vi "单通道IT01.vi"() -> ()   [LabVIEW 2020]
uses:
  <vilib>/Utility/miscctls.llb/LVPointTypeDef.ctl
  <vilib>/Utility/config.llb/Write Key (String).vi
  <vilib>/Utility/config.llb/Read Key (String).vi
  <vilib>/Utility/file.llb/Write Delimited Spreadsheet (string).vi
  <vilib>/Modbus/master/Modbus Master.lvclass
  <vilib>/Utility/config.llb/NI_LVConfig.lvlib
  LABVIEW.dll
  <vilib>/Modbus/master/Create Master Instance (Serial).vi
panel:
  in  "按钮":bool
  in  "文本下拉列表":u16(ring)=50 items=["30"=300, "35"=350, "40"=400, "45"=450, "50"=500, "55"=550, "60"=600, "65"=650, "70"=700, "75"=750, "80"=800]
  out "当前温度 2":dbl
  out "error out":errorcluster caption="错误输出"
  out "退出":bool
  out "保存所有":bool
  out "分析":bool
  out "配置":bool
  out "连接":bool
  in  "选项卡控件 3":enum32{"选项卡 2"}(tab)
  in  "开始连接":bool
  in  "搜索设备":bool
  in  "通讯方式选择":enum32{"USB", "ETHERNET", "RS485", "GPIB"}(radio)
  in  "表格":string[][](table)
  out "数组 2":refnum<vi>[](array[refnum])
  in  "通道选择":enum32{"ALL", "A1", "A2", "A3", "A4"}(radio)
  in  "测试项目":enum32{"EIS", "极化曲线", "耐久性曲线", "线性扫描"}(radio)
  in  "1":bool
  in  "测试项目 2":enum32{"极化曲线", "耐久性测试", "EIS"}(tab)
  in  "电源类型":u16(ring)
  in  "Ⅱ区测试点数:":i32
  in  "Ⅰ区测试点数:":dbl
  in  "膜面积(cm^2):":dbl
  in  "工步 2":i32(listbox)
  out "电流密度(A/cm^2):":dbl
  in  "测试时长(H):":dbl
  in  "施加电流(A):":dbl
  in  "有效膜面积(cm^2):":dbl
  in  "按钮 2":bool
  in  "VISA resource name 2":refnum<visa-resource-name>="COM3" caption="VISA resource name"
  in  "保存":bool
  in  "电解槽最大电压":dbl caption="电解槽最高温度设定："
  in  "循环水最差水质":dbl caption="冷却水最高温度："
  in  "水箱最低液位":dbl caption="冷却水最高温度："
  in  "氢气出口最大压力：":dbl caption="电解槽进口压力设定："
  in  "电解槽最高温度：":dbl caption="电解槽最高温度设定："
  in  "氢气最大露点：":dbl caption="氢气露点设定："
  in  "冷却水最高温度：":dbl
  in  "水箱补水液位：":dbl caption="水箱补水液位设定："
  in  "气液分离液位：":dbl caption="气液分离液位设定："
  in  "氢气出口背压设定：":dbl
  in  "水质换水":dbl caption="水质换水设定："
  in  "流量":T1(ring)
  in  "泵头":enum16{"YZ1515", "YZ2515", "KZ25", "YZ35"}(ring)
  in  "单选按钮":enum32{"正转", "反转"}(radio)
  in  "单选按钮 2":enum32{"四线", "二线"}(radio)
  in  "采样率":dbl
  in  "采样数":dbl
  in  "VISA resource name":refnum<visa-resource-name>="COM3"
  in  "温度25":u16(ring)=50 caption="文本下拉列表" items=["30"=300, "35"=350, "40"=400, "45"=450, "50"=500, "55"=550, "60"=600, "65"=650, "70"=700, "75"=750, "80"=800]
  in  "2":bool
  in  "3":bool
  in  "4":bool
  in  "通道选择 2":enum32{"未选择", "A1", "A2", "A3", "A4"}(radio)=enum."A1"
  out "报警信息":string
  out "当前电压":string
  out "当前电流":string
  in  "报警状态":bool
  in  "运行状态":bool
  out "当前温度":string
  out "通讯方式":string
  out "测试类型 2":string
  out "电压范围":string
  out "电流范围":string
  out "电源模式":string
  out "登录时间：":string
  out "用户：":string
  out "字符串 3":string
  out "队列输出 2":refnum<queue>
  in  "开始测量 4":bool caption="开始测量"
  in  "开始测量 3":bool caption="开始测量"
  in  "开始测量 2":bool caption="开始测量"
  in  "开始测量":bool
  in  "导出曲线":bool caption="历史曲线"
  in  "保存工步":bool
  in  "添加工步":bool
  in  "历史曲线":bool
  out "停止测试时间:":string
  out "开始测试时间:":string
  out "刷新":bool
  in  "重排所有视图":bool
  out "显示所有视图":bool
  out "流量 2":bool
  out "工步":bool
  out "压强":bool
  out "温度":bool
  out "电流/电压":bool
  in  "数组 12":string[][](array[string]) caption="数组"
  in  "数组 11":string[][](array[string]) caption="数组"
  in  "数组 10":string[][](array[string]) caption="数组"
  in  "数组":string[][](array[string])
  in  "压力3":string[][](array[string])
  in  "压力4":string[][](array[string])
  in  "压力2":string[][](array[string])
  in  "压力1":string[][](array[string])
  out "数值":i32
  in  "test":bool
  in  "水质4":string[][](array[string])
  in  "温度4":string[][](array[string])
  in  "水质3":string[][](array[string])
  in  "温度3":string[][](array[string])
  in  "水质2":string[][](array[string])
  in  "温度2":string[][](array[string])
  in  "温度显示 4":dbl
  in  "温度显示 3":dbl
  in  "温度显示 2":dbl
  in  "温度显示":dbl
  in  "所有数据4":string[][](array[string])
  in  "所有数据3":string[][](array[string])
  in  "所有数据2":string[][](array[string])
  in  "所有数据":string[][](array[string])
  out "数值 4":i32
  out "数值 3":i32
  out "数值 2":i32
  in  "极化曲线4":dbl[][](array[numeric])
  in  "极化电压4":dbl
  in  "极化电流4":dbl
  in  "电压4":dbl[](array[numeric])
  in  "电流4":dbl[](array[numeric])
  in  "极化曲线3":dbl[][](array[numeric])
  in  "极化电压3":dbl
  in  "极化电流3":dbl
  in  "电压3":dbl[](array[numeric])
  in  "电流3":dbl[](array[numeric])
  in  "极化曲线2":dbl[][](array[numeric])
  in  "极化电压2":dbl
  in  "极化电流2":dbl
  in  "电压2":dbl[](array[numeric])
  in  "电流2":dbl[](array[numeric])
  in  "极化曲线1":dbl[][](array[numeric])
  in  "极化电压1":dbl
  in  "极化电流1":dbl
  in  "电压1":dbl[](array[numeric])
  in  "电流1":dbl[](array[numeric])
  in  "水质1":string[][](array[string])
  in  "温度1":string[][](array[string])
  in  "选项卡控件 2":enum32{"选项卡 1", "选项卡 2", "选项卡 3"}(tab)
  in  "树形控件 2":string(tree)
  in  "撤销当前设置":bool
  in  "保存当前设置":bool
  in  "打开历史设置":bool
  out "数组 8":string[](array[string])
  in  "字符串":string
  out "数值 3":i32
  out "电流":dbl
  out "电压":dbl
  out "数据":string
  in  "数组 4":refnum<vi>[](array[refnum])
  in  "数组 5":refnum<vi>[](array[refnum])
  in  "数组 6":refnum<vi>[](array[refnum])
  in  "数组 7":refnum<vi>[](array[refnum])
  out "布尔":bool
  out "布尔 2":bool
  out "布尔 5":bool
  out "布尔 4":bool
  out "布尔 3":bool
  out "布尔 6":bool
  in  "数组 9":refnum<vi>[](array[refnum])
  in  "数组 3":refnum<vi>[](array[refnum])
  out "输出电磁阀":bool
  out "露点电磁阀":bool
  out "流量电磁阀":bool
  out "补水电磁阀":bool
  out "排水电磁阀":bool
  out "冷水控温阀":bool
  out "排尽电磁阀":bool
  out "冷却水温度过高报警":bool
  out "电堆超压报警":bool
  out "露点报警":bool
  out "电堆温度报警":bool
  out "积水报警":bool
  out "水质报警":bool
  out "水箱缺水报警":bool
  out "循环水温度报警":bool
  out "循环水流量报警":bool
  out "氢气出口超压报警":bool
  out "字符串 2":string
  # "设备列表"
  # "参数设置"
  # "测试设置"
  # "VISA"
  # "水温"
  # "℃"
  # "VISA"
  # "MPa"
  # "MΩ.cm"
  # "cm"
  # "cm"
  # "报警参数设置"
  # "℃"
  # "℃"
  # "V"
  # "℃"
  # "cm"
  # "MPa"
  # "MΩ.cm"
  # "工作设置"
  # "停机设置"
  # "工步设置"
  # "CH1"
  # "CH2"
  # "CH3"
  # "CH4"
  # "电磁阀状态"
  # "报警状态"
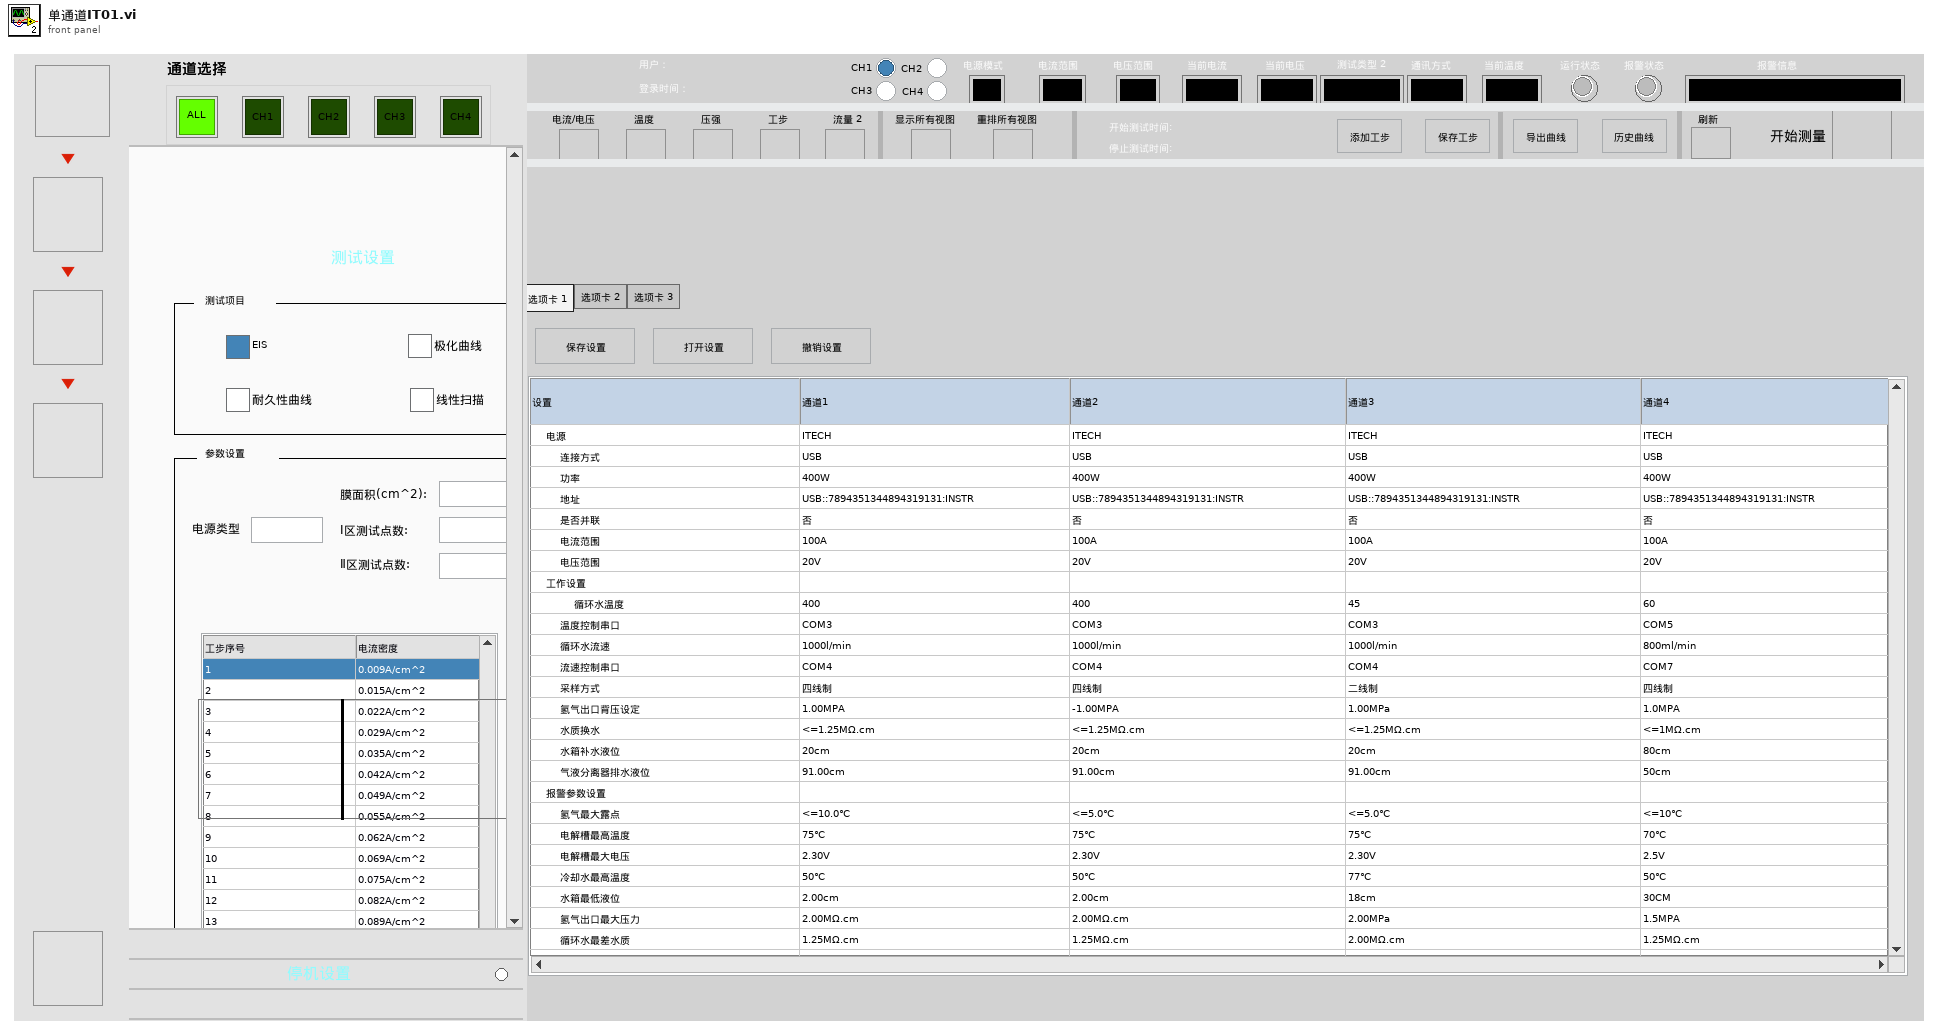
[diagram p1: front panel]
types:
  T1 = enum16{"200ml/min", "400lml/min", "600ml/min", "800ml/min", "1000ml/min", "1200ml/min", "1400ml/min", "1600ml/min"}
  T2 = enum8{"Enabled", "Disabled", "Disabled and Grayed Out"}
  T3 = enum16{"Always On", "Always Off", "Off While Running"}
  T4 = typedef "LVPointTypeDef.ctl" = cluster{"Horizontal":i16, "Vertical":i16}
  T5 = cluster{"温度1":refnum<vi>, "温度2":refnum<vi>, "温度3":refnum<vi>, "温度4":refnum<vi>}
  T6 = cluster{"水质1":refnum<vi>, "水质2":refnum<vi>, "水质3":refnum<vi>, "水质4":refnum<vi>}
  T7 = cluster{"极化曲线1":refnum<vi>, "极化曲线2":refnum<vi>, "极化曲线3":refnum<vi>, "极化曲线4":refnum<vi>}
  T8 = cluster{"电压1":refnum<vi>, "电压2":refnum<vi>, "电压3":refnum<vi>, "电压4":refnum<vi>}
  T9 = cluster{"电流1":refnum<vi>, "电流2":refnum<vi>, "电流3":refnum<vi>, "电流4":refnum<vi>}
  T10 = cluster{"压力1":refnum<vi>, "压力2":refnum<vi>, "压力3":refnum<vi>, "压力4":refnum<vi>}
  T11 = cluster{"所有数据":refnum<vi>, "数值":refnum<vi>, "极化曲线1":refnum<vi>, "极化电压1":refnum<vi>, "极化电流1":refnum<vi>, "电压1":refnum<vi>, "电流1":refnum<vi>, "水质1":refnum<vi>, "温度1":refnum<vi>, "温度显示":refnum<vi>, "压力1":refnum<vi>}
  T12 = cluster{"水质2":refnum<vi>, "温度2":refnum<vi>, "温度显示 2":refnum<vi>, "所有数据2":refnum<vi>, "数值 2":refnum<vi>, "极化曲线2":refnum<vi>, "极化电压2":refnum<vi>, "极化电流2":refnum<vi>, "电压2":refnum<vi>, "电流2":refnum<vi>, "压力2":refnum<vi>}
  T13 = cluster{"水质3":refnum<vi>, "温度3":refnum<vi>, "温度显示 3":refnum<vi>, "所有数据3":refnum<vi>, "数值 3":refnum<vi>, "极化曲线3":refnum<vi>, "极化电压3":refnum<vi>, "极化电流3":refnum<vi>, "电压3":refnum<vi>, "电流3":refnum<vi>, "压力3":refnum<vi>}
  T14 = cluster{"水质4":refnum<vi>, "温度4":refnum<vi>, "温度显示 4":refnum<vi>, "所有数据4":refnum<vi>, "数值 4":refnum<vi>, "极化曲线4":refnum<vi>, "极化电压4":refnum<vi>, "极化电流4":refnum<vi>, "电压4":refnum<vi>, "电流4":refnum<vi>, "压力4":refnum<vi>}
  T15 = enum32{"Invalid", "Standard", "Closed", "Hidden", "Minimized", "Maximized"}
  T16 = enum16{"open", "replace", "create", "open or create", "replace or create", "replace or create with confirmation"}
  T17 = typedef "NI_LVConfig.lvlib/Config Data RefNum.ctl" = refnum<k1>
  T18 = cluster{string, string[], string, i32, bool, i32}
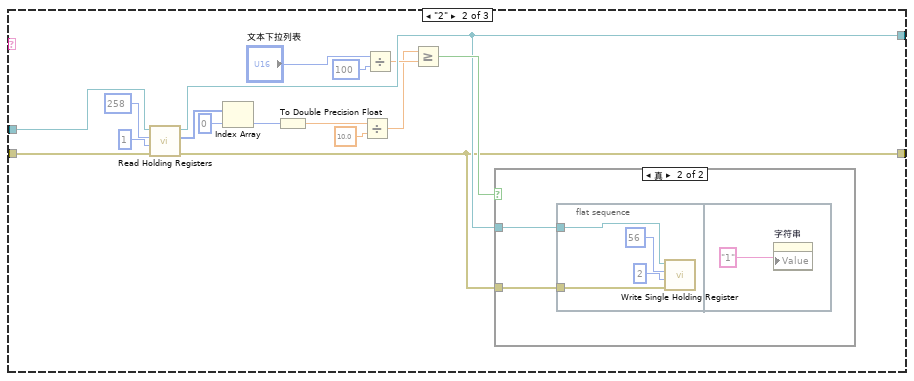
[diagram p2: hidden frame]
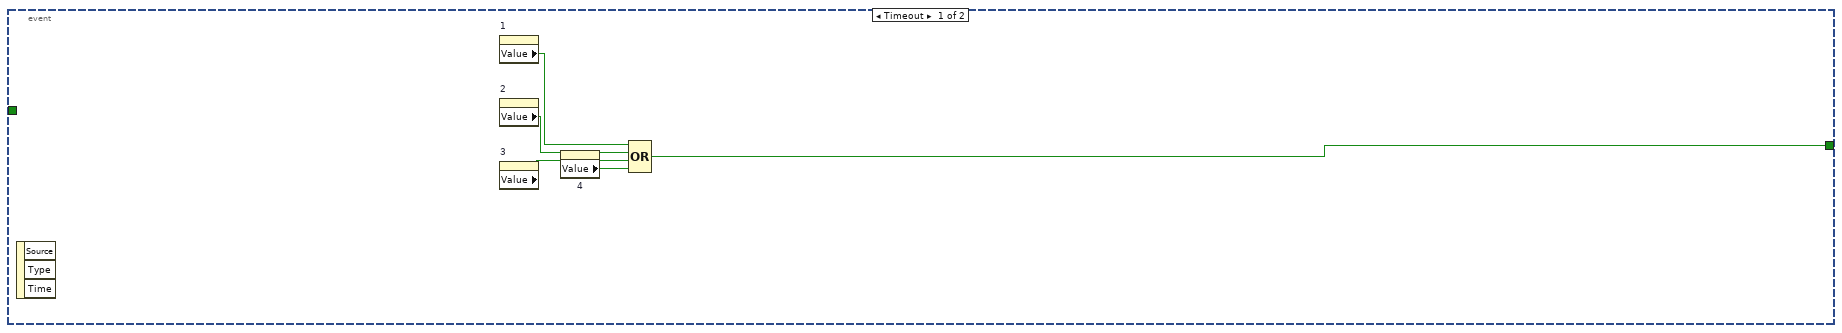
[diagram p6: hidden frame]
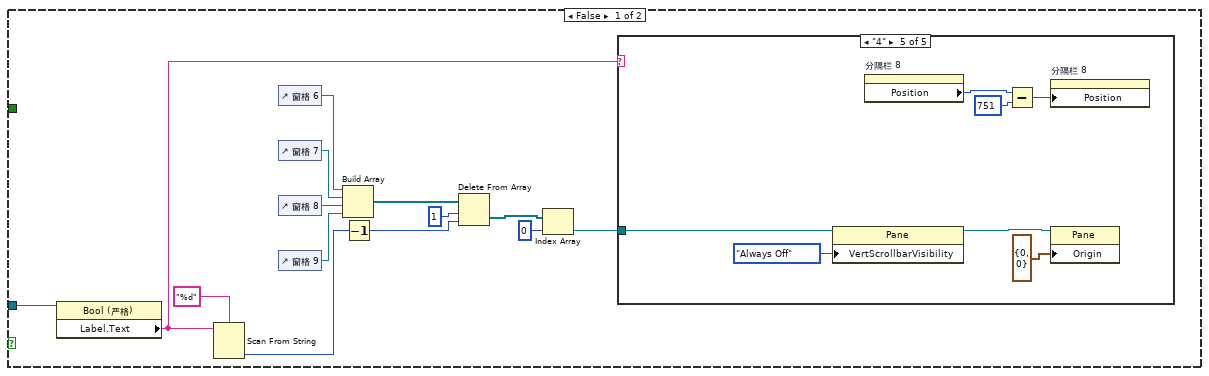
[diagram p7: hidden frame]
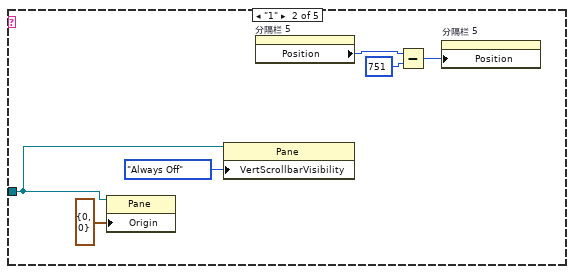
[diagram p9: hidden frame]
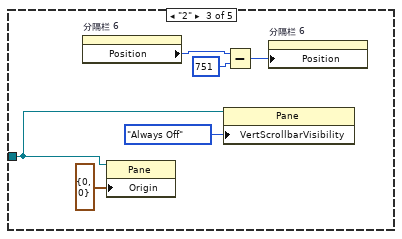
[diagram p10: hidden frame]
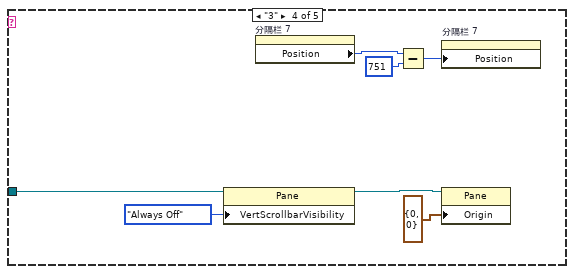
[diagram p11: hidden frame]
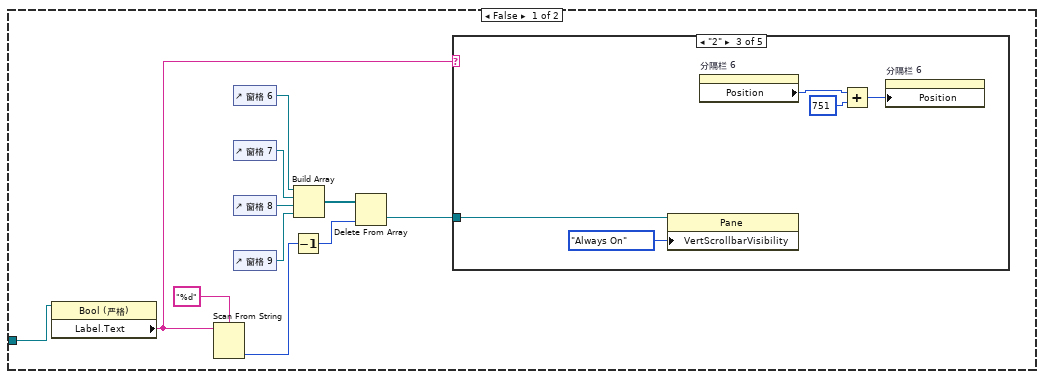
[diagram p12: hidden frame]
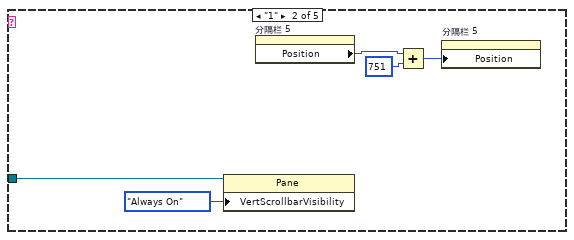
[diagram p14: hidden frame]
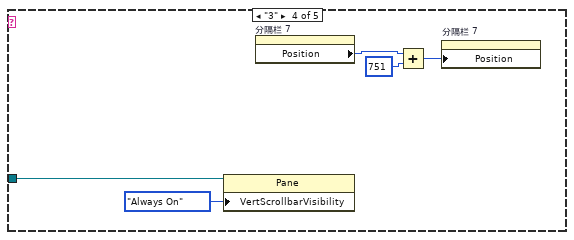
[diagram p15: hidden frame]
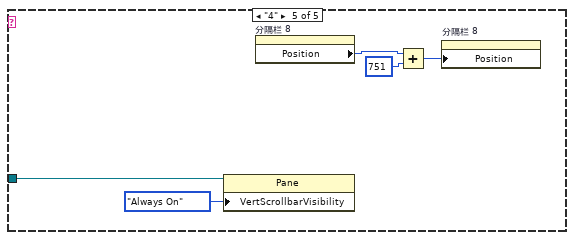
[diagram p16: hidden frame]
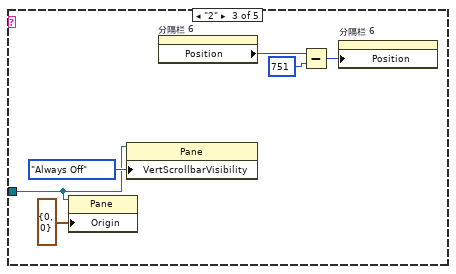
[diagram p19: hidden frame]
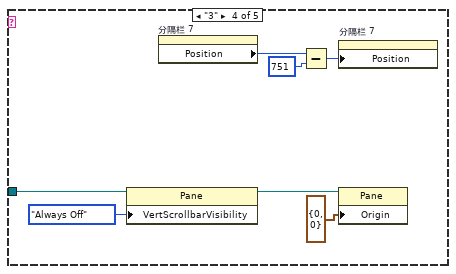
[diagram p20: hidden frame]
diagram:
  w20 = T2."Enabled" ("禁用")
  w10 = refnum<vi>[] [] ("数组 4")
  w64 = string[][] [] ("温度1")
  w65 = dbl[] [] ("电压1")
  (unwired) string[] ["循环水温度", "温度控制串口", "循环水流速", "流速控制串口", "采样方式", "氢气出口背压设定", "水质换水", "水箱补水液位", "气液分离器排水液位", "氢气最大露点", "电解槽最高温度", "电解槽最大电压", "冷却水最高温度", "水箱最低液位", "氢气出口最大压力", "循环水最差水质"]
  (unwired) TRUE ("运行时滚动到原点")
  w4 = string[][] []
  (unwired) TRUE ("布尔 17")
  (unwired) "添加工步"
  # "A2"
  # "USB0::0x2EC7::0x3000::803489033757710010::INSTR"
  # "a1"
  # "USB0::0x2EC7::0x3000::803489033757710011::INSTR"
  n1 = disable-structure shown="禁用" {
    frame Disabled {
      n2 = flat-sequence {
        frame #0 {
          w126 = "已完成" ("活动单元格:字符串")
          w127 = 8 ("活动单元格:活动列数")
          w130 = "A1" ("活动项:标识符")
          n3 = Add() -> (x=w129:dbl, x+y=w128:dbl)  [unwired: 1 in]
        }
        frame #1 {
          n4 = Index Array(array=w136, index (col)=0 ("禁用的索引 (列)")) -> (element=w134)  [unwired: 1 in]
          n5 = Search 1D Array(1D array=w134, element=" " ("元素")) -> (index of element=w132:i32)  [unwired: 1 in]
          n6 = Equal?(y=w132) -> (x = y?=w131:bool)  [unwired: 1 in]
          n7 = case shown="假" w131 {
            tunnel: [w142 _] -> w136
            frame False {
              w137 = u32 6618880
              w138 = "正在运行" ("活动单元格:字符串")
              w139 = 8 ("活动单元格:活动列数")
              w140 = "A1" ("活动项:标识符")
              w146 = 3 ("活动单元格:活动列数")
              w147 = "A1" ("活动项:标识符")
              w152 = 5 ("活动单元格:活动列数")
              w153 = "A1" ("活动项:标识符")
              w157 = 4 ("活动单元格:活动列数")
              w156 = "A1" ("活动项:标识符")
              w160 = 7 ("活动单元格:活动列数")
              w159 = "A1" ("活动项:标识符")
              n8 = Index Array(array=w142) -> (element=w149)  [unwired: 2 in]
              n9 = Increment() -> (x+1=w141:dbl)  [unwired: 1 in]
              n10 = Index Array(array=w149, index=3 ("索引")) -> (element=w150)
              n11 = Index Array(array=w149, index=2 ("索引")) -> (element=w154)
              n12 = Index Array(array=w149, index=5 ("索引")) -> (element=w158)
              n13 = Format Into String(w141) -> (resulting string=w144:string)  [unwired: 3 in, 1 out]
              n14 = Concatenate Strings("工步", w144) -> (w143:string)
            }
            frame True {
              w161 = "已完成" ("活动单元格:字符串")
              w162 = 8 ("活动单元格:活动列数")
              w163 = "A1" ("活动项:标识符")
            }
          }
        }
        frame #2 {
          n15 = case shown="真" {
            selector: _ -> [_ _]
            tunnel: [w165 w186] -> w164
            frame False {
              n16 = Index Array(array=w173) -> (element=w174, index=w175:i32)
              n17 = Unbundle(w174) -> (w168, w170)
              n18 = Build Array(w168) -> (w169:void[], w167)
              n19 = Build Array (concatenate)(w170) -> (w171:void[], w166:void[])
              n20 = Bundle(w169, w171) -> (w172:cluster{void[], void[]})  [unwired: 1 in]
              n21 = Replace Array Subset(new element=w172, index=w175) -> (array=w173:cluster{void[], void[]}[], w165:cluster{void[], void[]}[])
            }
            frame True {
              n22 = Array Size() -> (array=w181:dbl[], size(s)=w182:i32)
              n23 = Index Array(array=w181, index=w182) -> (element=w183)
              n24 = Unbundle(w183) -> (w180, w179)
              n25 = Build Array (concatenate)(w180) -> (w178:void[], w185:void[])
              n26 = Build Array (concatenate)(w179) -> (w177:void[], w184:void[])
              n27 = Bundle(w178, w177) -> (w176:cluster{void[], void[]})  [unwired: 1 in]
              n28 = Insert Into Array(array=w181, new element=w176) -> (w186:cluster{void[], void[]}[])  [unwired: 1 in]
            }
          }
        }
      }
    }
    frame Enabled {
    }
  }
  n29 = disable-structure shown="禁用" {
    frame Disabled {
      n30 = case shown="\"YZ35\"" {
        selector: _ -> [_ _ _ _]
        tunnel: ["YZ1515" "yz2515" "KZ25" "YZ35"] -> _
        frame "YZ1515", Default {
        }
        frame "YZ2515" {
        }
        frame "KZ25" {
        }
        frame "YZ35" {
        }
      }
    }
    frame Enabled {
    }
  }
  n31 = control-ref of="窗格 9"() -> (w100:refnum<vi>)
  n32 = property class="Pane"(reference=w100, "VertScrollbarVisibility"=T3."Always Off" ("垂直滚动条可见")) -> (error out=w98:errorcluster)  [unwired: 1 in, 1 out]
  n33 = property on="电压" class="DigNum (严格)"() -> ("Value"=w85:dbl)  [unwired: 2 in, 2 out]
  n34 = property on="电流" class="DigNum (严格)"() -> ("Value"=w82:dbl)  [unwired: 2 in, 2 out]
  n35 = Bundle By Name(cluster=cluster{"状态":bool, "错误码":i32, string} {"状态"=TRUE, "错误码"=0, ""} ("输入簇"), "状态"=TRUE, "错误码"=0) -> (w121:cluster{"状态":bool, "错误码":i32, string})
  n36 = Number To Fractional String(number=w82, precision (6)=i16 1 ("精度(6)")) -> (F-format string=→"当前电压":string)  [unwired: 2 in]
  n37 = Number To Fractional String(number=w85, precision (6)=i16 1 ("精度(6)")) -> (F-format string=→"当前电流":string)  [unwired: 2 in]
  n38 = flat-sequence {
    frame #0 {
      n39 = for {
        tunnel: i32[] [5, 6, 7] -> [w194] mode=indexing
        n40 = property on="窗格" class="Pane"() -> ("Decos[]"=w193:refnum<vi>[])  [unwired: 2 in, 2 out]
        n41 = Index Array(array=w193, index=w194) -> (element=w192:refnum<vi>)
        n42 = property class="Decor"(reference=w192, "Visible"=TRUE ("可见")) -> ()  [unwired: 1 in, 2 out]
      }
    }
    frame #1 {
      n43 = for {
        tunnel: i32[] [0, 1, 2, 3, 4] -> [w201] mode=indexing
        n44 = property on="窗格" class="Pane"() -> ("Decos[]"=w200:refnum<vi>[])  [unwired: 2 in, 2 out]
        n45 = Index Array(array=w200, index=w201) -> (element=w199:refnum<vi>)
        n46 = property class="Decor"(reference=w199, "Visible"=FALSE ("可见")) -> ()  [unwired: 1 in, 2 out]
      }
      n47 = property on="分隔栏 2" class="Splitter"("Position"=113 ("分隔栏位置")) -> ()  [unwired: 2 in, 2 out]
      n48 = property on="分隔栏 3" class="Splitter"("Position"=116 ("分隔栏位置")) -> ()  [unwired: 2 in, 2 out]
    }
    frame #2 {
      n49 = stacked-sequence {
        frame #0 {
          n50 = property on="分隔栏 4" class="Splitter"() -> ("Position"=w203:i32)  [unwired: 2 in, 2 out]
          n51 = Add(x=w203, y=32 ("分隔栏位置")) -> (x+y=w205:i32)
          n52 = property on="分隔栏 5" class="Splitter"("Position"=w205) -> ()  [unwired: 2 in, 2 out]
        }
        frame #1 {
          n53 = property on="分隔栏 4" class="Splitter"() -> ("Position"=w208:i32)  [unwired: 2 in, 2 out]
          n54 = Add(x=w208, y=62 ("分隔栏位置")) -> (x+y=w207:i32)
          n55 = property on="分隔栏 6" class="Splitter"("Position"=w207) -> ()  [unwired: 2 in, 2 out]
        }
        frame #2 {
          n56 = property on="分隔栏 4" class="Splitter"() -> ("Position"=w211:i32)  [unwired: 2 in, 2 out]
          n57 = Add(x=w211, y=92 ("分隔栏位置")) -> (x+y=w210:i32)
          n58 = property on="分隔栏 7" class="Splitter"("Position"=w210) -> ()  [unwired: 2 in, 2 out]
        }
        frame #3 {
          n59 = property on="分隔栏 4" class="Splitter"() -> ("Position"=w214:i32)  [unwired: 2 in, 2 out]
          n60 = Add(x=w214, y=122 ("分隔栏位置")) -> (x+y=w212:i32)
          n61 = property on="分隔栏 8" class="Splitter"("Position"=w212) -> ()  [unwired: 2 in, 2 out]
        }
      }
    }
  }
  n62 = property on="选项卡控件 2" class="TabCtl (严格)"("Value"=enum32{"选项卡 1", "选项卡 2", "选项卡 3"}."选项卡 1" ("选项卡控件 2")) -> (error out=w7:errorcluster)  [unwired: 2 in, 1 out]
  n63 = Obtain Queue(name (unnamed)="数据处理队列" ("名称（未命名）"), element data type=w121, create if not found? (T)=TRUE ("如未找到则创建？(T)")) -> (queue out=w119:refnum<queue>)  [unwired: 2 in, 2 out]
  "队列输出 2" <- w119
  n64 = property on="4" class="Bool (严格)"(error in=w98, "Value"=FALSE ("3 2")) -> (error out=w101:errorcluster)  [unwired: 1 in, 1 out]
  n65 = property on="重排所有视图" class="Bool (严格)"(error in=w7, "Value"=TRUE ("重排所有视图")) -> (error out=w32:errorcluster)  [unwired: 1 in, 1 out]
  n66 = control-ref of="水质1"() -> ()  [unwired: 1 out]
  n67 = control-ref of="水质2"() -> ()  [unwired: 1 out]
  n68 = control-ref of="水质3"() -> ()  [unwired: 1 out]
  n69 = control-ref of="水质4"() -> ()  [unwired: 1 out]
  n70 = property on="1" class="Bool (严格)"(error in=w101, "Value"=FALSE ("1")) -> (error out=w113:errorcluster)  [unwired: 1 in, 1 out]
  n71 = while {
    tunnel: w119 -> [w216]
    tunnel: [w215] -> w118
    stop <- FALSE stop-if-true
    n72 = event shown="[0] 超时" {
      selector: _ -> [_]
      dyn-events: _ -> [_]
      timeout: 100 -> [_]
      tunnel: w216 -> [w225]
      tunnel: [w222] -> w215
      event Timeout {
        n73 = event-data() -> ()  [unwired: 1 in, 3 out]
        n74 = Dequeue Element(queue=w225, timeout in ms (-1)=-1 ("超时毫秒(-1)")) -> (queue out=w222:refnum<queue>, element=w223:cluster{"状态":bool, "错误码":i32, string})  [unwired: 1 in, 2 out]
        n75 = Unbundle(w223) -> ("状态"=w219:bool, "错误码"=w220:i32, w221:string)
        n76 = case shown="真" w219 {
          tunnel: w221 -> [_ w231]
          tunnel: w220 -> [_ w229]
          frame False {
          }
          frame True {
            n77 = Format Into String(w229) -> (resulting string=w228:string)  [unwired: 3 in, 1 out]
            n78 = Concatenate Strings(w231, "错误：" ("字符串"), w228) -> (w227:string)
            n79 = One Button Dialog(message=w227, button name ("OK")="确定" ("按钮名称（“确定”）")) -> ()  [unwired: 1 out]
          }
        }
      }
    }
  }
  n80 = property on="2" class="Bool (严格)"(error in=w113, "Value"=FALSE ("2")) -> (error out=w112:errorcluster)  [unwired: 1 in, 1 out]
  n81 = property on="通道选择 2" class="RadioBtnsControl (严格)"(error in=w32, "Value"=enum32{"未选择", "A1", "A2", "A3", "A4"}."A1" ("通道选择 2")) -> (error out=w26:errorcluster)  [unwired: 1 in, 1 out]
  n82 = property on="通道选择" class="RadioBtnsControl (严格)"(error in=w26, "Value"=enum32{"ALL", "A1", "A2", "A3", "A4"}."ALL" ("通道选择")) -> (error out=w24:errorcluster)  [unwired: 1 in, 1 out]
  n83 = property on="3" class="Bool (严格)"(error in=w112, "Value"=FALSE ("3")) -> (error out=w109:errorcluster)  [unwired: 1 in, 1 out]
  n84 = property on="测试项目" class="RadioBtnsControl (严格)"(error in=w24, "Value"=enum32{"EIS", "极化曲线", "耐久性曲线", "线性扫描"}."极化曲线" ("测试项目：")) -> (error out=w22:errorcluster)  [unwired: 1 in, 1 out]
  n85 = control-ref of="窗格 6"() -> (w111:refnum<vi>)
  n86 = property on="测试项目 2" class="TabCtl (严格)"(error in=w22, "Value"=enum32{"极化曲线", "耐久性测试", "EIS"}."极化曲线" ("测试项目 2")) -> (error out=w21:errorcluster)  [unwired: 1 in, 1 out]
  n87 = property on="数组 3" class="Arr (严格)"(error in=w21, "Value"=refnum<vi>[] [] ("数组 3")) -> (error out=w96:errorcluster)  [unwired: 1 in, 1 out]
  n88 = property on="数组" class="Arr (严格)"(error in=w96, "Value"=w4) -> (error out=w5:errorcluster)  [unwired: 1 in, 1 out]
  n89 = property on="数组 10" class="Arr (严格)"(error in=w5, "Value"=w4) -> (error out=w2:errorcluster)  [unwired: 1 in, 1 out]
  n90 = property on="数组 11" class="Arr (严格)"(error in=w2, "Value"=w4) -> (error out=w3:errorcluster)  [unwired: 1 in, 1 out]
  n91 = property on="数组 12" class="Arr (严格)"(error in=w3, "Value"=w4) -> (error out=w1:errorcluster)  [unwired: 1 in, 1 out]
  n92 = property class="Pane"(reference=w111, error in=w109, "VertScrollbarVisibility"=T3."Always Off" ("垂直滚动条可见")) -> (error out=w106:errorcluster)  [unwired: 1 out]
  n93 = property on="数组 2" class="Arr (严格)"(error in=w1, "Value"=refnum<vi>[] [] ("数组 2")) -> (error out=w34:errorcluster)  [unwired: 1 in, 1 out]
  n94 = Release Queue(queue=w118) -> ()  [unwired: 2 in, 3 out]
  n95 = control-ref of="窗格 7"() -> (w107:refnum<vi>)
  n96 = property on="数组 4" class="Arr (严格)"(error in=w34, "Value"=refnum<vi>[] [] ("数组 4")) -> (error out=w19:errorcluster)  [unwired: 1 in, 1 out]
  n97 = property on="分析" class="Bool (严格)"(error in=w19, "DisabledEnum"=w20) -> (error out=w18:errorcluster)  [unwired: 1 in, 1 out]
  n98 = property on="保存所有" class="Bool (严格)"(error in=w18, "DisabledEnum"=w20) -> (error out=w17:errorcluster)  [unwired: 1 in, 1 out]
  n99 = property on="连接" class="Bool (严格)"(error in=w17, "DisabledEnum"=w20) -> (error out=w16:errorcluster)  [unwired: 1 in, 1 out]
  n100 = property on="配置" class="Bool (严格)"(error in=w16, "DisabledEnum"=w20) -> (error out=w15:errorcluster)  [unwired: 1 in, 1 out]
  n101 = property class="Pane"(reference=w107, error in=w106, "VertScrollbarVisibility"=T3."Always Off" ("垂直滚动条可见")) -> (error out=w103:errorcluster)  [unwired: 1 out]
  n102 = property on="通道选择" class="RadioBtnsControl (严格)"(error in=w15, "DisabledEnum"=w20) -> (error out=w14:errorcluster)  [unwired: 1 in, 1 out]
  n103 = property on="2" class="Bool (严格)"(error in=w14, "DisabledEnum"=w20) -> (error out=w13:errorcluster)  [unwired: 1 in, 1 out]
  n104 = property on="3" class="Bool (严格)"(error in=w13, "DisabledEnum"=w20) -> (error out=w12:errorcluster)  [unwired: 1 in, 1 out]
  n105 = property on="4" class="Bool (严格)"(error in=w12, "DisabledEnum"=w20) -> (error out=w11:errorcluster)  [unwired: 1 in, 1 out]
  n106 = property on="数值" class="DigNum (严格)"("Value"=0.0 ("数值")) -> (error out=w54:errorcluster)  [unwired: 2 in, 1 out]
  n107 = property on="温度1" class="Arr (严格)"(error in=w54, "Value"=string[][] [] ("温度1")) -> (error out=w73:errorcluster)  [unwired: 1 in, 1 out]
  n108 = property on="水质1" class="Arr (严格)"(error in=w73, "Value"=string[][] [] ("温度1")) -> (error out=w72:errorcluster)  [unwired: 1 in, 1 out]
  n109 = property on="所有数据" class="Arr (严格)"(error in=w72, "Value"=string[][] [] ("温度1")) -> (error out=w70:errorcluster)  [unwired: 1 in, 1 out]
  n110 = property on="极化曲线1" class="Arr (严格)"(error in=w70, "Value"=dbl[][] [] ("极化曲线1")) -> (error out=w69:errorcluster)  [unwired: 1 in, 1 out]
  n111 = property on="数组 5" class="Arr (严格)"(error in=w11, "Value"=refnum<vi>[] [] ("数组 4")) -> (error out=w31:errorcluster)  [unwired: 1 in, 1 out]
  n112 = property on="数组 6" class="Arr (严格)"(error in=w31, "Value"=refnum<vi>[] [] ("数组 4")) -> (error out=w30:errorcluster)  [unwired: 1 in, 1 out]
  n113 = property on="数组 7" class="Arr (严格)"(error in=w30, "Value"=w10) -> (error out=w9:errorcluster)  [unwired: 1 in, 1 out]
  n114 = property on="数组 9" class="Arr (严格)"(error in=w9, "Value"=w10) -> (error out=w8:errorcluster)  [unwired: 1 in, 1 out]
  n115 = property on="开始测量" class="Bool (严格)"(error in=w8, "Visible"=TRUE ("可见")) -> (error out=w47:errorcluster)  [unwired: 1 in, 1 out]
  n116 = property on="开始测量 2" class="Bool (严格)"(error in=w47, "Visible"=FALSE ("可见")) -> (error out=w46:errorcluster)  [unwired: 1 in, 1 out]
  n117 = property on="开始测量 3" class="Bool (严格)"(error in=w46, "Visible"=FALSE ("可见")) -> (error out=w45:errorcluster)  [unwired: 1 in, 1 out]
  n118 = property on="开始测量 4" class="Bool (严格)"(error in=w45, "Visible"=FALSE ("可见")) -> (error out=w44:errorcluster)  [unwired: 1 in, 1 out]
  n119 = property on="数值 2" class="DigNum (严格)"("Value"=0 ("数值 2")) -> ()  [unwired: 2 in, 2 out]
  n120 = property on="电流1" class="Arr (严格)"(error in=w69, "Value"=dbl[] [] ("电压1")) -> (error out=w68:errorcluster)  [unwired: 1 in, 1 out]
  n121 = property on="电压1" class="Arr (严格)"(error in=w68, "Value"=dbl[] [] ("电压1")) -> (error out=w62:errorcluster)  [unwired: 1 in, 1 out]
  n122 = property on="电压2" class="Arr (严格)"(error in=w62, "Value"=w65) -> (error out=w61:errorcluster)  [unwired: 1 in, 1 out]
  n123 = property on="电流2" class="Arr (严格)"(error in=w61, "Value"=w65) -> (error out=w60:errorcluster)  [unwired: 1 in, 1 out]
  n124 = property on="水质2" class="Arr (严格)"(error in=w60, "Value"=w64) -> (error out=w59:errorcluster)  [unwired: 1 in, 1 out]
  n125 = property on="温度2" class="Arr (严格)"(error in=w59, "Value"=w64) -> (error out=w58:errorcluster)  [unwired: 1 in, 1 out]
  n126 = property on="所有数据2" class="Arr (严格)"(error in=w58, "Value"=w64) -> (error out=w57:errorcluster)  [unwired: 1 in, 1 out]
  n127 = property on="极化曲线2" class="Arr (严格)"(error in=w57, "Value"=dbl[][] [] ("极化曲线1")) -> (error out=w56:errorcluster)  [unwired: 1 in, 1 out]
  n128 = control-ref of="窗格 8"() -> (w104:refnum<vi>)
  n129 = property on="开始测量" class="Bool (严格)"(error in=w44, "Value"=FALSE ("开始测量")) -> (error out=w42:errorcluster)  [unwired: 1 in, 1 out]
  n130 = property on="开始测量 2" class="Bool (严格)"(error in=w42, "Value"=FALSE ("开始测量 2")) -> (error out=w40:errorcluster)  [unwired: 1 in, 1 out]
  n131 = property on="开始测量 3" class="Bool (严格)"(error in=w40, "Value"=FALSE ("开始测量 3")) -> (error out=w38:errorcluster)  [unwired: 1 in, 1 out]
  n132 = property on="开始测量 4" class="Bool (严格)"(error in=w38, "Value"=FALSE ("开始测量 4")) -> (error out=w36:errorcluster)  [unwired: 1 in, 1 out]
  n133 = property class="Pane"(reference=w104, error in=w103, "VertScrollbarVisibility"=T3."Always Off" ("垂直滚动条可见")) -> (error out=w79:errorcluster)  [unwired: 1 out]
  n134 = while {
    shift-right: [w233] -> _
    shift-left: FALSE -> [w232]
    tunnel: w79 -> [_]
    stop <- FALSE stop-if-true
    n135 = event shown="[1] \"1\", \"2\", \"3\", \"4\": 值改变" {
      selector: _ -> [_ _]
      dyn-events: _ -> [_ _]
      timeout: 100 -> [_ _]
      tunnel: [w236 w241] -> w233
      tunnel: w232 -> [_ w242]
      event Timeout {
        n136 = event-data() -> ()  [unwired: 1 in, 3 out]
        n137 = property on="1" class="Bool (严格)"() -> ("Value"=w240:bool)  [unwired: 2 in, 2 out]
        n138 = property on="2" class="Bool (严格)"() -> ("Value"=w239:bool)  [unwired: 2 in, 2 out]
        n139 = property on="3" class="Bool (严格)"() -> ("Value"=w238:bool)  [unwired: 2 in, 2 out]
        n140 = property on="4" class="Bool (严格)"() -> ("Value"=w237:bool)  [unwired: 2 in, 2 out]
        n141 = Compound Arithmetic op=OR ("复合运算")(w240, w239, w238, w237) -> (w236:bool)
      }
      event "1", "2", "3", "4": Value Change {
        n142 = event-data() -> ("CtlRef"=w244:refnum<vi>, "NewVal"=w243:bool)  [unwired: 1 in, 4 out]
        n143 = case shown="真" w243 {
          tunnel: w244 -> [w246 w286]
          tunnel: w242 -> [_ w285]
          tunnel: [_ w285] -> w241
          frame False {
            n144 = property class="Bool (严格)"(reference=w246) -> ("Label.Text"=w245:string)  [unwired: 1 in, 2 out]
            n145 = Scan From String(format string="%d" ("格式字符串"), input string=w245) -> (output 1=w247:i32)  [unwired: 3 in, 3 out]
            n146 = control-ref of="窗格 6"() -> (w251:refnum<vi>)
            n147 = control-ref of="窗格 7"() -> (w250:refnum<vi>)
            n148 = control-ref of="窗格 8"() -> (w249:refnum<vi>)
            n149 = control-ref of="窗格 9"() -> (w258:refnum<vi>)
            n150 = Build Array(w251, w250, w249, w258) -> (w248:refnum<vi>[])
            n151 = Decrement(x=w247) -> (x-1=w252:i32)
            n152 = Delete From Array(array=w248, length=1 ("长度"), index=w252) -> (deleted portion=w255:refnum<vi>[])  [unwired: 1 out]
            n153 = Index Array(array=w255, index=0 ("索引")) -> (element=w257:refnum<vi>)
            n154 = case shown="\"4\"" w245 {
              tunnel: w257 -> [_ w260 w265 w272 w281]
              frame "假", Default {
              }
              frame "1" {
                n155 = property class="Pane"(reference=w260, "Origin"=T4 {"Horizontal"=0, "Vertical"=0} ("原点")) -> ()  [unwired: 1 in, 2 out]
                n156 = property class="Pane"(reference=w260, "VertScrollbarVisibility"=T3."Always Off" ("垂直滚动条可见")) -> ()  [unwired: 1 in, 2 out]
                n157 = property on="分隔栏 5" class="Splitter"() -> ("Position"=w263:i32)  [unwired: 2 in, 2 out]
                n158 = Subtract(x=w263, y=751) -> (x-y=w264:i32)
                n159 = property on="分隔栏 5" class="Splitter"("Position"=w264) -> ()  [unwired: 2 in, 2 out]
              }
              frame "2" {
                n160 = property on="分隔栏 6" class="Splitter"() -> ("Position"=w269:i32)  [unwired: 2 in, 2 out]
                n161 = property class="Pane"(reference=w265, "Origin"=T4 {"Horizontal"=0, "Vertical"=0} ("原点")) -> ()  [unwired: 1 in, 2 out]
                n162 = property class="Pane"(reference=w265, "VertScrollbarVisibility"=T3."Always Off" ("垂直滚动条可见")) -> ()  [unwired: 1 in, 2 out]
                n163 = Subtract(x=w269, y=751) -> (x-y=w270:i32)
                n164 = property on="分隔栏 6" class="Splitter"("Position"=w270) -> ()  [unwired: 2 in, 2 out]
              }
              frame "3" {
                n165 = property class="Pane"(reference=w272, "VertScrollbarVisibility"=T3."Always Off" ("垂直滚动条可见")) -> (reference out=w271:refnum<vi>)  [unwired: 1 in, 1 out]
                n166 = property on="分隔栏 7" class="Splitter"() -> ("Position"=w276:i32)  [unwired: 2 in, 2 out]
                n167 = Subtract(x=w276, y=751) -> (x-y=w275:i32)
                n168 = property on="分隔栏 7" class="Splitter"("Position"=w275) -> ()  [unwired: 2 in, 2 out]
                n169 = property class="Pane"(reference=w271, "Origin"=T4 {"Horizontal"=0, "Vertical"=0} ("原点")) -> ()  [unwired: 1 in, 2 out]
              }
              frame "4" {
                n170 = property class="Pane"(reference=w281, "VertScrollbarVisibility"=T3."Always Off" ("垂直滚动条可见")) -> (reference out=w280:refnum<vi>)  [unwired: 1 in, 1 out]
                n171 = property on="分隔栏 8" class="Splitter"() -> ("Position"=w279:i32)  [unwired: 2 in, 2 out]
                n172 = Subtract(x=w279, y=751) -> (x-y=w278:i32)
                n173 = property on="分隔栏 8" class="Splitter"("Position"=w278) -> ()  [unwired: 2 in, 2 out]
                n174 = property class="Pane"(reference=w280, "Origin"=T4 {"Horizontal"=0, "Vertical"=0} ("原点")) -> ()  [unwired: 1 in, 2 out]
              }
            }
          }
          frame True {
            n175 = case shown="真" w285 {
              tunnel: w286 -> [w297 w318]
              frame False {
                n176 = property class="Bool (严格)"(reference=w297) -> ("Label.Text"=w292:string)  [unwired: 1 in, 2 out]
                n177 = Scan From String(format string="%d" ("格式字符串"), input string=w292) -> (output 1=w290:i32)  [unwired: 3 in, 3 out]
                n178 = control-ref of="窗格 6"() -> (w295:refnum<vi>)
                n179 = control-ref of="窗格 7"() -> (w294:refnum<vi>)
                n180 = control-ref of="窗格 8"() -> (w293:refnum<vi>)
                n181 = control-ref of="窗格 9"() -> (w296:refnum<vi>)
                n182 = Decrement(x=w290) -> (x-1=w289:i32)
                n183 = Build Array(w295, w294, w293, w296) -> (w288:refnum<vi>[])
                n184 = Delete From Array(array=w288, index=w289) -> (deleted portion=w287:refnum<vi>)  [unwired: 1 in, 1 out]
                n185 = case shown="\"2\"" w292 {
                  tunnel: w287 -> [_ w299 w303 w308 w315]
                  frame "假", Default {
                  }
                  frame "1" {
                    n186 = property class="Pane"(reference=w299, "VertScrollbarVisibility"=T3."Always On" ("垂直滚动条可见")) -> ()  [unwired: 1 in, 2 out]
                    n187 = property on="分隔栏 5" class="Splitter"() -> ("Position"=w301:i32)  [unwired: 2 in, 2 out]
                    n188 = Add(x=w301, y=751) -> (x+y=w302:i32)
                    n189 = property on="分隔栏 5" class="Splitter"("Position"=w302) -> ()  [unwired: 2 in, 2 out]
                  }
                  frame "2" {
                    n190 = property class="Pane"(reference=w303, "VertScrollbarVisibility"=T3."Always On" ("垂直滚动条可见")) -> ()  [unwired: 1 in, 2 out]
                    n191 = property on="分隔栏 6" class="Splitter"() -> ("Position"=w306:i32)  [unwired: 2 in, 2 out]
                    n192 = Add(x=w306, y=751) -> (x+y=w307:i32)
                    n193 = property on="分隔栏 6" class="Splitter"("Position"=w307) -> ()  [unwired: 2 in, 2 out]
                  }
                  frame "3" {
                    n194 = property class="Pane"(reference=w308, "VertScrollbarVisibility"=T3."Always On" ("垂直滚动条可见")) -> ()  [unwired: 1 in, 2 out]
                    n195 = property on="分隔栏 7" class="Splitter"() -> ("Position"=w311:i32)  [unwired: 2 in, 2 out]
                    n196 = Add(x=w311, y=751) -> (x+y=w310:i32)
                    n197 = property on="分隔栏 7" class="Splitter"("Position"=w310) -> ()  [unwired: 2 in, 2 out]
                  }
                  frame "4" {
                    n198 = property class="Pane"(reference=w315, "VertScrollbarVisibility"=T3."Always On" ("垂直滚动条可见")) -> ()  [unwired: 1 in, 2 out]
                    n199 = property on="分隔栏 8" class="Splitter"() -> ("Position"=w314:i32)  [unwired: 2 in, 2 out]
                    n200 = Add(x=w314, y=751) -> (x+y=w313:i32)
                    n201 = property on="分隔栏 8" class="Splitter"("Position"=w313) -> ()  [unwired: 2 in, 2 out]
                  }
                }
              }
              frame True {
                n202 = stacked-sequence {
                  tunnel: w318 -> [w326 _]
                  tunnel: w318 -> [_ w376]
                  frame #0 {
                    n203 = control-ref of="1"() -> (w327:refnum<vi>)
                    n204 = control-ref of="2"() -> (w328:refnum<vi>)
                    n205 = control-ref of="3"() -> (w329:refnum<vi>)
                    n206 = control-ref of="4"() -> (w330:refnum<vi>)
                    n207 = property class="Bool (严格)"(reference=w326) -> ("Label.Text"=w325:string)  [unwired: 1 in, 2 out]
                    n208 = Scan From String(format string="%d" ("格式字符串"), input string=w325) -> (output 1=w323:i32)  [unwired: 3 in, 3 out]
                    n209 = Build Array(w327, w328, w329, w330) -> (w320:refnum<vi>[])
                    n210 = Decrement(x=w323) -> (x-1=w322:i32)
                    n211 = Delete From Array(array=w320, length=1 ("长度"), index=w322) -> (array with subset deleted=w319:refnum<vi>[])  [unwired: 1 out]
                    n212 = for {
                      tunnel: w319 -> [w332] mode=indexing
                      n213 = property class="Bool (严格)"(reference=w332) -> ("Value"=w331:bool)  [unwired: 1 in, 2 out]
                      n214 = Equal?(x=w331, y=TRUE) -> (x = y?=w333:bool)
                      n215 = case shown="真" w333 {
                        tunnel: w332 -> [_ w336]
                        frame False {
                        }
                        frame True {
                          n216 = property class="Bool (严格)"(reference=w336) -> ("Label.Text"=w340:string)  [unwired: 1 in, 2 out]
                          n217 = property class="Bool (严格)"(reference=w336, "Value"=FALSE ("值")) -> ()  [unwired: 1 in, 2 out]
                          n218 = Scan From String(format string="%d" ("格式字符串"), input string=w340) -> (output 1=w335:i32)  [unwired: 3 in, 3 out]
                          n219 = control-ref of="窗格 6"() -> (w344:refnum<vi>)
                          n220 = control-ref of="窗格 7"() -> (w343:refnum<vi>)
                          n221 = control-ref of="窗格 8"() -> (w342:refnum<vi>)
                          n222 = control-ref of="窗格 9"() -> (w348:refnum<vi>)
                          n223 = Decrement(x=w335) -> (x-1=w345:i32)
                          n224 = Build Array(w344, w343, w342, w348) -> (w341:refnum<vi>[])
                          n225 = Delete From Array(array=w341, length=1 ("长度"), index=w345) -> (deleted portion=w346:refnum<vi>[])  [unwired: 1 out]
                          n226 = Index Array(array=w346, index=0 ("索引")) -> (element=w347:refnum<vi>)
                          n227 = case shown="\"1\"" w340 {
                            tunnel: w347 -> [_ w351 w356 w363 w372]
                            frame "假", Default {
                            }
                            frame "1" {
                              n228 = property class="Pane"(reference=w351, "Origin"=T4 {"Horizontal"=0, "Vertical"=0} ("原点")) -> ()  [unwired: 1 in, 2 out]
                              n229 = property class="Pane"(reference=w351, "VertScrollbarVisibility"=T3."Always Off" ("垂直滚动条可见")) -> ()  [unwired: 1 in, 2 out]
                              n230 = property on="分隔栏 5" class="Splitter"() -> ("Position"=w354:i32)  [unwired: 2 in, 2 out]
                              n231 = Subtract(x=w354, y=751) -> (x-y=w355:i32)
                              n232 = property on="分隔栏 5" class="Splitter"("Position"=w355) -> ()  [unwired: 2 in, 2 out]
                            }
                            frame "2" {
                              n233 = property class="Pane"(reference=w356, "Origin"=T4 {"Horizontal"=0, "Vertical"=0} ("原点")) -> ()  [unwired: 1 in, 2 out]
                              n234 = property class="Pane"(reference=w356, "VertScrollbarVisibility"=T3."Always Off" ("垂直滚动条可见")) -> ()  [unwired: 1 in, 2 out]
                              n235 = property on="分隔栏 6" class="Splitter"() -> ("Position"=w360:i32)  [unwired: 2 in, 2 out]
                              n236 = Subtract(x=w360, y=751) -> (x-y=w361:i32)
                              n237 = property on="分隔栏 6" class="Splitter"("Position"=w361) -> ()  [unwired: 2 in, 2 out]
                            }
                            frame "3" {
                              n238 = property class="Pane"(reference=w363, "VertScrollbarVisibility"=T3."Always Off" ("垂直滚动条可见")) -> (reference out=w362:refnum<vi>)  [unwired: 1 in, 1 out]
                              n239 = property on="分隔栏 7" class="Splitter"() -> ("Position"=w367:i32)  [unwired: 2 in, 2 out]
                              n240 = Subtract(x=w367, y=751) -> (x-y=w366:i32)
                              n241 = property on="分隔栏 7" class="Splitter"("Position"=w366) -> ()  [unwired: 2 in, 2 out]
                              n242 = property class="Pane"(reference=w362, "Origin"=T4 {"Horizontal"=0, "Vertical"=0} ("原点")) -> ()  [unwired: 1 in, 2 out]
                            }
                            frame "4" {
                              n243 = property class="Pane"(reference=w372, "VertScrollbarVisibility"=T3."Always Off" ("垂直滚动条可见")) -> (reference out=w371:refnum<vi>)  [unwired: 1 in, 1 out]
                              n244 = property on="分隔栏 8" class="Splitter"() -> ("Position"=w370:i32)  [unwired: 2 in, 2 out]
                              n245 = Subtract(x=w370, y=751) -> (x-y=w369:i32)
                              n246 = property on="分隔栏 8" class="Splitter"("Position"=w369) -> ()  [unwired: 2 in, 2 out]
                              n247 = property class="Pane"(reference=w371, "Origin"=T4 {"Horizontal"=0, "Vertical"=0} ("原点")) -> ()  [unwired: 1 in, 2 out]
                            }
                          }
                        }
                      }
                    }
                  }
                  frame #1 {
                    n248 = property class="Bool (严格)"(reference=w376) -> ("Label.Text"=w382:string)  [unwired: 1 in, 2 out]
                    n249 = Scan From String(format string="%d" ("格式字符串"), input string=w382) -> (output 1=w381:i32)  [unwired: 3 in, 3 out]
                    n250 = control-ref of="窗格 6"() -> (w385:refnum<vi>)
                    n251 = control-ref of="窗格 7"() -> (w384:refnum<vi>)
                    n252 = control-ref of="窗格 8"() -> (w383:refnum<vi>)
                    n253 = control-ref of="窗格 9"() -> (w386:refnum<vi>)
                    n254 = Decrement(x=w381) -> (x-1=w380:i32)
                    n255 = Build Array(w385, w384, w383, w386) -> (w379:refnum<vi>[])
                    n256 = Delete From Array(array=w379, index=w380) -> (deleted portion=w378:refnum<vi>)  [unwired: 1 in, 1 out]
                    n257 = case shown="\"4\"" w382 {
                      tunnel: w378 -> [_ w388 w392 w397 w404]
                      frame "假", Default {
                      }
                      frame "1" {
                        n258 = property on="分隔栏 5" class="Splitter"() -> ("Position"=w390:i32)  [unwired: 2 in, 2 out]
                        n259 = property class="Pane"(reference=w388, "VertScrollbarVisibility"=T3."Always On" ("垂直滚动条可见")) -> ()  [unwired: 1 in, 2 out]
                        n260 = Add(x=w390, y=751) -> (x+y=w391:i32)
                        n261 = property on="分隔栏 5" class="Splitter"("Position"=w391) -> ()  [unwired: 2 in, 2 out]
                      }
                      frame "2" {
                        n262 = property on="分隔栏 6" class="Splitter"() -> ("Position"=w395:i32)  [unwired: 2 in, 2 out]
                        n263 = property class="Pane"(reference=w392, "VertScrollbarVisibility"=T3."Always On" ("垂直滚动条可见")) -> ()  [unwired: 1 in, 2 out]
                        n264 = Add(x=w395, y=751) -> (x+y=w396:i32)
                        n265 = property on="分隔栏 6" class="Splitter"("Position"=w396) -> ()  [unwired: 2 in, 2 out]
                      }
                      frame "3" {
                        n266 = property on="分隔栏 7" class="Splitter"() -> ("Position"=w400:i32)  [unwired: 2 in, 2 out]
                        n267 = property class="Pane"(reference=w397, "VertScrollbarVisibility"=T3."Always On" ("垂直滚动条可见")) -> ()  [unwired: 1 in, 2 out]
                        n268 = Add(x=w400, y=751) -> (x+y=w399:i32)
                        n269 = property on="分隔栏 7" class="Splitter"("Position"=w399) -> ()  [unwired: 2 in, 2 out]
                      }
                      frame "4" {
                        n270 = property on="分隔栏 8" class="Splitter"() -> ("Position"=w403:i32)  [unwired: 2 in, 2 out]
                        n271 = property class="Pane"(reference=w404, "VertScrollbarVisibility"=T3."Always On" ("垂直滚动条可见")) -> ()  [unwired: 1 in, 2 out]
                        n272 = Add(x=w403, y=751) -> (x+y=w402:i32)
                        n273 = property on="分隔栏 8" class="Splitter"("Position"=w402) -> ()  [unwired: 2 in, 2 out]
                      }
                    }
                  }
                }
              }
            }
          }
        }
      }
    }
  }
  n274 = property on="当前温度 2" class="DigNum (严格)" props=["Value"]() -> ()  [unwired: 2 in, 3 out]
  n275 = property on="队列输出 2" class="TypRef (严格)" props=["Value"]() -> ()  [unwired: 2 in, 3 out]
  n276 = disable-structure shown="禁用" {
    disable-tunnel: [w407 _] -> w77
    frame Disabled {
      w416 = u16 0 items=["无", "奇", "偶"] ("parity (Even)")
      n277 = To Variant(anything="VISA resource name") -> (Variant=w413:variant)
      n278 = Variant To Data(type="", Variant=w413) -> (data=→"数据":string)  [unwired: 1 in, 1 out]
      n279 = call-poly <vilib>:"Create Master Instance.vi"("serial type"=enum16{"RTU", "ASCII"}."RTU", "parity (Even)"=w416, "unit ID"=u8 1, "baud rate (9600)"=u32 9600, "VISA resource name"="VISA resource name") -> ("error out"=w409:errorcluster, "serial master instance"=w407:refnum<class "Modbus Master.lvclass">)  [unwired: 5 in]
      n280 = property on="字符串" class="Str"("Value"="1" ("字符串")) -> ()  [unwired: 2 in, 2 out]
      n281 = while {
        tunnel: w407 -> [w421]
        tunnel: w409 -> [w419]
        stop <- FALSE stop-if-true
        n282 = Wait (ms)(milliseconds to wait=u32 100 ("等待时间（毫秒）")) -> ()  [unwired: 1 out]
        n283 = case shown="\"1\", 默认" "字符串" {
          tunnel: w421 -> [w434 w450 _]
          tunnel: w419 -> [w433 w449 _]
          tunnel: [w430 w440 _] -> _
          tunnel: [w429 w439 _] -> _
          frame "1", Default {
            n284 = call-dynamic "Read Holding Registers.vi"("error in (no error)"=w433, "number of holding registers"=u16 1, "starting address"=u16 258, "Modbus master in"=w434) -> ("error out"=w429:errorcluster, "register values"=w428:u16[], "Modbus master out"=w430:refnum<class "Modbus Master.lvclass">)  [unwired: 5 in]
            "error out" <- w429
            n285 = Index Array(array=w428, index=0 ("索引")) -> (element=w426:u16)
            n286 = To Double Precision Float(number=w426) -> (double precision float=w425:dbl)
            n287 = Divide(x=w425, y=10.0) -> (x/y=→"当前温度 2":dbl)
          }
          frame "2" {
            n288 = call-dynamic "Read Holding Registers.vi"("error in (no error)"=w449, "number of holding registers"=u16 1, "starting address"=u16 258, "Modbus master in"=w450) -> ("error out"=w439:errorcluster, "register values"=w446:u16[], "Modbus master out"=w440:refnum<class "Modbus Master.lvclass">)  [unwired: 5 in]
            n289 = Index Array(array=w446, index=0 ("索引")) -> (element=w444:u16)
            n290 = To Double Precision Float(number=w444) -> (double precision float=w443:dbl)
            n291 = Divide(x=w443, y=10.0) -> (x/y=w435:dbl)
            n292 = Divide(x="文本下拉列表", y=u16 100) -> (x/y=w437:dbl)
            n293 = Greater Or Equal?(x=w435, y=w437) -> (x >= y?=w441:bool)
            n294 = case shown="真" w441 {
              tunnel: w440 -> [_ w452]
              tunnel: w439 -> [_ w451]
              frame False {
              }
              frame True {
                n295 = flat-sequence {
                  tunnel: w452 -> [w454]
                  tunnel: w451 -> [w453]
                  frame #0 {
                    n296 = call-dynamic "Write Single Holding Register.vi"("error in (no error)"=w453, "holding register value"=u16 2, "address"=u16 56, "Modbus master in"=w454) -> ()  [unwired: 6 in, 2 out]
                  }
                  frame #1 {
                    n297 = property on="字符串" class="Str"("Value"="1" ("字符串")) -> ()  [unwired: 2 in, 2 out]
                  }
                }
              }
            }
          }
          frame "0" {
          }
        }
      }
    }
    frame Enabled {
    }
  }
  n298 = while {
    tunnel: w77 -> [w458]
    tunnel: w56 -> [_]
    tunnel: w36 -> [_]
    stop <- FALSE stop-if-true
    n299 = event shown="[6] \"开始测量\", \"开始测量 2\", \"开始测量 3\", \"开始测量 4\": 值改变" {
      selector: _ -> [_ _ _ _ _ _ _ _ _ _ _ _ _ _ _ _]
      dyn-events: _ -> [_ _ _ _ _ _ _ _ _ _ _ _ _ _ _ _]
      timeout: 100 -> [_ _ _ _ _ _ _ _ _ _ _ _ _ _ _ _]
      tunnel: w458 -> [_ _ _ _ _ _ _ _ _ _ _ _ _ _ w1574 _]
      event Timeout {
        n300 = event-data() -> ()  [unwired: 1 in, 3 out]
      }
      event "保存所有", "配置", "连接", "分析", "退出": Mouse Down {
        n301 = event-data() -> ("CtlRef"=w462:refnum<vi>)  [unwired: 1 in, 7 out]
        n302 = flat-sequence {
          tunnel: w462 -> [w473]
          tunnel: [w463] -> w461
          tunnel: w461 -> [w485]
          frame #0 {
            n303 = property class="Bool (严格)"(reference=w473) -> ("Label.Text"=w463:string)  [unwired: 1 in, 2 out]
            n304 = Search 1D Array(1D array=string[] ["保存", "分析", "配置", "连接", "退出"], element=w463, start index (0)=0 ("开始索引(0)")) -> (index of element=w469:i32)
            n305 = Delete From Array(array=i32[] [0, 1, 2, 3, 4], length=1 ("长度"), index=w469) -> (deleted portion=w466:i32[], array with subset deleted=w467:i32[])
            n306 = Index Array(array=w466, index=0 ("索引")) -> (element=w464:i32)
            n307 = flat-sequence {
              tunnel: w467 -> [w476]
              tunnel: [w475] -> w474
              tunnel: w464 -> [w475]
              tunnel: w474 -> [w482]
              frame #0 {
                n308 = for {
                  tunnel: w476 -> [w480] mode=indexing
                  n309 = property on="窗格" class="Pane"() -> ("Decos[]"=w477:refnum<vi>[])  [unwired: 2 in, 2 out]
                  n310 = Index Array(array=w477, index=w480) -> (element=w479:refnum<vi>)
                  n311 = property class="Decor"(reference=w479, "Visible"=FALSE ("可见")) -> ()  [unwired: 1 in, 2 out]
                }
              }
              frame #1 {
                n312 = property on="窗格" class="Pane"() -> ("Decos[]"=w481:refnum<vi>[])  [unwired: 2 in, 2 out]
                n313 = Index Array(array=w481, index=w482) -> (element=w483:refnum<vi>)
                n314 = property class="Decor"(reference=w483, "Visible"=TRUE ("可见")) -> ()  [unwired: 1 in, 2 out]
              }
            }
          }
          frame #1 {
            n315 = case shown="\"分析\"" w485 {
              frame "假", Default {
              }
              frame "连接" {
                n316 = flat-sequence {
                  frame #0 {
                    n317 = property on="分隔栏 3" class="Splitter"() -> ("Position"=w488:i32)  [unwired: 2 in, 2 out]
                    n318 = Equal?(x=w488, y=116) -> (x = y?=w486:bool)
                    n319 = case shown="假" w486 {
                      frame False {
                        n320 = property on="分隔栏 3" class="Splitter"() -> ("Position"=w490:i32)  [unwired: 2 in, 2 out]
                        n321 = Greater?(x=w490, y=508) -> (0:w489:bool)
                        n322 = case shown="真" w489 {
                          frame False {
                          }
                          frame True {
                            n323 = while {
                              i -> [w499]
                              stop <- w492 stop-if-true
                              n324 = Multiply(x=50, y=w499) -> (x*y=w496:i32)
                              n325 = Subtract(x=509, y=w496) -> (x-y=w493:i32)
                              n326 = Less?(x=w493, y=166) -> (x < y?=w494:bool)
                              n327 = case shown="假" w494 {
                                tunnel: w493 -> [w500 _]
                                tunnel: [FALSE TRUE] -> w492
                                frame False {
                                n328 = property on="分隔栏 3" class="Splitter"("Position"=w500) -> ()  [unwired: 2 in, 2 out]
                                }
                                frame True {
                                n329 = property on="分隔栏 3" class="Splitter"("Position"=116 ("分隔栏位置")) -> ()  [unwired: 2 in, 2 out]
                                }
                              }
                            }
                          }
                        }
                      }
                      frame True {
                      }
                    }
                  }
                  frame #1 {
                    n330 = property on="分隔栏 2" class="Splitter"() -> ("Position"=w506:i32)  [unwired: 2 in, 2 out]
                    n331 = Equal?(x=w506, y=113) -> (x = y?=w505:bool)
                    n332 = case shown="真" w505 {
                      frame True {
                        n333 = while {
                          i -> [w514]
                          stop <- w507 stop-if-true
                          n334 = Multiply(x=50, y=w514) -> (x*y=w511:i32)
                          n335 = Add(x=113, y=w511) -> (x+y=w508:i32)
                          n336 = Greater?(x=w508, y=398) -> (0:w509:bool)
                          n337 = case shown="真" w509 {
                            tunnel: w508 -> [w515 _]
                            tunnel: [FALSE TRUE] -> w507
                            frame False {
                              n338 = property on="分隔栏 2" class="Splitter"("Position"=w515) -> ()  [unwired: 2 in, 2 out]
                            }
                            frame True {
                              n339 = property on="分隔栏 2" class="Splitter"("Position"=505 ("分隔栏位置")) -> ()  [unwired: 2 in, 2 out]
                            }
                          }
                        }
                      }
                      frame False {
                        n340 = while {
                          i -> [w526]
                          stop <- w519 stop-if-true
                          n341 = Multiply(x=50, y=w526) -> (x*y=w523:i32)
                          n342 = Subtract(x=448, y=w523) -> (x-y=w520:i32)
                          n343 = Less?(x=w520, y=163) -> (x < y?=w521:bool)
                          n344 = case shown="真" w521 {
                            tunnel: w520 -> [w527 _]
                            tunnel: [FALSE TRUE] -> w519
                            frame False {
                              n345 = property on="分隔栏 2" class="Splitter"("Position"=w527) -> ()  [unwired: 2 in, 2 out]
                            }
                            frame True {
                              n346 = property on="分隔栏 2" class="Splitter"("Position"=113 ("分隔栏位置")) -> ()  [unwired: 2 in, 2 out]
                            }
                          }
                        }
                      }
                    }
                  }
                }
              }
              frame "配置" {
                n347 = flat-sequence {
                  frame #0 {
                    n348 = property on="分隔栏 2" class="Splitter"() -> ("Position"=w532:i32)  [unwired: 2 in, 2 out]
                    n349 = Equal?(x=w532, y=113) -> (x = y?=w533:bool)
                    n350 = case shown="假" w533 {
                      frame False {
                        n351 = while {
                          i -> [w542]
                          stop <- w535 stop-if-true
                          n352 = Multiply(x=50, y=w542) -> (x*y=w539:i32)
                          n353 = Subtract(x=448, y=w539) -> (x-y=w536:i32)
                          n354 = Less?(x=w536, y=163) -> (x < y?=w537:bool)
                          n355 = case shown="真" w537 {
                            tunnel: w536 -> [w543 _]
                            tunnel: [FALSE TRUE] -> w535
                            frame False {
                              n356 = property on="分隔栏 2" class="Splitter"("Position"=w543) -> ()  [unwired: 2 in, 2 out]
                            }
                            frame True {
                              n357 = property on="分隔栏 2" class="Splitter"("Position"=113 ("分隔栏位置")) -> ()  [unwired: 2 in, 2 out]
                            }
                          }
                        }
                      }
                      frame True {
                      }
                    }
                  }
                  frame #1 {
                    n358 = property on="分隔栏 3" class="Splitter"() -> ("Position"=w547:i32)  [unwired: 2 in, 2 out]
                    n359 = Equal?(x=w547, y=116) -> (x = y?=w549:bool)
                    n360 = case shown="假" w549 {
                      frame True {
                        n361 = while {
                          i -> [w557]
                          stop <- w550 stop-if-true
                          n362 = Multiply(x=50, y=w557) -> (x*y=w554:i32)
                          n363 = Add(x=116, y=w554) -> (x+y=w551:i32)
                          n364 = Greater?(x=w551, y=459) -> (0:w552:bool)
                          n365 = case shown="真" w552 {
                            tunnel: w551 -> [w558 _]
                            tunnel: [FALSE TRUE] -> w550
                            frame False {
                              n366 = property on="分隔栏 3" class="Splitter"("Position"=w558) -> ()  [unwired: 2 in, 2 out]
                            }
                            frame True {
                              n367 = property on="分隔栏 3" class="Splitter"("Position"=509 ("分隔栏位置")) -> ()  [unwired: 2 in, 2 out]
                            }
                          }
                        }
                      }
                      frame False {
                        n368 = while {
                          i -> [w569]
                          stop <- w562 stop-if-true
                          n369 = Multiply(x=50, y=w569) -> (x*y=w566:i32)
                          n370 = Subtract(x=509, y=w566) -> (x-y=w563:i32)
                          n371 = Less?(x=w563, y=166) -> (x < y?=w564:bool)
                          n372 = case shown="真" w564 {
                            tunnel: w563 -> [w570 _]
                            tunnel: [FALSE TRUE] -> w562
                            frame False {
                              n373 = property on="分隔栏 3" class="Splitter"("Position"=w570) -> ()  [unwired: 2 in, 2 out]
                            }
                            frame True {
                              n374 = property on="分隔栏 3" class="Splitter"("Position"=116 ("分隔栏位置")) -> ()  [unwired: 2 in, 2 out]
                            }
                          }
                        }
                      }
                    }
                  }
                }
                n375 = property on="选项卡控件 2" class="TabCtl (严格)"("Value"=enum32{"选项卡 1", "选项卡 2", "选项卡 3"}."选项卡 1" ("选项卡控件 2")) -> ()  [unwired: 2 in, 2 out]
              }
              frame "分析" {
                n376 = property on="测试项目" class="RadioBtnsControl (严格)"() -> ("Value"=w575:enum32{"EIS", "极化曲线", "耐久性曲线", "线性扫描"})  [unwired: 2 in, 2 out]
                n377 = property on="选项卡控件 2" class="TabCtl (严格)"("Value"=enum32{"选项卡 1", "选项卡 2", "选项卡 3"}."选项卡 3" ("选项卡控件 2")) -> ()  [unwired: 2 in, 2 out]
                n378 = case shown="\"极化曲线\"" w575 {
                  frame "EIS", Default {
                  }
                  frame "极化曲线" {
                    n379 = flat-sequence {
                      frame #0 {
                        n380 = flat-sequence {
                          frame #0 {
                            "数组 8" <- string[] ["温度", "水质", "极化曲线", "压力", "工步列表"]
                          }
                          frame #1 {
                            n381 = stacked-sequence {
                              frame #0 {
                                n382 = flat-sequence {
                                frame #0 {
                                n383 = stacked-sequence {
                                frame #0 {
                                n384 = property on="分隔栏 4" class="Splitter"() -> ("Position"=w578:i32)  [unwired: 2 in, 2 out]
                                n385 = Add(x=w578, y=32 ("分隔栏位置")) -> (x+y=w580:i32)
                                n386 = property on="分隔栏 5" class="Splitter"("Position"=w580) -> ()  [unwired: 2 in, 2 out]
                                }
                                frame #1 {
                                n387 = property on="分隔栏 4" class="Splitter"() -> ("Position"=w583:i32)  [unwired: 2 in, 2 out]
                                n388 = Add(x=w583, y=62 ("分隔栏位置")) -> (x+y=w582:i32)
                                n389 = property on="分隔栏 6" class="Splitter"("Position"=w582) -> ()  [unwired: 2 in, 2 out]
                                }
                                frame #2 {
                                n390 = property on="分隔栏 4" class="Splitter"() -> ("Position"=w586:i32)  [unwired: 2 in, 2 out]
                                n391 = Add(x=w586, y=92 ("分隔栏位置")) -> (x+y=w585:i32)
                                n392 = property on="分隔栏 7" class="Splitter"("Position"=w585) -> ()  [unwired: 2 in, 2 out]
                                }
                                frame #3 {
                                n393 = property on="分隔栏 4" class="Splitter"() -> ("Position"=w589:i32)  [unwired: 2 in, 2 out]
                                n394 = Add(x=w589, y=122 ("分隔栏位置")) -> (x+y=w587:i32)
                                n395 = property on="分隔栏 8" class="Splitter"("Position"=w587) -> ()  [unwired: 2 in, 2 out]
                                }
                                }
                                }
                                frame #1 {
                                n396 = property on="1" class="Bool (严格)"("Value"=FALSE ("1")) -> ()  [unwired: 2 in, 2 out]
                                n397 = property on="2" class="Bool (严格)"("Value"=FALSE ("2")) -> ()  [unwired: 2 in, 2 out]
                                n398 = property on="3" class="Bool (严格)"("Value"=FALSE ("3")) -> ()  [unwired: 2 in, 2 out]
                                n399 = property on="4" class="Bool (严格)"("Value"=FALSE ("4")) -> ()  [unwired: 2 in, 2 out]
                                }
                                frame #2 {
                                n400 = control-ref of="窗格 8"() -> (w598:refnum<vi>)
                                n401 = control-ref of="窗格 7"() -> (w599:refnum<vi>)
                                n402 = control-ref of="窗格 6"() -> (w600:refnum<vi>)
                                n403 = control-ref of="窗格 9"() -> (w601:refnum<vi>)
                                n404 = property class="Pane"(reference=w598, "VertScrollbarVisibility"=T3."Always Off" ("垂直滚动条可见")) -> ()  [unwired: 1 in, 2 out]
                                n405 = property class="Pane"(reference=w599, "VertScrollbarVisibility"=T3."Always Off" ("垂直滚动条可见")) -> ()  [unwired: 1 in, 2 out]
                                n406 = property class="Pane"(reference=w600, "VertScrollbarVisibility"=T3."Always Off" ("垂直滚动条可见")) -> ()  [unwired: 1 in, 2 out]
                                n407 = property class="Pane"(reference=w601, "VertScrollbarVisibility"=T3."Always Off" ("垂直滚动条可见")) -> ()  [unwired: 1 in, 2 out]
                                }
                                }
                              }
                              frame #1 {
                                n408 = property on="分隔栏 2" class="Splitter"() -> ("Position"=w605:i32)  [unwired: 2 in, 2 out]
                                n409 = property on="分隔栏 3" class="Splitter"() -> ("Position"=w606:i32)  [unwired: 2 in, 2 out]
                                n410 = Equal?(x=w605, y=113) -> (x = y?=w604:bool)
                                n411 = Equal?(x=w606, y=116) -> (x = y?=w607:bool)
                                n412 = case shown="假" w607 {
                                frame False {
                                n413 = property on="分隔栏 3" class="Splitter"() -> ("Position"=w609:i32)  [unwired: 2 in, 2 out]
                                n414 = Greater?(x=w609, y=508) -> (0:w608:bool)
                                n415 = case shown="真" w608 {
                                frame False {
                                }
                                frame True {
                                n416 = while {
                                i -> [w618]
                                stop <- w611 stop-if-true
                                n417 = Multiply(x=10, y=w618) -> (x*y=w615:i32)
                                n418 = Subtract(x=509, y=w615) -> (x-y=w612:i32)
                                n419 = Less?(x=w612, y=166) -> (x < y?=w613:bool)
                                n420 = case shown="真" w613 {
                                tunnel: w612 -> [w619 _]
                                tunnel: [FALSE TRUE] -> w611
                                frame False {
                                n421 = property on="分隔栏 3" class="Splitter"("Position"=w619) -> ()  [unwired: 2 in, 2 out]
                                }
                                frame True {
                                n422 = property on="分隔栏 3" class="Splitter"("Position"=116 ("分隔栏位置")) -> ()  [unwired: 2 in, 2 out]
                                }
                                }
                                }
                                }
                                }
                                }
                                frame True {
                                }
                                }
                                n423 = case shown="假" w604 {
                                frame False {
                                n424 = while {
                                i -> [w630]
                                stop <- w623 stop-if-true
                                n425 = Multiply(x=10, y=w630) -> (x*y=w627:i32)
                                n426 = Subtract(x=448, y=w627) -> (x-y=w624:i32)
                                n427 = Less?(x=w624, y=163) -> (x < y?=w625:bool)
                                n428 = case shown="假" w625 {
                                tunnel: w624 -> [w631 _]
                                tunnel: [FALSE TRUE] -> w623
                                frame False {
                                n429 = property on="分隔栏 2" class="Splitter"("Position"=w631) -> ()  [unwired: 2 in, 2 out]
                                }
                                frame True {
                                n430 = property on="分隔栏 2" class="Splitter"("Position"=113 ("分隔栏位置")) -> ()  [unwired: 2 in, 2 out]
                                }
                                }
                                }
                                }
                                frame True {
                                }
                                }
                              }
                            }
                            n431 = property on="数组 3" class="Arr (严格)"() -> ("Value"=w577:refnum<vi>[])  [unwired: 2 in, 2 out]
                            n432 = for {
                              tunnel: w577 -> [w641] mode=indexing
                              n433 = property class="VI"(reference=w641) -> ("Name"=w640:string)  [unwired: 1 in, 2 out]
                              n434 = Search/Split String(string=w640, search string/char (-)=".") -> (substring before match=w638:string)  [unwired: 1 in, 2 out]
                              n435 = property on="数组 8" class="Arr (严格)"() -> ("Value"=w637:string[])  [unwired: 2 in, 2 out]
                              n436 = Search 1D Array(1D array=w637, element=w638) -> (index of element=w636:i32)  [unwired: 1 in]
                              n437 = Delete From Array(array=w637, index=w636) -> (array with subset deleted=w635:string[])  [unwired: 1 in, 1 out]
                              n438 = property on="数组 8" class="Arr (严格)"("Value"=w635) -> ()  [unwired: 2 in, 2 out]
                            }
                          }
                          frame #2 {
                            n439 = control-ref of="通道选择 2"() -> (w643:refnum<vi>)
                            n440 = register-events(w643) -> (reference out=w642:refnum<event-registration>)  [unwired: 2 in, 1 out]
                            n441 = property on="数组 8" class="Arr (严格)"() -> ("Value"=w644:string[])  [unwired: 2 in, 2 out]
                            n442 = for {
                              tunnel: w644 -> [w646] mode=indexing
                              tunnel: w642 -> [w645]
                              n443 = case shown="\"极化曲线\"" w646 {
                                tunnel: w645 -> [w650 w666 w682 w716 _]
                                frame "温度", Default {
                                n444 = control-ref of="温度1"() -> (w657:refnum<vi>)
                                n445 = control-ref of="温度2"() -> (w658:refnum<vi>)
                                n446 = control-ref of="温度3"() -> (w659:refnum<vi>)
                                n447 = control-ref of="温度4"() -> (w660:refnum<vi>)
                                n448 = Bundle By Name(cluster=T5 {"温度1"=refnum, "温度2"=refnum, "温度3"=refnum, "温度4"=refnum}, "温度1"=w657, "温度2"=w658, "温度3"=w659, "温度4"=w660) -> (w656:T5)
                                n449 = Open VI Reference(type specifier VI Refnum (for type only)=refnum<vi> refnum ("类型说明符VI引用句柄（仅用于类型）"), vi path=path "C:/Users/526computer/Desktop/新建文件夹/温度.vi", options=128 ("选项")) -> (vi reference=w662:refnum<vi>, error out=w661:errorcluster)  [unwired: 3 in]
                                n450 = control-ref of="布尔"() -> (w655:refnum<vi>)
                                n451 = call-by-ref "开始异步调用"(reference=w662, error in=w661, "Bool引用句柄"=w655, "簇"=w656, "事件注册引用句柄 2"=w650) -> (reference out=w647:refnum<vi>)  [unwired: 9 in, 1 out]
                                n452 = property on="数组 3" class="Arr (严格)"() -> ("Value"=w648:refnum<vi>[])  [unwired: 2 in, 2 out]
                                n453 = Insert Into Array(array=w648, new element=w647) -> (w649:refnum<vi>[])  [unwired: 1 in]
                                n454 = property on="数组 3" class="Arr (严格)"("Value"=w649) -> ()  [unwired: 2 in, 2 out]
                                }
                                frame "水质" {
                                n455 = control-ref of="水质1"() -> (w674:refnum<vi>)
                                n456 = control-ref of="水质2"() -> (w675:refnum<vi>)
                                n457 = control-ref of="水质3"() -> (w676:refnum<vi>)
                                n458 = control-ref of="水质4"() -> (w677:refnum<vi>)
                                n459 = Bundle By Name(cluster=T6 {"水质1"=refnum, "水质2"=refnum, "水质3"=refnum, "水质4"=refnum}, "水质1"=w674, "水质2"=w675, "水质3"=w676, "水质4"=w677) -> (w673:T6)
                                n460 = control-ref of="布尔 2"() -> (w671:refnum<vi>)
                                n461 = Open VI Reference(type specifier VI Refnum (for type only)=refnum<vi> refnum ("类型说明符VI引用句柄（仅用于类型）"), vi path=path "C:/Users/526computer/Desktop/新建文件夹/水质.vi", options=128 ("选项")) -> (vi reference=w672:refnum<vi>, error out=w678:errorcluster)  [unwired: 3 in]
                                n462 = call-by-ref "开始异步调用"(reference=w672, error in=w678, "Bool引用句柄"=w671, "簇"=w673, "事件注册引用句柄"=w666) -> (reference out=w663:refnum<vi>)  [unwired: 9 in, 1 out]
                                n463 = property on="数组 3" class="Arr (严格)"() -> ("Value"=w664:refnum<vi>[])  [unwired: 2 in, 2 out]
                                n464 = Insert Into Array(array=w664, new element=w663) -> (w665:refnum<vi>[])  [unwired: 1 in]
                                n465 = property on="数组 3" class="Arr (严格)"("Value"=w665) -> ()  [unwired: 2 in, 2 out]
                                }
                                frame "极化曲线" {
                                n466 = control-ref of="电流4"() -> (w693:refnum<vi>)
                                n467 = control-ref of="电流3"() -> (w694:refnum<vi>)
                                n468 = control-ref of="电流2"() -> (w695:refnum<vi>)
                                n469 = control-ref of="电流1"() -> (w696:refnum<vi>)
                                n470 = Bundle By Name(cluster=T9 {"电流1"=refnum, "电流2"=refnum, "电流3"=refnum, "电流4"=refnum}, "电流1"=w696, "电流2"=w695, "电流3"=w694, "电流4"=w693) -> (w692:T9)
                                n471 = control-ref of="电压3"() -> (w699:refnum<vi>)
                                n472 = control-ref of="电压4"() -> (w698:refnum<vi>)
                                n473 = control-ref of="电压1"() -> (w697:refnum<vi>)
                                n474 = control-ref of="电压2"() -> (w700:refnum<vi>)
                                n475 = Bundle By Name(cluster=T8 {"电压1"=refnum, "电压2"=refnum, "电压3"=refnum, "电压4"=refnum}, "电压1"=w697, "电压2"=w700, "电压3"=w699, "电压4"=w698) -> (w691:T8)
                                n476 = control-ref of="布尔 3"() -> (w689:refnum<vi>)
                                n477 = Open VI Reference(type specifier VI Refnum (for type only)=refnum<vi> refnum ("类型说明符VI引用句柄（仅用于类型）"), vi path=path "C:/Users/526computer/Desktop/新建文件夹/极化曲线.vi", options=128 ("选项")) -> (vi reference=w706:refnum<vi>, error out=w705:errorcluster)  [unwired: 3 in]
                                n478 = control-ref of="极化曲线3"() -> (w703:refnum<vi>)
                                n479 = control-ref of="极化曲线4"() -> (w704:refnum<vi>)
                                n480 = control-ref of="极化曲线1"() -> (w701:refnum<vi>)
                                n481 = control-ref of="极化曲线2"() -> (w702:refnum<vi>)
                                n482 = property on="数组 3" class="Arr (严格)"() -> ("Value"=w680:refnum<vi>[])  [unwired: 2 in, 2 out]
                                n483 = Bundle By Name(cluster=T7 {"极化曲线1"=refnum, "极化曲线2"=refnum, "极化曲线3"=refnum, "极化曲线4"=refnum}, "极化曲线1"=w701, "极化曲线2"=w702, "极化曲线3"=w703, "极化曲线4"=w704) -> (w690:T7)
                                n484 = call-by-ref "开始异步调用"(reference=w706, error in=w705, "Bool引用句柄"=w689, "输出簇 3"=w690, "输出簇 2"=w691, "输出簇"=w692, "事件注册引用句柄 2"=w682) -> (reference out=w679:refnum<vi>)  [unwired: 7 in, 1 out]
                                n485 = Insert Into Array(array=w680, new element=w679) -> (w681:refnum<vi>[])  [unwired: 1 in]
                                n486 = property on="数组 3" class="Arr (严格)"("Value"=w681) -> ()  [unwired: 2 in, 2 out]
                                }
                                frame "压力" {
                                n487 = control-ref of="压力1"() -> (w711:refnum<vi>)
                                n488 = control-ref of="压力2"() -> (w710:refnum<vi>)
                                n489 = control-ref of="压力3"() -> (w709:refnum<vi>)
                                n490 = control-ref of="压力4"() -> (w708:refnum<vi>)
                                n491 = Bundle By Name(cluster=T10 {"压力1"=refnum, "压力2"=refnum, "压力3"=refnum, "压力4"=refnum}, "压力1"=w711, "压力2"=w710, "压力3"=w709, "压力4"=w708) -> (w707:T10)
                                n492 = control-ref of="布尔 4"() -> (w720:refnum<vi>)
                                n493 = Open VI Reference(type specifier VI Refnum (for type only)=refnum<vi> refnum ("类型说明符VI引用句柄（仅用于类型）"), vi path=path "C:/Users/526computer/Desktop/新建文件夹/压力.vi", options=128 ("选项")) -> (vi reference=w721:refnum<vi>, error out=w722:errorcluster)  [unwired: 3 in]
                                n494 = call-by-ref "开始异步调用"(reference=w721, error in=w722, "Bool引用句柄"=w720, "簇"=w707, "事件注册引用句柄 2"=w716) -> (reference out=w713:refnum<vi>)  [unwired: 9 in, 1 out]
                                n495 = property on="数组 3" class="Arr (严格)"() -> ("Value"=w714:refnum<vi>[])  [unwired: 2 in, 2 out]
                                n496 = Insert Into Array(array=w714, new element=w713) -> (w715:refnum<vi>[])  [unwired: 1 in]
                                n497 = property on="数组 3" class="Arr (严格)"("Value"=w715) -> ()  [unwired: 2 in, 2 out]
                                }
                                frame "工步列表" {
                                w729 = string[][] [["1", "CC", "15", "0.95", "1700", "20"], ["2", "CC", "15", "2.15", "1700", "20"], ["3", "CC", "15", "3.35", "1700", "20"], ["4", "CC", "15", "4.55", "1700", "20"], ["5", "CC", "15", "5.75", "1700", "20"], ["6", "CC", "15", "6.95", "1700", "20"], ["7", "CC", "15", "8.15", "1700", "20"], ["8", "CC", "15", "9.35", "1700", "20"], ["9", "CC", "15", "10.55", "1700", "20"], ["10", "CC", "15", "11.75", "1700", "20"], ["11", "CC", "15", "12.95", "1700", "20"], ["12", "CC", "15", "14.15", "1700", "20"], ["13", "CC", "15", "15.35", "1700", "20"], ["14", "CC", "15", "16.55", "1700", "20"], ["15", "CC", "15", "17.75", "1700", "20"], ["16", "CC", "15", "18.95", "1700", "180"], ["17", "CC", "15", "20.15", "1700", "180"], ["18", "CC", "15", "21.35", "1700", "180"], ["19", "CC", "15", "22.55", "1700", "180"], ["20", "CC", "15", "23.75", "1700", "180"], ["21", "CC", "15", "24.95", "1700", "180"], ["22", "CC", "15", "26.15", "1700", "180"], ["23", "CC", "15", "27.35", "1700", "180"], ["24", "CC", "15", "28.55", "1700", "180"], ["25", "CC", "15", "29.75", "1700", "180"], ["26", "CC", "15", "30.95", "1700", "180"], ["27", "CC", "15", "32.15", "1700", "180"], ["28", "CC", "15", "33.35", "1700", "180"], ["29", "CC", "15", "34.55", "1700", "180"], ["30", "CC", "15", "35.75", "1700", "180"], ["31", "CC", "15", "36.95", "1700", "180"], ["32", "CC", "15", "38.15", "1700", "180"], ["33", "CC", "15", "39.35", "1700", "180"], ["34", "CC", "15", "40.55", "1700", "180"], ["35", "CC", "15", "41.75", "1700", "180"], ["36", "CC", "15", "42.95", "1700", "180"], ["37", "CC", "15", "44.15", "1700", "180"], ["38", "CC", "15", "45.35", "1700", "180"], ["39", "CC", "15", "46.55", "1700", "180"], ["40", "CC", "15", "47.75", "1700", "180"], ["41", "CC", "15", "48.95", "1700", "180"], ["42", "CC", "15", "50.15", "1700", "180"], ["43", "CC", "15", "51.35", "1700", "180"], ["44", "CC", "15", "52.55", "1700", "180"], ["45", "CC", "15", "53.75", "1700", "180"], ["46", "CC", "15", "54.95", "1700", "180"], ["47", "CC", "15", "56.15", "1700", "180"], ["48", "CC", "15", "57.35", "1700", "180"], ["49", "CC", "15", "58.55", "1700", "180"], ["50", "CC", "15", "59.75", "1700", "180"], ["51", "CC", "15", "60.95", "1700", "180"], ["52", "CC", "15", "62.15", "1700", "180"], ["53", "CC", "15", "63.35", "1700", "180"], ["54", "CC", "15", "64.55", "1700", "180"], ["55", "CC", "15", "65.75", "1700", "180"], ["56", "CC", "15", "66.95", "1700", "180"], ["57", "CC", "15", "68.15", "1700", "180"], ["58", "CC", "15", "69.35", "1700", "180"], ["59", "CC", "15", "70.55", "1700", "180"], ["60", "CC", "15", "71.75", "1700", "180"], ["61", "CC", "15", "72.95", "1700", "180"], ["62", "CC", "15", "74.15", "1700", "180"], ["63", "CC", "15", "75.35", "1700", "180"], ["64", "CC", "15", "76.55", "1700", "180"], ["65", "CC", "15", "77.75", "1700", "180"], ["66", "CC", "15", "78.95", "1700", "180"], ["67", "CC", "15", "80.15", "1700", "180"], ["68", "CC", "15", "81.35", "1700", "180"], ["69", "CC", "15", "82.55", "1700", "180"], ["70", "CC", "15", "83.75", "1700", "180"], ["71", "CC", "15", "84.95", "1700", "180"], ["72", "CC", "15", "86.15", "1700", "180"], ["73", "CC", "15", "87.35", "1700", "180"], ["74", "CC", "15", "88.55", "1700", "180"], ["75", "CC", "15", "89.75", "1700", "180"], ["76", "CC", "15", "90.95", "1700", "180"], ["77", "CC", "15", "92.15", "1700", "180"], ["78", "CC", "15", "93.35", "1700", "180"], ["79", "CC", "15", "94.55", "1700", "180"], ["80", "CC", "15", "95.75", "1700", "180"], ["81", "CC", "15", "96.95", "1700", "180"], ["82", "CC", "15", "98.15", "1700", "180"], ["83", "CC", "15", "99.35", "1700", "180"], ["84", "CC", "15", "100.55", "1700", "180"], [" ", " ", " ", " ", " ", " "]] ("已删除元素的数组子集")
                                # "数值 3"
                                n498 = control-ref of="数值"() -> (w738:refnum<vi>)
                                n499 = control-ref of="数值 2"() -> (w737:refnum<vi>)
                                n500 = control-ref of="数值 4"() -> (w735:refnum<vi>)
                                n501 = control-ref of="数值 3"() -> (w736:refnum<vi>)
                                n502 = Build Array(w738, w737, w736, w735) -> (w734:refnum<vi>[])
                                n503 = register-events(w734) -> (reference out=w732:refnum<event-registration>)  [unwired: 2 in, 1 out]
                                n504 = Build Array(string[][] [["1", "CC", "15", "0.95", "1700", "20"], ["2", "CC", "15", "2.15", "1700", "20"], ["3", "CC", "15", "3.35", "1700", "20"], ["4", "CC", "15", "4.55", "1700", "20"], ["5", "CC", "15", "5.75", "1700", "20"], ["6", "CC", "15", "6.95", "1700", "20"], ["7", "CC", "15", "8.15", "1700", "20"], ["8", "CC", "15", "9.35", "1700", "20"], ["9", "CC", "15", "10.55", "1700", "20"], ["10", "CC", "15", "11.75", "1700", "20"], ["11", "CC", "15", "12.95", "1700", "20"], ["12", "CC", "15", "14.15", "1700", "20"], ["13", "CC", "15", "15.35", "1700", "20"], ["14", "CC", "15", "16.55", "1700", "20"], ["15", "CC", "15", "17.75", "1700", "20"], ["16", "CC", "15", "18.95", "1700", "180"], ["17", "CC", "15", "20.15", "1700", "180"], ["18", "CC", "15", "21.35", "1700", "180"], ["19", "CC", "15", "22.55", "1700", "180"], ["20", "CC", "15", "23.75", "1700", "180"], ["21", "CC", "15", "24.95", "1700", "180"], ["22", "CC", "15", "26.15", "1700", "180"], ["23", "CC", "15", "27.35", "1700", "180"], ["24", "CC", "15", "28.55", "1700", "180"], ["25", "CC", "15", "29.75", "1700", "180"], ["26", "CC", "15", "30.95", "1700", "180"], ["27", "CC", "15", "32.15", "1700", "180"], ["28", "CC", "15", "33.35", "1700", "180"], ["29", "CC", "15", "34.55", "1700", "180"], ["30", "CC", "15", "35.75", "1700", "180"], ["31", "CC", "15", "36.95", "1700", "180"], ["32", "CC", "15", "38.15", "1700", "180"], ["33", "CC", "15", "39.35", "1700", "180"], ["34", "CC", "15", "40.55", "1700", "180"], ["35", "CC", "15", "41.75", "1700", "180"], ["36", "CC", "15", "42.95", "1700", "180"], ["37", "CC", "15", "44.15", "1700", "180"], ["38", "CC", "15", "45.35", "1700", "180"], ["39", "CC", "15", "46.55", "1700", "180"], ["40", "CC", "15", "47.75", "1700", "180"], ["41", "CC", "15", "48.95", "1700", "180"], ["42", "CC", "15", "50.15", "1700", "180"], ["43", "CC", "15", "51.35", "1700", "180"], ["44", "CC", "15", "52.55", "1700", "180"], ["45", "CC", "15", "53.75", "1700", "180"], ["46", "CC", "15", "54.95", "1700", "180"], ["47", "CC", "15", "56.15", "1700", "180"], ["48", "CC", "15", "57.35", "1700", "180"], ["49", "CC", "15", "58.55", "1700", "180"], ["50", "CC", "15", "59.75", "1700", "180"], ["51", "CC", "15", "60.95", "1700", "180"], ["52", "CC", "15", "62.15", "1700", "180"], ["53", "CC", "15", "63.35", "1700", "180"], ["54", "CC", "15", "64.55", "1700", "180"], ["55", "CC", "15", "65.75", "1700", "180"], ["56", "CC", "15", "66.95", "1700", "180"], ["57", "CC", "15", "68.15", "1700", "180"], ["58", "CC", "15", "69.35", "1700", "180"], ["59", "CC", "15", "70.55", "1700", "180"], ["60", "CC", "15", "71.75", "1700", "180"], ["61", "CC", "15", "72.95", "1700", "180"], ["62", "CC", "15", "74.15", "1700", "180"], ["63", "CC", "15", "75.35", "1700", "180"], ["64", "CC", "15", "76.55", "1700", "180"], ["65", "CC", "15", "77.75", "1700", "180"], ["66", "CC", "15", "78.95", "1700", "180"], ["67", "CC", "15", "80.15", "1700", "180"], ["68", "CC", "15", "81.35", "1700", "180"], ["69", "CC", "15", "82.55", "1700", "180"], ["70", "CC", "15", "83.75", "1700", "180"], ["71", "CC", "15", "84.95", "1700", "180"], ["72", "CC", "15", "86.15", "1700", "180"], ["73", "CC", "15", "87.35", "1700", "180"], ["74", "CC", "15", "88.55", "1700", "180"], ["75", "CC", "15", "89.75", "1700", "180"], ["76", "CC", "15", "90.95", "1700", "180"], ["77", "CC", "15", "92.15", "1700", "180"], ["78", "CC", "15", "93.35", "1700", "180"], ["79", "CC", "15", "94.55", "1700", "180"], ["80", "CC", "15", "95.75", "1700", "180"], ["81", "CC", "15", "96.95", "1700", "180"], ["82", "CC", "15", "98.15", "1700", "180"], ["83", "CC", "15", "99.35", "1700", "180"], ["84", "CC", "15", "100.55", "1700", "180"], [" ", " ", " ", " ", " ", " "]] ("已删除元素的数组子集"), w729, w729, w729) -> (w733:string[][][])
                                n505 = control-ref of="布尔 5"() -> (w731:refnum<vi>)
                                n506 = Open VI Reference(type specifier VI Refnum (for type only)=refnum<vi> refnum ("类型说明符VI引用句柄（仅用于类型）"), vi path=path "C:/Users/526computer/Desktop/新建文件夹/工步列表.vi" ("VI路径"), options=128 ("选项")) -> (vi reference=w740:refnum<vi>, error out=w739:errorcluster)  [unwired: 3 in]
                                n507 = call-by-ref "开始异步调用"(reference=w740, error in=w739, "Bool引用句柄"=w731, "事件注册引用句柄 3"=w732, "添加的数组 2"=w734, "添加的数组"=w733) -> (reference out=w723:refnum<vi>)  [unwired: 8 in, 1 out]
                                n508 = property on="数组 3" class="Arr (严格)"() -> ("Value"=w724:refnum<vi>[])  [unwired: 2 in, 2 out]
                                n509 = Insert Into Array(array=w724, new element=w723) -> (w725:refnum<vi>[])  [unwired: 1 in]
                                n510 = property on="数组 3" class="Arr (严格)"("Value"=w725) -> ()  [unwired: 2 in, 2 out]
                                }
                              }
                            }
                          }
                        }
                      }
                      frame #1 {
                        n511 = property on="数组 3" class="Arr (严格)"() -> ("Value"=w741:refnum<vi>[])  [unwired: 2 in, 2 out]
                        n512 = for {
                          tunnel: w741 -> [w742] mode=indexing
                          n513 = property class="VI"(reference=w742) -> ("Front Panel.Title"=w753:string)  [unwired: 1 in, 2 out]
                          n514 = Wait (ms)(milliseconds to wait=u32 100 ("等待时间（毫秒）")) -> ()  [unwired: 1 out]
                          n515 = Compound Arithmetic op=OR ("复合运算")(1, 2 ("y"), 64 ("值")) -> (w754:i32)
                          n516 = dll-call lib="C:/Users/526computer/Desktop/LABVIEW.dll" fn="findlabview"("lpcallsname"=0, "winname"=w753, "layer"=-1, "x"=0, "y"=0, "cx"=0, "cy"=0, "flag"=w754) -> ()  [unwired: 12 in, 2 out]
                        }
                      }
                    }
                  }
                  frame "耐久性曲线" {
                    n517 = flat-sequence {
                      frame #0 {
                        n518 = flat-sequence {
                          frame #0 {
                            n519 = stacked-sequence {
                              frame #0 {
                                n520 = property on="分隔栏 4" class="Splitter"() -> ("Position"=w755:i32)  [unwired: 2 in, 2 out]
                                n521 = Add(x=w755, y=32 ("分隔栏位置")) -> (x+y=w757:i32)
                                n522 = property on="分隔栏 5" class="Splitter"("Position"=w757) -> ()  [unwired: 2 in, 2 out]
                              }
                              frame #1 {
                                n523 = property on="分隔栏 4" class="Splitter"() -> ("Position"=w760:i32)  [unwired: 2 in, 2 out]
                                n524 = Add(x=w760, y=62 ("分隔栏位置")) -> (x+y=w759:i32)
                                n525 = property on="分隔栏 6" class="Splitter"("Position"=w759) -> ()  [unwired: 2 in, 2 out]
                              }
                              frame #2 {
                                n526 = property on="分隔栏 4" class="Splitter"() -> ("Position"=w763:i32)  [unwired: 2 in, 2 out]
                                n527 = Add(x=w763, y=92 ("分隔栏位置")) -> (x+y=w762:i32)
                                n528 = property on="分隔栏 7" class="Splitter"("Position"=w762) -> ()  [unwired: 2 in, 2 out]
                              }
                              frame #3 {
                                n529 = property on="分隔栏 4" class="Splitter"() -> ("Position"=w766:i32)  [unwired: 2 in, 2 out]
                                n530 = Add(x=w766, y=122 ("分隔栏位置")) -> (x+y=w764:i32)
                                n531 = property on="分隔栏 8" class="Splitter"("Position"=w764) -> ()  [unwired: 2 in, 2 out]
                              }
                            }
                          }
                          frame #1 {
                            n532 = property on="1" class="Bool (严格)"("Value"=FALSE ("1")) -> ()  [unwired: 2 in, 2 out]
                            n533 = property on="2" class="Bool (严格)"("Value"=FALSE ("2")) -> ()  [unwired: 2 in, 2 out]
                            n534 = property on="3" class="Bool (严格)"("Value"=FALSE ("3")) -> ()  [unwired: 2 in, 2 out]
                            n535 = property on="4" class="Bool (严格)"("Value"=FALSE ("4")) -> ()  [unwired: 2 in, 2 out]
                          }
                          frame #2 {
                            n536 = control-ref of="窗格 8"() -> (w775:refnum<vi>)
                            n537 = control-ref of="窗格 7"() -> (w776:refnum<vi>)
                            n538 = control-ref of="窗格 6"() -> (w777:refnum<vi>)
                            n539 = control-ref of="窗格 9"() -> (w778:refnum<vi>)
                            n540 = property class="Pane"(reference=w775, "VertScrollbarVisibility"=T3."Always Off" ("垂直滚动条可见")) -> ()  [unwired: 1 in, 2 out]
                            n541 = property class="Pane"(reference=w776, "VertScrollbarVisibility"=T3."Always Off" ("垂直滚动条可见")) -> ()  [unwired: 1 in, 2 out]
                            n542 = property class="Pane"(reference=w777, "VertScrollbarVisibility"=T3."Always Off" ("垂直滚动条可见")) -> ()  [unwired: 1 in, 2 out]
                            n543 = property class="Pane"(reference=w778, "VertScrollbarVisibility"=T3."Always Off" ("垂直滚动条可见")) -> ()  [unwired: 1 in, 2 out]
                          }
                        }
                      }
                      frame #1 {
                        n544 = property on="分隔栏 2" class="Splitter"() -> ("Position"=w782:i32)  [unwired: 2 in, 2 out]
                        n545 = property on="分隔栏 3" class="Splitter"() -> ("Position"=w783:i32)  [unwired: 2 in, 2 out]
                        n546 = Equal?(x=w782, y=113) -> (x = y?=w781:bool)
                        n547 = Equal?(x=w783, y=116) -> (x = y?=w784:bool)
                        n548 = case shown="假" w784 {
                          frame False {
                            n549 = property on="分隔栏 3" class="Splitter"() -> ("Position"=w786:i32)  [unwired: 2 in, 2 out]
                            n550 = Greater?(x=w786, y=508) -> (0:w785:bool)
                            n551 = case shown="真" w785 {
                              frame False {
                              }
                              frame True {
                                n552 = while {
                                i -> [w795]
                                stop <- w788 stop-if-true
                                n553 = Multiply(x=10, y=w795) -> (x*y=w792:i32)
                                n554 = Subtract(x=509, y=w792) -> (x-y=w789:i32)
                                n555 = Less?(x=w789, y=166) -> (x < y?=w790:bool)
                                n556 = case shown="真" w790 {
                                tunnel: w789 -> [w796 _]
                                tunnel: [FALSE TRUE] -> w788
                                frame False {
                                n557 = property on="分隔栏 3" class="Splitter"("Position"=w796) -> ()  [unwired: 2 in, 2 out]
                                }
                                frame True {
                                n558 = property on="分隔栏 3" class="Splitter"("Position"=116 ("分隔栏位置")) -> ()  [unwired: 2 in, 2 out]
                                }
                                }
                                }
                              }
                            }
                          }
                          frame True {
                          }
                        }
                        n559 = case shown="假" w781 {
                          frame False {
                            n560 = while {
                              i -> [w807]
                              stop <- w800 stop-if-true
                              n561 = Multiply(x=10, y=w807) -> (x*y=w804:i32)
                              n562 = Subtract(x=448, y=w804) -> (x-y=w801:i32)
                              n563 = Less?(x=w801, y=163) -> (x < y?=w802:bool)
                              n564 = case shown="假" w802 {
                                tunnel: w801 -> [w808 _]
                                tunnel: [FALSE TRUE] -> w800
                                frame False {
                                n565 = property on="分隔栏 2" class="Splitter"("Position"=w808) -> ()  [unwired: 2 in, 2 out]
                                }
                                frame True {
                                n566 = property on="分隔栏 2" class="Splitter"("Position"=113 ("分隔栏位置")) -> ()  [unwired: 2 in, 2 out]
                                }
                              }
                            }
                          }
                          frame True {
                          }
                        }
                      }
                      frame #2 {
                        n567 = control-ref of="电流1"() -> (w826:refnum<vi>)
                        n568 = control-ref of="电流2"() -> (w825:refnum<vi>)
                        n569 = control-ref of="电流3"() -> (w824:refnum<vi>)
                        n570 = control-ref of="电流4"() -> (w823:refnum<vi>)
                        n571 = control-ref of="电压1"() -> (w827:refnum<vi>)
                        n572 = control-ref of="电压2"() -> (w830:refnum<vi>)
                        n573 = control-ref of="电压3"() -> (w829:refnum<vi>)
                        n574 = control-ref of="电压4"() -> (w828:refnum<vi>)
                        n575 = Bundle By Name(cluster=T9 {"电流1"=refnum, "电流2"=refnum, "电流3"=refnum, "电流4"=refnum}, "电流1"=w826, "电流2"=w825, "电流3"=w824, "电流4"=w823) -> (w822:T9)
                        n576 = Bundle By Name(cluster=T8 {"电压1"=refnum, "电压2"=refnum, "电压3"=refnum, "电压4"=refnum}, "电压1"=w827, "电压2"=w830, "电压3"=w829, "电压4"=w828) -> (w821:T8)
                        n577 = control-ref of="布尔 6"() -> (w820:refnum<vi>)
                        n578 = Open VI Reference(type specifier VI Refnum (for type only)=refnum<vi> refnum ("类型说明符VI引用句柄（仅用于类型）"), vi path=path "C:/Users/526computer/Desktop/新建文件夹/耐久性测试.vi" ("VI路径"), options=128 ("选项")) -> (vi reference=w831:refnum<vi>)  [unwired: 3 in, 1 out]
                        n579 = call-by-ref "开始异步调用"(reference=w831, "Bool引用句柄"=w820, "输出簇 2"=w821, "输出簇"=w822, "事件注册引用句柄 2"=refnum<event-registration> refnum ("事件注册引用句柄")) -> (reference out=w813:refnum<vi>)  [unwired: 9 in, 1 out]
                        n580 = Build Array(w813) -> (w812:refnum<vi>[])
                        n581 = property on="数组 9" class="Arr (严格)"("Value"=w812) -> ()  [unwired: 2 in, 2 out]
                      }
                      frame #3 {
                        n582 = Wait (ms)(milliseconds to wait=u32 100 ("等待时间（毫秒）")) -> ()  [unwired: 1 out]
                        n583 = Compound Arithmetic op=OR ("复合运算")(1, 2 ("y"), 64 ("值")) -> (w843:i32)
                        n584 = dll-call lib="C:/Users/526computer/Desktop/LABVIEW.dll" fn="findlabview"("lpcallsname"=0, "winname"="耐久性测试", "layer"=-1, "x"=0, "y"=0, "cx"=0, "cy"=0, "flag"=w843) -> ()  [unwired: 12 in, 2 out]
                      }
                    }
                  }
                  frame "线性扫描" {
                  }
                }
              }
            }
          }
          frame #2 {
          }
        }
      }
      event "连接": Mouse Enter {
        n585 = event-data() -> ()  [unwired: 1 in, 4 out]
        n586 = flat-sequence {
          frame #0 {
            n587 = flat-sequence {
              frame #0 {
                n588 = stacked-sequence {
                  frame #0 {
                    n589 = property on="分隔栏 4" class="Splitter"() -> ("Position"=w844:i32)  [unwired: 2 in, 2 out]
                    n590 = Add(x=w844, y=32 ("分隔栏位置")) -> (x+y=w846:i32)
                    n591 = property on="分隔栏 5" class="Splitter"("Position"=w846) -> ()  [unwired: 2 in, 2 out]
                  }
                  frame #1 {
                    n592 = property on="分隔栏 4" class="Splitter"() -> ("Position"=w849:i32)  [unwired: 2 in, 2 out]
                    n593 = Add(x=w849, y=62 ("分隔栏位置")) -> (x+y=w848:i32)
                    n594 = property on="分隔栏 6" class="Splitter"("Position"=w848) -> ()  [unwired: 2 in, 2 out]
                  }
                  frame #2 {
                    n595 = property on="分隔栏 4" class="Splitter"() -> ("Position"=w852:i32)  [unwired: 2 in, 2 out]
                    n596 = Add(x=w852, y=92 ("分隔栏位置")) -> (x+y=w851:i32)
                    n597 = property on="分隔栏 7" class="Splitter"("Position"=w851) -> ()  [unwired: 2 in, 2 out]
                  }
                  frame #3 {
                    n598 = property on="分隔栏 4" class="Splitter"() -> ("Position"=w855:i32)  [unwired: 2 in, 2 out]
                    n599 = Add(x=w855, y=122 ("分隔栏位置")) -> (x+y=w853:i32)
                    n600 = property on="分隔栏 8" class="Splitter"("Position"=w853) -> ()  [unwired: 2 in, 2 out]
                  }
                }
              }
              frame #1 {
                n601 = property on="1" class="Bool (严格)"("Value"=FALSE ("1")) -> ()  [unwired: 2 in, 2 out]
                n602 = property on="2" class="Bool (严格)"("Value"=FALSE ("2")) -> ()  [unwired: 2 in, 2 out]
                n603 = property on="3" class="Bool (严格)"("Value"=FALSE ("3")) -> ()  [unwired: 2 in, 2 out]
                n604 = property on="4" class="Bool (严格)"("Value"=FALSE ("4")) -> ()  [unwired: 2 in, 2 out]
              }
              frame #2 {
                n605 = control-ref of="窗格 8"() -> (w864:refnum<vi>)
                n606 = control-ref of="窗格 7"() -> (w865:refnum<vi>)
                n607 = control-ref of="窗格 6"() -> (w866:refnum<vi>)
                n608 = control-ref of="窗格 9"() -> (w867:refnum<vi>)
                n609 = property class="Pane"(reference=w864, "VertScrollbarVisibility"=T3."Always Off" ("垂直滚动条可见")) -> ()  [unwired: 1 in, 2 out]
                n610 = property class="Pane"(reference=w865, "VertScrollbarVisibility"=T3."Always Off" ("垂直滚动条可见")) -> ()  [unwired: 1 in, 2 out]
                n611 = property class="Pane"(reference=w866, "VertScrollbarVisibility"=T3."Always Off" ("垂直滚动条可见")) -> ()  [unwired: 1 in, 2 out]
                n612 = property class="Pane"(reference=w867, "VertScrollbarVisibility"=T3."Always Off" ("垂直滚动条可见")) -> ()  [unwired: 1 in, 2 out]
              }
            }
          }
          frame #1 {
            n613 = property on="分隔栏 3" class="Splitter"() -> ("Position"=w870:i32)  [unwired: 2 in, 2 out]
            n614 = Equal?(x=w870, y=116) -> (x = y?=w869:bool)
            n615 = case shown="假" w869 {
              frame False {
                n616 = property on="分隔栏 3" class="Splitter"() -> ("Position"=w872:i32)  [unwired: 2 in, 2 out]
                n617 = Greater?(x=w872, y=508) -> (0:w871:bool)
                n618 = case shown="真" w871 {
                  frame False {
                  }
                  frame True {
                    n619 = while {
                      i -> [w881]
                      stop <- w874 stop-if-true
                      n620 = Multiply(x=10, y=w881) -> (x*y=w878:i32)
                      n621 = Subtract(x=509, y=w878) -> (x-y=w875:i32)
                      n622 = Less?(x=w875, y=166) -> (x < y?=w876:bool)
                      n623 = case shown="真" w876 {
                        tunnel: w875 -> [w882 _]
                        tunnel: [FALSE TRUE] -> w874
                        frame False {
                          n624 = property on="分隔栏 3" class="Splitter"("Position"=w882) -> ()  [unwired: 2 in, 2 out]
                        }
                        frame True {
                          n625 = property on="分隔栏 3" class="Splitter"("Position"=116 ("分隔栏位置")) -> ()  [unwired: 2 in, 2 out]
                        }
                      }
                    }
                  }
                }
              }
              frame True {
              }
            }
          }
          frame #2 {
            n626 = while {
              tunnel: u32 10 ("Delay(ms)") -> [w890]
              stop <- w891 stop-if-true
              n627 = property on="分隔栏 2" class="Splitter"() -> ("Position"=w887:i32)  [unwired: 2 in, 2 out]
              n628 = Wait (ms)(milliseconds to wait=w890) -> ()  [unwired: 1 out]
              n629 = Subtract(x=510 ("y"), y=w887) -> (x-y=w894:i32)
              n630 = expression code="x/10"(w894) -> (w893:i32)
              n631 = Round Toward -Infinity(1:w893) -> (0:w892:i32)
              n632 = Add(x=w887, y=w892) -> (x+y=w888:i32)
              n633 = Equal To 0?(x=w892) -> (x = 0?=w891:bool)
              n634 = property on="分隔栏 2" class="Splitter"("Position"=w888) -> ()  [unwired: 2 in, 2 out]
            }
          }
        }
      }
      event "配置": Mouse Enter {
        n635 = event-data() -> ()  [unwired: 1 in, 4 out]
        n636 = property on="选项卡控件 2" class="TabCtl (严格)"("Value"=enum32{"选项卡 1", "选项卡 2", "选项卡 3"}."选项卡 1" ("选项卡控件 2")) -> ()  [unwired: 2 in, 2 out]
        n637 = flat-sequence {
          frame #0 {
            n638 = flat-sequence {
              frame #0 {
                n639 = stacked-sequence {
                  frame #0 {
                    n640 = property on="分隔栏 4" class="Splitter"() -> ("Position"=w896:i32)  [unwired: 2 in, 2 out]
                    n641 = Add(x=w896, y=32 ("分隔栏位置")) -> (x+y=w898:i32)
                    n642 = property on="分隔栏 5" class="Splitter"("Position"=w898) -> ()  [unwired: 2 in, 2 out]
                  }
                  frame #1 {
                    n643 = property on="分隔栏 4" class="Splitter"() -> ("Position"=w901:i32)  [unwired: 2 in, 2 out]
                    n644 = Add(x=w901, y=62 ("分隔栏位置")) -> (x+y=w900:i32)
                    n645 = property on="分隔栏 6" class="Splitter"("Position"=w900) -> ()  [unwired: 2 in, 2 out]
                  }
                  frame #2 {
                    n646 = property on="分隔栏 4" class="Splitter"() -> ("Position"=w904:i32)  [unwired: 2 in, 2 out]
                    n647 = Add(x=w904, y=92 ("分隔栏位置")) -> (x+y=w903:i32)
                    n648 = property on="分隔栏 7" class="Splitter"("Position"=w903) -> ()  [unwired: 2 in, 2 out]
                  }
                  frame #3 {
                    n649 = property on="分隔栏 4" class="Splitter"() -> ("Position"=w907:i32)  [unwired: 2 in, 2 out]
                    n650 = Add(x=w907, y=122 ("分隔栏位置")) -> (x+y=w905:i32)
                    n651 = property on="分隔栏 8" class="Splitter"("Position"=w905) -> ()  [unwired: 2 in, 2 out]
                  }
                }
              }
              frame #1 {
                n652 = property on="1" class="Bool (严格)"("Value"=FALSE ("1")) -> ()  [unwired: 2 in, 2 out]
                n653 = property on="2" class="Bool (严格)"("Value"=FALSE ("2")) -> ()  [unwired: 2 in, 2 out]
                n654 = property on="3" class="Bool (严格)"("Value"=FALSE ("3")) -> ()  [unwired: 2 in, 2 out]
                n655 = property on="4" class="Bool (严格)"("Value"=FALSE ("4")) -> ()  [unwired: 2 in, 2 out]
              }
              frame #2 {
                n656 = control-ref of="窗格 8"() -> (w916:refnum<vi>)
                n657 = control-ref of="窗格 7"() -> (w917:refnum<vi>)
                n658 = control-ref of="窗格 6"() -> (w918:refnum<vi>)
                n659 = control-ref of="窗格 9"() -> (w919:refnum<vi>)
                n660 = property class="Pane"(reference=w916, "VertScrollbarVisibility"=T3."Always Off" ("垂直滚动条可见")) -> ()  [unwired: 1 in, 2 out]
                n661 = property class="Pane"(reference=w917, "VertScrollbarVisibility"=T3."Always Off" ("垂直滚动条可见")) -> ()  [unwired: 1 in, 2 out]
                n662 = property class="Pane"(reference=w918, "VertScrollbarVisibility"=T3."Always Off" ("垂直滚动条可见")) -> ()  [unwired: 1 in, 2 out]
                n663 = property class="Pane"(reference=w919, "VertScrollbarVisibility"=T3."Always Off" ("垂直滚动条可见")) -> ()  [unwired: 1 in, 2 out]
              }
            }
          }
          frame #1 {
            n664 = property on="分隔栏 2" class="Splitter"() -> ("Position"=w921:i32)  [unwired: 2 in, 2 out]
            n665 = Equal?(x=w921, y=113) -> (x = y?=w922:bool)
            n666 = case shown="假" w922 {
              frame False {
                n667 = while {
                  i -> [w930]
                  stop <- w923 stop-if-true
                  n668 = Multiply(x=10, y=w930) -> (x*y=w927:i32)
                  n669 = Subtract(x=448, y=w927) -> (x-y=w924:i32)
                  n670 = Less?(x=w924, y=163) -> (x < y?=w925:bool)
                  n671 = case shown="假" w925 {
                    tunnel: w924 -> [w931 _]
                    tunnel: [FALSE TRUE] -> w923
                    frame False {
                      n672 = property on="分隔栏 2" class="Splitter"("Position"=w931) -> ()  [unwired: 2 in, 2 out]
                    }
                    frame True {
                      n673 = property on="分隔栏 2" class="Splitter"("Position"=113 ("分隔栏位置")) -> ()  [unwired: 2 in, 2 out]
                    }
                  }
                }
              }
              frame True {
              }
            }
          }
          frame #2 {
            n674 = while {
              tunnel: 10 -> [w939]
              stop <- w940 stop-if-true
              n675 = property on="分隔栏 3" class="Splitter"() -> ("Position"=w937:i32)  [unwired: 2 in, 2 out]
              n676 = Wait (ms)(milliseconds to wait=w939) -> ()  [unwired: 1 out]
              n677 = Subtract(x=514, y=w937) -> (x-y=w943:i32)
              n678 = expression code="x/10"(w943) -> (w942:i32)
              n679 = Round Toward -Infinity(1:w942) -> (0:w941:i32)
              n680 = Add(x=w937, y=w941) -> (x+y=w938:i32)
              n681 = Equal To 0?(x=w941) -> (x = 0?=w940:bool)
              n682 = property on="分隔栏 3" class="Splitter"("Position"=w938) -> ()  [unwired: 2 in, 2 out]
            }
          }
        }
      }
      event "分析": Mouse Enter {
        n683 = event-data() -> ()  [unwired: 1 in, 4 out]
      }
      event "布尔 2", "布尔 3", "布尔 4", "布尔 5", "布尔", "布尔 6": Value Change {
        n684 = event-data() -> ("CtlRef"=w945:refnum<vi>)  [unwired: 1 in, 5 out]
        n685 = property class="Bool (严格)"(reference=w945) -> ("Label.Text"=w944:string)  [unwired: 1 in, 2 out]
        n686 = case shown="\"布尔 6\"" w944 {
          frame "布尔", Default {
            n687 = property on="数组 3" class="Arr (严格)"() -> ("Value"=w946:refnum<vi>[])  [unwired: 2 in, 2 out]
            n688 = for {
              tunnel: w946 -> [w948] mode=indexing
              i -> [w947]
              n689 = property class="VI"(reference=w948) -> ("Name"=w951:string)  [unwired: 1 in, 2 out]
              n690 = Equal?(x=w951, y="温度.vi") -> (x = y?=w949:bool)
              n691 = case shown="真" w949 {
                tunnel: w948 -> [_ w957]
                tunnel: w947 -> [_ w953]
                frame False {
                }
                frame True {
                  n692 = invoke class="VI" method="Abort VI"(reference=w957) -> (reference out=w956:refnum<vi>)  [unwired: 2 in, 2 out]
                  n693 = invoke class="VI" method="FP.Close"(reference=w956) -> (reference out=w955:refnum<vi>)  [unwired: 2 in, 2 out]
                  n694 = Close Reference(reference=w955) -> ()  [unwired: 1 in, 1 out]
                  n695 = property on="数组 3" class="Arr (严格)"() -> ("Value"=w954:refnum<vi>[])  [unwired: 2 in, 2 out]
                  n696 = Delete From Array(array=w954, index=w953) -> (array with subset deleted=w952:refnum<vi>[])  [unwired: 1 in, 1 out]
                  n697 = property on="数组 3" class="Arr (严格)"("Value"=w952) -> ()  [unwired: 2 in, 2 out]
                }
              }
            }
          }
          frame "布尔 2" {
            n698 = property on="数组 3" class="Arr (严格)"() -> ("Value"=w958:refnum<vi>[])  [unwired: 2 in, 2 out]
            n699 = for {
              tunnel: w958 -> [w961] mode=indexing
              i -> [w960]
              n700 = property class="VI"(reference=w961) -> ("Name"=w963:string)  [unwired: 1 in, 2 out]
              n701 = Equal?(x=w963, y="水质.vi") -> (x = y?=w962:bool)
              n702 = case shown="真" w962 {
                tunnel: w961 -> [_ w969]
                tunnel: w960 -> [_ w966]
                frame False {
                }
                frame True {
                  n703 = invoke class="VI" method="Abort VI"(reference=w969) -> (reference out=w968:refnum<vi>)  [unwired: 2 in, 2 out]
                  n704 = invoke class="VI" method="FP.Close"(reference=w968) -> (reference out=w967:refnum<vi>)  [unwired: 2 in, 2 out]
                  n705 = Close Reference(reference=w967) -> ()  [unwired: 1 in, 1 out]
                  n706 = property on="数组 3" class="Arr (严格)"() -> ("Value"=w965:refnum<vi>[])  [unwired: 2 in, 2 out]
                  n707 = Delete From Array(array=w965, index=w966) -> (array with subset deleted=w964:refnum<vi>[])  [unwired: 1 in, 1 out]
                  n708 = property on="数组 3" class="Arr (严格)"("Value"=w964) -> ()  [unwired: 2 in, 2 out]
                }
              }
            }
          }
          frame "布尔 3" {
            n709 = property on="数组 3" class="Arr (严格)"() -> ("Value"=w970:refnum<vi>[])  [unwired: 2 in, 2 out]
            n710 = for {
              tunnel: w970 -> [w973] mode=indexing
              i -> [w972]
              n711 = property class="VI"(reference=w973) -> ("Name"=w975:string)  [unwired: 1 in, 2 out]
              n712 = Equal?(x=w975, y="极化曲线.vi") -> (x = y?=w974:bool)
              n713 = case shown="真" w974 {
                tunnel: w973 -> [_ w981]
                tunnel: w972 -> [_ w978]
                frame False {
                }
                frame True {
                  n714 = invoke class="VI" method="Abort VI"(reference=w981) -> (reference out=w980:refnum<vi>)  [unwired: 2 in, 2 out]
                  n715 = invoke class="VI" method="FP.Close"(reference=w980) -> (reference out=w979:refnum<vi>)  [unwired: 2 in, 2 out]
                  n716 = Close Reference(reference=w979) -> ()  [unwired: 1 in, 1 out]
                  n717 = property on="数组 3" class="Arr (严格)"() -> ("Value"=w976:refnum<vi>[])  [unwired: 2 in, 2 out]
                  n718 = Delete From Array(array=w976, index=w978) -> (array with subset deleted=w977:refnum<vi>[])  [unwired: 1 in, 1 out]
                  n719 = property on="数组 3" class="Arr (严格)"("Value"=w977) -> ()  [unwired: 2 in, 2 out]
                }
              }
            }
          }
          frame "布尔 4" {
            n720 = property on="数组 3" class="Arr (严格)"() -> ("Value"=w982:refnum<vi>[])  [unwired: 2 in, 2 out]
            n721 = for {
              tunnel: w982 -> [w985] mode=indexing
              i -> [w984]
              n722 = property class="VI"(reference=w985) -> ("Name"=w987:string)  [unwired: 1 in, 2 out]
              n723 = Equal?(x=w987, y="压力.vi") -> (x = y?=w986:bool)
              n724 = case shown="真" w986 {
                tunnel: w985 -> [_ w993]
                tunnel: w984 -> [_ w990]
                frame False {
                }
                frame True {
                  n725 = invoke class="VI" method="Abort VI"(reference=w993) -> (reference out=w992:refnum<vi>)  [unwired: 2 in, 2 out]
                  n726 = invoke class="VI" method="FP.Close"(reference=w992) -> (reference out=w991:refnum<vi>)  [unwired: 2 in, 2 out]
                  n727 = Close Reference(reference=w991) -> ()  [unwired: 1 in, 1 out]
                  n728 = property on="数组 3" class="Arr (严格)"() -> ("Value"=w989:refnum<vi>[])  [unwired: 2 in, 2 out]
                  n729 = Delete From Array(array=w989, index=w990) -> (array with subset deleted=w988:refnum<vi>[])  [unwired: 1 in, 1 out]
                  n730 = property on="数组 3" class="Arr (严格)"("Value"=w988) -> ()  [unwired: 2 in, 2 out]
                }
              }
            }
          }
          frame "布尔 5" {
            n731 = property on="数组 3" class="Arr (严格)"() -> ("Value"=w994:refnum<vi>[])  [unwired: 2 in, 2 out]
            n732 = for {
              tunnel: w994 -> [w997] mode=indexing
              i -> [w996]
              n733 = property class="VI"(reference=w997) -> ("Name"=w999:string)  [unwired: 1 in, 2 out]
              n734 = Equal?(x=w999, y="工步列表.vi") -> (x = y?=w998:bool)
              n735 = case shown="真" w998 {
                tunnel: w997 -> [_ w1005]
                tunnel: w996 -> [_ w1002]
                frame False {
                }
                frame True {
                  n736 = invoke class="VI" method="Abort VI"(reference=w1005) -> (reference out=w1004:refnum<vi>)  [unwired: 2 in, 2 out]
                  n737 = invoke class="VI" method="FP.Close"(reference=w1004) -> (reference out=w1003:refnum<vi>)  [unwired: 2 in, 2 out]
                  n738 = Close Reference(reference=w1003) -> ()  [unwired: 1 in, 1 out]
                  n739 = property on="数组 3" class="Arr (严格)"() -> ("Value"=w1001:refnum<vi>[])  [unwired: 2 in, 2 out]
                  n740 = Delete From Array(array=w1001, index=w1002) -> (array with subset deleted=w1000:refnum<vi>[])  [unwired: 1 in, 1 out]
                  n741 = property on="数组 3" class="Arr (严格)"("Value"=w1000) -> ()  [unwired: 2 in, 2 out]
                }
              }
            }
          }
          frame "布尔 6" {
            n742 = flat-sequence {
              frame #0 {
                n743 = property on="数组 9" class="Arr (严格)"() -> ("Value"=w1006:refnum<vi>[])  [unwired: 2 in, 2 out]
                n744 = for {
                  tunnel: w1006 -> [w1007] mode=indexing
                  n745 = invoke class="VI" method="Abort VI"(reference=w1007) -> (reference out=w1009:refnum<vi>)  [unwired: 2 in, 2 out]
                  n746 = invoke class="VI" method="FP.Close"(reference=w1009) -> (reference out=w1008:refnum<vi>)  [unwired: 2 in, 2 out]
                  n747 = Close Reference(reference=w1008) -> ()  [unwired: 1 in, 1 out]
                }
              }
              frame #1 {
                n748 = property on="数组 9" class="Arr (严格)"("Value"=refnum<vi>[] [] ("数组 9")) -> ()  [unwired: 2 in, 2 out]
              }
            }
          }
        }
      }
      event "开始测量", "开始测量 2", "开始测量 3", "开始测量 4": Value Change {
        n749 = event-data() -> ("CtlRef"=w1014:refnum<vi>, "NewVal"=w1012:bool)  [unwired: 1 in, 4 out]
        n750 = property class="Bool (严格)"(reference=w1014) -> ("Label.Text"=w1013:string)  [unwired: 1 in, 2 out]
        n751 = property on="测试项目" class="RadioBtnsControl (严格)"() -> ("Value"=w1011:enum32{"EIS", "极化曲线", "耐久性曲线", "线性扫描"})  [unwired: 2 in, 2 out]
        n752 = case shown="\"极化曲线\"" w1011 {
          tunnel: w1013 -> [_ w1016 w1143 _]
          tunnel: w1012 -> [_ w1015 w1144 _]
          frame "EIS", Default {
          }
          frame "极化曲线" {
            n753 = case shown="真" w1015 {
              tunnel: w1016 -> [w1017 w1038]
              frame False {
                n754 = case shown="\"开始测量\", 默认" w1017 {
                  frame "开始测量", Default {
                    n755 = flat-sequence {
                      frame #0 {
                        n756 = property on="数组 4" class="Arr (严格)"() -> ("Value"=w1018:refnum<vi>[])  [unwired: 2 in, 2 out]
                        n757 = for {
                          tunnel: w1018 -> [w1021] mode=indexing
                          n758 = invoke class="VI" method="Abort VI"(reference=w1021) -> (reference out=w1020:refnum<vi>)  [unwired: 2 in, 2 out]
                          n759 = invoke class="VI" method="FP.Close"(reference=w1020) -> (reference out=w1019:refnum<vi>)  [unwired: 2 in, 2 out]
                          n760 = Close Reference(reference=w1019) -> ()  [unwired: 1 in, 1 out]
                        }
                      }
                      frame #1 {
                        n761 = property on="数组 4" class="Arr (严格)"("Value"=refnum<vi>[] [] ("数组 4")) -> ()  [unwired: 2 in, 2 out]
                      }
                    }
                  }
                  frame "开始测量 2" {
                    n762 = flat-sequence {
                      frame #0 {
                        n763 = property on="数组 5" class="Arr (严格)"() -> ("Value"=w1023:refnum<vi>[])  [unwired: 2 in, 2 out]
                        n764 = for {
                          tunnel: w1023 -> [w1026] mode=indexing
                          n765 = invoke class="VI" method="Abort VI"(reference=w1026) -> (reference out=w1025:refnum<vi>)  [unwired: 2 in, 2 out]
                          n766 = invoke class="VI" method="FP.Close"(reference=w1025) -> (reference out=w1024:refnum<vi>)  [unwired: 2 in, 2 out]
                          n767 = Close Reference(reference=w1024) -> ()  [unwired: 1 in, 1 out]
                        }
                      }
                      frame #1 {
                        n768 = property on="数组 5" class="Arr (严格)"("Value"=refnum<vi>[] [] ("数组 5")) -> ()  [unwired: 2 in, 2 out]
                      }
                    }
                  }
                  frame "开始测量 3" {
                    n769 = flat-sequence {
                      frame #0 {
                        n770 = property on="数组 6" class="Arr (严格)"() -> ("Value"=w1028:refnum<vi>[])  [unwired: 2 in, 2 out]
                        n771 = for {
                          tunnel: w1028 -> [w1031] mode=indexing
                          n772 = invoke class="VI" method="Abort VI"(reference=w1031) -> (reference out=w1030:refnum<vi>)  [unwired: 2 in, 2 out]
                          n773 = invoke class="VI" method="FP.Close"(reference=w1030) -> (reference out=w1029:refnum<vi>)  [unwired: 2 in, 2 out]
                          n774 = Close Reference(reference=w1029) -> ()  [unwired: 1 in, 1 out]
                        }
                      }
                      frame #1 {
                        n775 = property on="数组 6" class="Arr (严格)"("Value"=refnum<vi>[] [] ("数组 6")) -> ()  [unwired: 2 in, 2 out]
                      }
                    }
                  }
                  frame "开始测量 4" {
                    n776 = flat-sequence {
                      frame #0 {
                        n777 = property on="数组 7" class="Arr (严格)"() -> ("Value"=w1033:refnum<vi>[])  [unwired: 2 in, 2 out]
                        n778 = for {
                          tunnel: w1033 -> [w1036] mode=indexing
                          n779 = invoke class="VI" method="Abort VI"(reference=w1036) -> (reference out=w1035:refnum<vi>)  [unwired: 2 in, 2 out]
                          n780 = invoke class="VI" method="FP.Close"(reference=w1035) -> (reference out=w1034:refnum<vi>)  [unwired: 2 in, 2 out]
                          n781 = Close Reference(reference=w1034) -> ()  [unwired: 1 in, 1 out]
                        }
                      }
                      frame #1 {
                        n782 = property on="数组 7" class="Arr (严格)"("Value"=refnum<vi>[] [] ("数组 7")) -> ()  [unwired: 2 in, 2 out]
                      }
                    }
                  }
                }
              }
              frame True {
                n783 = case shown="\"开始测量\", 默认" w1038 {
                  frame "开始测量", Default {
                    w1044 = "USB0::0x2EC7::0x3000::803489033757710017::INSTR"  # 用户名
                    n784 = control-ref of="温度显示"() -> (w1054:refnum<vi>)
                    n785 = control-ref of="水质1"() -> (w1055:refnum<vi>)
                    n786 = control-ref of="温度1"() -> (w1056:refnum<vi>)
                    n787 = control-ref of="所有数据"() -> (w1057:refnum<vi>)
                    n788 = control-ref of="数值"() -> (w1058:refnum<vi>)
                    n789 = control-ref of="极化曲线1"() -> (w1059:refnum<vi>)
                    n790 = control-ref of="极化电压1"() -> (w1060:refnum<vi>)
                    n791 = control-ref of="极化电流1"() -> (w1061:refnum<vi>)
                    n792 = control-ref of="电压1"() -> (w1062:refnum<vi>)
                    n793 = control-ref of="电流1"() -> (w1063:refnum<vi>)
                    n794 = property on="用户：" class="Str"() -> ("Value"=w1052:string)  [unwired: 2 in, 2 out]
                    n795 = property on="测试类型 2" class="Str"() -> ("Value"=w1051:string)  [unwired: 2 in, 2 out]
                    n796 = Bundle By Name(cluster=cluster{"用户名":string, "项目名称":string} {"用户名"="", "项目名称"=""}, "用户名"=w1052, "项目名称"=w1051) -> (w1050:cluster{"用户名":string, "项目名称":string})
                    n797 = control-ref of="压力1"() -> (w1040:refnum<vi>)
                    n798 = Bundle By Name(cluster=T11 {"所有数据"=refnum, "数值"=refnum, "极化曲线1"=refnum, "极化电压1"=refnum, "极化电流1"=refnum, "电压1"=refnum, "电流1"=refnum, "水质1"=refnum, "温度1"=refnum, "温度显示"=refnum, "压力1"=refnum}, "所有数据"=w1057, "数值"=w1058, "极化曲线1"=w1059, "极化电压1"=w1060, "极化电流1"=w1061, "电压1"=w1062, "电流1"=w1063, "水质1"=w1055, "温度1"=w1056, "温度显示"=w1054, "压力1"=w1040) -> (w1039:T11)
                    n799 = Open VI Reference(type specifier VI Refnum (for type only)=refnum<vi> refnum ("类型说明符VI引用句柄（仅用于类型）"), vi path=path "C:/Users/526computer/Desktop/2022 - 副本/pem/电源函数/输出调用01.vi" ("VI路径"), options=128 ("选项")) -> (vi reference=w1053:refnum<vi>)  [unwired: 3 in, 1 out]
                    n800 = call-by-ref "开始异步调用"(reference=w1053, "输出簇"=w1050, "数组"=string[][] [["1", "CC", "15", "0.95", "1700", "20"], ["2", "CC", "15", "2.15", "1700", "20"], ["3", "CC", "15", "3.35", "1700", "20"], ["4", "CC", "15", "4.55", "1700", "20"], ["5", "CC", "15", "5.75", "1700", "20"], ["6", "CC", "15", "6.95", "1700", "20"], ["7", "CC", "15", "8.15", "1700", "20"], ["8", "CC", "15", "9.35", "1700", "20"], ["9", "CC", "15", "10.55", "1700", "20"], ["10", "CC", "15", "11.75", "1700", "20"], ["11", "CC", "15", "12.95", "1700", "20"], ["12", "CC", "15", "14.15", "1700", "20"], ["13", "CC", "15", "15.35", "1700", "20"], ["14", "CC", "15", "16.55", "1700", "20"], ["15", "CC", "15", "17.75", "1700", "20"], ["16", "CC", "15", "18.95", "1700", "180"], ["17", "CC", "15", "20.15", "1700", "180"], ["18", "CC", "15", "21.35", "1700", "180"], ["19", "CC", "15", "22.55", "1700", "180"], ["20", "CC", "15", "23.75", "1700", "180"], ["21", "CC", "15", "24.95", "1700", "180"], ["22", "CC", "15", "26.15", "1700", "180"], ["23", "CC", "15", "27.35", "1700", "180"], ["24", "CC", "15", "28.55", "1700", "180"], ["25", "CC", "15", "29.75", "1700", "180"], ["26", "CC", "15", "30.95", "1700", "180"], ["27", "CC", "15", "32.15", "1700", "180"], ["28", "CC", "15", "33.35", "1700", "180"], ["29", "CC", "15", "34.55", "1700", "180"], ["30", "CC", "15", "35.75", "1700", "180"], ["31", "CC", "15", "36.95", "1700", "180"], ["32", "CC", "15", "38.15", "1700", "180"], ["33", "CC", "15", "39.35", "1700", "180"], ["34", "CC", "15", "40.55", "1700", "180"], ["35", "CC", "15", "41.75", "1700", "180"], ["36", "CC", "15", "42.95", "1700", "180"], ["37", "CC", "15", "44.15", "1700", "180"], ["38", "CC", "15", "45.35", "1700", "180"], ["39", "CC", "15", "46.55", "1700", "180"], ["40", "CC", "15", "47.75", "1700", "180"], ["41", "CC", "15", "48.95", "1700", "180"], ["42", "CC", "15", "50.15", "1700", "180"], ["43", "CC", "15", "51.35", "1700", "180"], ["44", "CC", "15", "52.55", "1700", "180"], ["45", "CC", "15", "53.75", "1700", "180"], ["46", "CC", "15", "54.95", "1700", "180"], ["47", "CC", "15", "56.15", "1700", "180"], ["48", "CC", "15", "57.35", "1700", "180"], ["49", "CC", "15", "58.55", "1700", "180"], ["50", "CC", "15", "59.75", "1700", "180"], ["51", "CC", "15", "60.95", "1700", "180"], ["52", "CC", "15", "62.15", "1700", "180"], ["53", "CC", "15", "63.35", "1700", "180"], ["54", "CC", "15", "64.55", "1700", "180"], ["55", "CC", "15", "65.75", "1700", "180"], ["56", "CC", "15", "66.95", "1700", "180"], ["57", "CC", "15", "68.15", "1700", "180"], ["58", "CC", "15", "69.35", "1700", "180"], ["59", "CC", "15", "70.55", "1700", "180"], ["60", "CC", "15", "71.75", "1700", "180"], ["61", "CC", "15", "72.95", "1700", "180"], ["62", "CC", "15", "74.15", "1700", "180"], ["63", "CC", "15", "75.35", "1700", "180"], ["64", "CC", "15", "76.55", "1700", "180"], ["65", "CC", "15", "77.75", "1700", "180"], ["66", "CC", "15", "78.95", "1700", "180"], ["67", "CC", "15", "80.15", "1700", "180"], ["68", "CC", "15", "81.35", "1700", "180"], ["69", "CC", "15", "82.55", "1700", "180"], ["70", "CC", "15", "83.75", "1700", "180"], ["71", "CC", "15", "84.95", "1700", "180"], ["72", "CC", "15", "86.15", "1700", "180"], ["73", "CC", "15", "87.35", "1700", "180"], ["74", "CC", "15", "88.55", "1700", "180"], ["75", "CC", "15", "89.75", "1700", "180"], ["76", "CC", "15", "90.95", "1700", "180"], ["77", "CC", "15", "92.15", "1700", "180"], ["78", "CC", "15", "93.35", "1700", "180"], ["79", "CC", "15", "94.55", "1700", "180"], ["80", "CC", "15", "95.75", "1700", "180"], ["81", "CC", "15", "96.95", "1700", "180"], ["82", "CC", "15", "98.15", "1700", "180"], ["83", "CC", "15", "99.35", "1700", "180"], ["84", "CC", "15", "100.55", "1700", "180"], [" ", " ", " ", " ", " ", " "]] ("已删除元素的数组子集"), "字符串"=w1044, "输出簇 2"=w1039) -> (reference out=w1047:refnum<vi>)  [unwired: 13 in, 1 out]
                    n801 = property on="数组 4" class="Arr (严格)"() -> ("Value"=w1049:refnum<vi>[])  [unwired: 2 in, 2 out]
                    n802 = Insert Into Array(array=w1049, new element=w1047) -> (w1048:refnum<vi>[])  [unwired: 1 in]
                    n803 = property on="数组 4" class="Arr (严格)"("Value"=w1048) -> ()  [unwired: 2 in, 2 out]
                  }
                  frame "开始测量 2" {
                    w1083 = "USB0::0x2EC7::0x3000::803490033757710003::INSTR"  # 用户名
                    n804 = property on="用户：" class="Str"() -> ("Value"=w1087:string)  [unwired: 2 in, 2 out]
                    n805 = property on="测试类型 2" class="Str"() -> ("Value"=w1086:string)  [unwired: 2 in, 2 out]
                    n806 = Bundle By Name(cluster=cluster{"用户名":string, "项目名称":string} {"用户名"="", "项目名称"=""}, "用户名"=w1087, "项目名称"=w1086) -> (w1082:cluster{"用户名":string, "项目名称":string})
                    n807 = control-ref of="电流2"() -> (w1069:refnum<vi>)
                    n808 = control-ref of="电压2"() -> (w1070:refnum<vi>)
                    n809 = control-ref of="极化电流2"() -> (w1071:refnum<vi>)
                    n810 = control-ref of="极化曲线2"() -> (w1073:refnum<vi>)
                    n811 = control-ref of="极化电压2"() -> (w1072:refnum<vi>)
                    n812 = control-ref of="数值 2"() -> (w1074:refnum<vi>)
                    n813 = control-ref of="所有数据2"() -> (w1075:refnum<vi>)
                    n814 = control-ref of="水质2"() -> (w1078:refnum<vi>)
                    n815 = control-ref of="温度2"() -> (w1077:refnum<vi>)
                    n816 = control-ref of="温度显示 2"() -> (w1076:refnum<vi>)
                    n817 = control-ref of="压力2"() -> (w1065:refnum<vi>)
                    n818 = Bundle By Name(cluster=T12 {"水质2"=refnum, "温度2"=refnum, "温度显示 2"=refnum, "所有数据2"=refnum, "数值 2"=refnum, "极化曲线2"=refnum, "极化电压2"=refnum, "极化电流2"=refnum, "电压2"=refnum, "电流2"=refnum, "压力2"=refnum}, "水质2"=w1078, "温度2"=w1077, "温度显示 2"=w1076, "所有数据2"=w1075, "数值 2"=w1074, "极化曲线2"=w1073, "极化电压2"=w1072, "极化电流2"=w1071, "电压2"=w1070, "电流2"=w1069, "压力2"=w1065) -> (w1068:T12)
                    n819 = Open VI Reference(type specifier VI Refnum (for type only)=refnum<vi> refnum ("类型说明符VI引用句柄（仅用于类型）"), vi path=path "C:/Users/526computer/Desktop/2022 - 副本/pem/电源函数/输出调用02.vi" ("VI路径"), options=128 ("选项")) -> (vi reference=w1090:refnum<vi>)  [unwired: 3 in, 1 out]
                    n820 = call-by-ref "开始异步调用"(reference=w1090, "输出簇"=w1082, "数组"=string[][] [["1", "CC", "15", "0.95", "1700", "20"], ["2", "CC", "15", "2.15", "1700", "20"], ["3", "CC", "15", "3.35", "1700", "20"], ["4", "CC", "15", "4.55", "1700", "20"], ["5", "CC", "15", "5.75", "1700", "20"], ["6", "CC", "15", "6.95", "1700", "20"], ["7", "CC", "15", "8.15", "1700", "20"], ["8", "CC", "15", "9.35", "1700", "20"], ["9", "CC", "15", "10.55", "1700", "20"], ["10", "CC", "15", "11.75", "1700", "20"], ["11", "CC", "15", "12.95", "1700", "20"], ["12", "CC", "15", "14.15", "1700", "20"], ["13", "CC", "15", "15.35", "1700", "20"], ["14", "CC", "15", "16.55", "1700", "20"], ["15", "CC", "15", "17.75", "1700", "20"], ["16", "CC", "15", "18.95", "1700", "180"], ["17", "CC", "15", "20.15", "1700", "180"], ["18", "CC", "15", "21.35", "1700", "180"], ["19", "CC", "15", "22.55", "1700", "180"], ["20", "CC", "15", "23.75", "1700", "180"], ["21", "CC", "15", "24.95", "1700", "180"], ["22", "CC", "15", "26.15", "1700", "180"], ["23", "CC", "15", "27.35", "1700", "180"], ["24", "CC", "15", "28.55", "1700", "180"], ["25", "CC", "15", "29.75", "1700", "180"], ["26", "CC", "15", "30.95", "1700", "180"], ["27", "CC", "15", "32.15", "1700", "180"], ["28", "CC", "15", "33.35", "1700", "180"], ["29", "CC", "15", "34.55", "1700", "180"], ["30", "CC", "15", "35.75", "1700", "180"], ["31", "CC", "15", "36.95", "1700", "180"], ["32", "CC", "15", "38.15", "1700", "180"], ["33", "CC", "15", "39.35", "1700", "180"], ["34", "CC", "15", "40.55", "1700", "180"], ["35", "CC", "15", "41.75", "1700", "180"], ["36", "CC", "15", "42.95", "1700", "180"], ["37", "CC", "15", "44.15", "1700", "180"], ["38", "CC", "15", "45.35", "1700", "180"], ["39", "CC", "15", "46.55", "1700", "180"], ["40", "CC", "15", "47.75", "1700", "180"], ["41", "CC", "15", "48.95", "1700", "180"], ["42", "CC", "15", "50.15", "1700", "180"], ["43", "CC", "15", "51.35", "1700", "180"], ["44", "CC", "15", "52.55", "1700", "180"], ["45", "CC", "15", "53.75", "1700", "180"], ["46", "CC", "15", "54.95", "1700", "180"], ["47", "CC", "15", "56.15", "1700", "180"], ["48", "CC", "15", "57.35", "1700", "180"], ["49", "CC", "15", "58.55", "1700", "180"], ["50", "CC", "15", "59.75", "1700", "180"], ["51", "CC", "15", "60.95", "1700", "180"], ["52", "CC", "15", "62.15", "1700", "180"], ["53", "CC", "15", "63.35", "1700", "180"], ["54", "CC", "15", "64.55", "1700", "180"], ["55", "CC", "15", "65.75", "1700", "180"], ["56", "CC", "15", "66.95", "1700", "180"], ["57", "CC", "15", "68.15", "1700", "180"], ["58", "CC", "15", "69.35", "1700", "180"], ["59", "CC", "15", "70.55", "1700", "180"], ["60", "CC", "15", "71.75", "1700", "180"], ["61", "CC", "15", "72.95", "1700", "180"], ["62", "CC", "15", "74.15", "1700", "180"], ["63", "CC", "15", "75.35", "1700", "180"], ["64", "CC", "15", "76.55", "1700", "180"], ["65", "CC", "15", "77.75", "1700", "180"], ["66", "CC", "15", "78.95", "1700", "180"], ["67", "CC", "15", "80.15", "1700", "180"], ["68", "CC", "15", "81.35", "1700", "180"], ["69", "CC", "15", "82.55", "1700", "180"], ["70", "CC", "15", "83.75", "1700", "180"], ["71", "CC", "15", "84.95", "1700", "180"], ["72", "CC", "15", "86.15", "1700", "180"], ["73", "CC", "15", "87.35", "1700", "180"], ["74", "CC", "15", "88.55", "1700", "180"], ["75", "CC", "15", "89.75", "1700", "180"], ["76", "CC", "15", "90.95", "1700", "180"], ["77", "CC", "15", "92.15", "1700", "180"], ["78", "CC", "15", "93.35", "1700", "180"], ["79", "CC", "15", "94.55", "1700", "180"], ["80", "CC", "15", "95.75", "1700", "180"], ["81", "CC", "15", "96.95", "1700", "180"], ["82", "CC", "15", "98.15", "1700", "180"], ["83", "CC", "15", "99.35", "1700", "180"], ["84", "CC", "15", "100.55", "1700", "180"], [" ", " ", " ", " ", " ", " "]] ("已删除元素的数组子集"), "字符串"=w1083, "输出簇 2"=w1068) -> (reference out=w1081:refnum<vi>)  [unwired: 13 in, 1 out]
                    n821 = property on="数组 5" class="Arr (严格)"() -> ("Value"=w1067:refnum<vi>[])  [unwired: 2 in, 2 out]
                    n822 = Insert Into Array(array=w1067, new element=w1081) -> (w1066:refnum<vi>[])  [unwired: 1 in]
                    n823 = property on="数组 5" class="Arr (严格)"("Value"=w1066) -> ()  [unwired: 2 in, 2 out]
                  }
                  frame "开始测量 3" {
                    w1110 = "USB0::0x2EC7::0x3000::803489033757710017::INSTR"  # 用户名
                    n824 = property on="用户：" class="Str"() -> ("Value"=w1106:string)  [unwired: 2 in, 2 out]
                    n825 = property on="测试类型 2" class="Str"() -> ("Value"=w1105:string)  [unwired: 2 in, 2 out]
                    n826 = control-ref of="水质3"() -> (w1104:refnum<vi>)
                    n827 = control-ref of="温度3"() -> (w1103:refnum<vi>)
                    n828 = control-ref of="温度显示 3"() -> (w1102:refnum<vi>)
                    n829 = control-ref of="所有数据3"() -> (w1101:refnum<vi>)
                    n830 = control-ref of="数值 3"() -> (w1100:refnum<vi>)
                    n831 = control-ref of="极化曲线3"() -> (w1099:refnum<vi>)
                    n832 = control-ref of="极化电压3"() -> (w1098:refnum<vi>)
                    n833 = control-ref of="极化电流3"() -> (w1097:refnum<vi>)
                    n834 = control-ref of="电压3"() -> (w1096:refnum<vi>)
                    n835 = control-ref of="电流3"() -> (w1095:refnum<vi>)
                    n836 = Bundle By Name(cluster=cluster{"用户名":string, "项目名称":string} {"用户名"="", "项目名称"=""}, "用户名"=w1106, "项目名称"=w1105) -> (w1114:cluster{"用户名":string, "项目名称":string})
                    n837 = control-ref of="压力3"() -> (w1091:refnum<vi>)
                    n838 = Bundle By Name(cluster=T13 {"水质3"=refnum, "温度3"=refnum, "温度显示 3"=refnum, "所有数据3"=refnum, "数值 3"=refnum, "极化曲线3"=refnum, "极化电压3"=refnum, "极化电流3"=refnum, "电压3"=refnum, "电流3"=refnum, "压力3"=refnum}, "水质3"=w1104, "温度3"=w1103, "温度显示 3"=w1102, "所有数据3"=w1101, "数值 3"=w1100, "极化曲线3"=w1099, "极化电压3"=w1098, "极化电流3"=w1097, "电压3"=w1096, "电流3"=w1095, "压力3"=w1091) -> (w1094:T13)
                    n839 = Open VI Reference(type specifier VI Refnum (for type only)=refnum<vi> refnum ("类型说明符VI引用句柄（仅用于类型）"), vi path=path "C:/Users/526computer/Desktop/2022 - 副本/pem/电源函数/输出调用03.vi" ("VI路径"), options=128 ("选项")) -> (vi reference=w1115:refnum<vi>)  [unwired: 3 in, 1 out]
                    n840 = property on="数组 6" class="Arr (严格)"() -> ("Value"=w1093:refnum<vi>[])  [unwired: 2 in, 2 out]
                    n841 = call-by-ref "开始异步调用"(reference=w1115, "输出簇"=w1114, "数组"=string[][] [["1", "CC", "15", "0.95", "1700", "20"], ["2", "CC", "15", "2.15", "1700", "20"], ["3", "CC", "15", "3.35", "1700", "20"], ["4", "CC", "15", "4.55", "1700", "20"], ["5", "CC", "15", "5.75", "1700", "20"], ["6", "CC", "15", "6.95", "1700", "20"], ["7", "CC", "15", "8.15", "1700", "20"], ["8", "CC", "15", "9.35", "1700", "20"], ["9", "CC", "15", "10.55", "1700", "20"], ["10", "CC", "15", "11.75", "1700", "20"], ["11", "CC", "15", "12.95", "1700", "20"], ["12", "CC", "15", "14.15", "1700", "20"], ["13", "CC", "15", "15.35", "1700", "20"], ["14", "CC", "15", "16.55", "1700", "20"], ["15", "CC", "15", "17.75", "1700", "20"], ["16", "CC", "15", "18.95", "1700", "180"], ["17", "CC", "15", "20.15", "1700", "180"], ["18", "CC", "15", "21.35", "1700", "180"], ["19", "CC", "15", "22.55", "1700", "180"], ["20", "CC", "15", "23.75", "1700", "180"], ["21", "CC", "15", "24.95", "1700", "180"], ["22", "CC", "15", "26.15", "1700", "180"], ["23", "CC", "15", "27.35", "1700", "180"], ["24", "CC", "15", "28.55", "1700", "180"], ["25", "CC", "15", "29.75", "1700", "180"], ["26", "CC", "15", "30.95", "1700", "180"], ["27", "CC", "15", "32.15", "1700", "180"], ["28", "CC", "15", "33.35", "1700", "180"], ["29", "CC", "15", "34.55", "1700", "180"], ["30", "CC", "15", "35.75", "1700", "180"], ["31", "CC", "15", "36.95", "1700", "180"], ["32", "CC", "15", "38.15", "1700", "180"], ["33", "CC", "15", "39.35", "1700", "180"], ["34", "CC", "15", "40.55", "1700", "180"], ["35", "CC", "15", "41.75", "1700", "180"], ["36", "CC", "15", "42.95", "1700", "180"], ["37", "CC", "15", "44.15", "1700", "180"], ["38", "CC", "15", "45.35", "1700", "180"], ["39", "CC", "15", "46.55", "1700", "180"], ["40", "CC", "15", "47.75", "1700", "180"], ["41", "CC", "15", "48.95", "1700", "180"], ["42", "CC", "15", "50.15", "1700", "180"], ["43", "CC", "15", "51.35", "1700", "180"], ["44", "CC", "15", "52.55", "1700", "180"], ["45", "CC", "15", "53.75", "1700", "180"], ["46", "CC", "15", "54.95", "1700", "180"], ["47", "CC", "15", "56.15", "1700", "180"], ["48", "CC", "15", "57.35", "1700", "180"], ["49", "CC", "15", "58.55", "1700", "180"], ["50", "CC", "15", "59.75", "1700", "180"], ["51", "CC", "15", "60.95", "1700", "180"], ["52", "CC", "15", "62.15", "1700", "180"], ["53", "CC", "15", "63.35", "1700", "180"], ["54", "CC", "15", "64.55", "1700", "180"], ["55", "CC", "15", "65.75", "1700", "180"], ["56", "CC", "15", "66.95", "1700", "180"], ["57", "CC", "15", "68.15", "1700", "180"], ["58", "CC", "15", "69.35", "1700", "180"], ["59", "CC", "15", "70.55", "1700", "180"], ["60", "CC", "15", "71.75", "1700", "180"], ["61", "CC", "15", "72.95", "1700", "180"], ["62", "CC", "15", "74.15", "1700", "180"], ["63", "CC", "15", "75.35", "1700", "180"], ["64", "CC", "15", "76.55", "1700", "180"], ["65", "CC", "15", "77.75", "1700", "180"], ["66", "CC", "15", "78.95", "1700", "180"], ["67", "CC", "15", "80.15", "1700", "180"], ["68", "CC", "15", "81.35", "1700", "180"], ["69", "CC", "15", "82.55", "1700", "180"], ["70", "CC", "15", "83.75", "1700", "180"], ["71", "CC", "15", "84.95", "1700", "180"], ["72", "CC", "15", "86.15", "1700", "180"], ["73", "CC", "15", "87.35", "1700", "180"], ["74", "CC", "15", "88.55", "1700", "180"], ["75", "CC", "15", "89.75", "1700", "180"], ["76", "CC", "15", "90.95", "1700", "180"], ["77", "CC", "15", "92.15", "1700", "180"], ["78", "CC", "15", "93.35", "1700", "180"], ["79", "CC", "15", "94.55", "1700", "180"], ["80", "CC", "15", "95.75", "1700", "180"], ["81", "CC", "15", "96.95", "1700", "180"], ["82", "CC", "15", "98.15", "1700", "180"], ["83", "CC", "15", "99.35", "1700", "180"], ["84", "CC", "15", "100.55", "1700", "180"], [" ", " ", " ", " ", " ", " "]] ("已删除元素的数组子集"), "字符串"=w1110, "输出簇 2"=w1094) -> (reference out=w1113:refnum<vi>)  [unwired: 13 in, 1 out]
                    n842 = Insert Into Array(array=w1093, new element=w1113) -> (w1092:refnum<vi>[])  [unwired: 1 in]
                    n843 = property on="数组 6" class="Arr (严格)"("Value"=w1092) -> ()  [unwired: 2 in, 2 out]
                  }
                  frame "开始测量 4" {
                    w1136 = "USB0::0x2EC7::0x3000::803489033757710017::INSTR"  # 用户名
                    n844 = control-ref of="水质4"() -> (w1130:refnum<vi>)
                    n845 = control-ref of="温度4"() -> (w1129:refnum<vi>)
                    n846 = control-ref of="温度显示 4"() -> (w1128:refnum<vi>)
                    n847 = control-ref of="所有数据4"() -> (w1127:refnum<vi>)
                    n848 = control-ref of="数值 4"() -> (w1126:refnum<vi>)
                    n849 = control-ref of="极化曲线4"() -> (w1125:refnum<vi>)
                    n850 = control-ref of="极化电压4"() -> (w1124:refnum<vi>)
                    n851 = control-ref of="极化电流4"() -> (w1123:refnum<vi>)
                    n852 = control-ref of="电压4"() -> (w1122:refnum<vi>)
                    n853 = control-ref of="电流4"() -> (w1121:refnum<vi>)
                    n854 = property on="用户：" class="Str"() -> ("Value"=w1132:string)  [unwired: 2 in, 2 out]
                    n855 = property on="测试类型 2" class="Str"() -> ("Value"=w1131:string)  [unwired: 2 in, 2 out]
                    n856 = Bundle By Name(cluster=cluster{"用户名":string, "项目名称":string} {"用户名"="", "项目名称"=""}, "用户名"=w1132, "项目名称"=w1131) -> (w1140:cluster{"用户名":string, "项目名称":string})
                    n857 = control-ref of="压力4"() -> (w1117:refnum<vi>)
                    n858 = Bundle By Name(cluster=T14 {"水质4"=refnum, "温度4"=refnum, "温度显示 4"=refnum, "所有数据4"=refnum, "数值 4"=refnum, "极化曲线4"=refnum, "极化电压4"=refnum, "极化电流4"=refnum, "电压4"=refnum, "电流4"=refnum, "压力4"=refnum}, "水质4"=w1130, "温度4"=w1129, "温度显示 4"=w1128, "所有数据4"=w1127, "数值 4"=w1126, "极化曲线4"=w1125, "极化电压4"=w1124, "极化电流4"=w1123, "电压4"=w1122, "电流4"=w1121, "压力4"=w1117) -> (w1120:T14)
                    n859 = Open VI Reference(type specifier VI Refnum (for type only)=refnum<vi> refnum ("类型说明符VI引用句柄（仅用于类型）"), vi path=path "C:/Users/526computer/Desktop/2022 - 副本/pem/电源函数/输出调用04.vi" ("VI路径"), options=128 ("选项")) -> (vi reference=w1141:refnum<vi>)  [unwired: 3 in, 1 out]
                    n860 = property on="数组 7" class="Arr (严格)"() -> ("Value"=w1119:refnum<vi>[])  [unwired: 2 in, 2 out]
                    n861 = call-by-ref "开始异步调用"(reference=w1141, "输出簇"=w1140, "数组"=string[][] [["1", "CC", "15", "0.95", "1700", "20"], ["2", "CC", "15", "2.15", "1700", "20"], ["3", "CC", "15", "3.35", "1700", "20"], ["4", "CC", "15", "4.55", "1700", "20"], ["5", "CC", "15", "5.75", "1700", "20"], ["6", "CC", "15", "6.95", "1700", "20"], ["7", "CC", "15", "8.15", "1700", "20"], ["8", "CC", "15", "9.35", "1700", "20"], ["9", "CC", "15", "10.55", "1700", "20"], ["10", "CC", "15", "11.75", "1700", "20"], ["11", "CC", "15", "12.95", "1700", "20"], ["12", "CC", "15", "14.15", "1700", "20"], ["13", "CC", "15", "15.35", "1700", "20"], ["14", "CC", "15", "16.55", "1700", "20"], ["15", "CC", "15", "17.75", "1700", "20"], ["16", "CC", "15", "18.95", "1700", "180"], ["17", "CC", "15", "20.15", "1700", "180"], ["18", "CC", "15", "21.35", "1700", "180"], ["19", "CC", "15", "22.55", "1700", "180"], ["20", "CC", "15", "23.75", "1700", "180"], ["21", "CC", "15", "24.95", "1700", "180"], ["22", "CC", "15", "26.15", "1700", "180"], ["23", "CC", "15", "27.35", "1700", "180"], ["24", "CC", "15", "28.55", "1700", "180"], ["25", "CC", "15", "29.75", "1700", "180"], ["26", "CC", "15", "30.95", "1700", "180"], ["27", "CC", "15", "32.15", "1700", "180"], ["28", "CC", "15", "33.35", "1700", "180"], ["29", "CC", "15", "34.55", "1700", "180"], ["30", "CC", "15", "35.75", "1700", "180"], ["31", "CC", "15", "36.95", "1700", "180"], ["32", "CC", "15", "38.15", "1700", "180"], ["33", "CC", "15", "39.35", "1700", "180"], ["34", "CC", "15", "40.55", "1700", "180"], ["35", "CC", "15", "41.75", "1700", "180"], ["36", "CC", "15", "42.95", "1700", "180"], ["37", "CC", "15", "44.15", "1700", "180"], ["38", "CC", "15", "45.35", "1700", "180"], ["39", "CC", "15", "46.55", "1700", "180"], ["40", "CC", "15", "47.75", "1700", "180"], ["41", "CC", "15", "48.95", "1700", "180"], ["42", "CC", "15", "50.15", "1700", "180"], ["43", "CC", "15", "51.35", "1700", "180"], ["44", "CC", "15", "52.55", "1700", "180"], ["45", "CC", "15", "53.75", "1700", "180"], ["46", "CC", "15", "54.95", "1700", "180"], ["47", "CC", "15", "56.15", "1700", "180"], ["48", "CC", "15", "57.35", "1700", "180"], ["49", "CC", "15", "58.55", "1700", "180"], ["50", "CC", "15", "59.75", "1700", "180"], ["51", "CC", "15", "60.95", "1700", "180"], ["52", "CC", "15", "62.15", "1700", "180"], ["53", "CC", "15", "63.35", "1700", "180"], ["54", "CC", "15", "64.55", "1700", "180"], ["55", "CC", "15", "65.75", "1700", "180"], ["56", "CC", "15", "66.95", "1700", "180"], ["57", "CC", "15", "68.15", "1700", "180"], ["58", "CC", "15", "69.35", "1700", "180"], ["59", "CC", "15", "70.55", "1700", "180"], ["60", "CC", "15", "71.75", "1700", "180"], ["61", "CC", "15", "72.95", "1700", "180"], ["62", "CC", "15", "74.15", "1700", "180"], ["63", "CC", "15", "75.35", "1700", "180"], ["64", "CC", "15", "76.55", "1700", "180"], ["65", "CC", "15", "77.75", "1700", "180"], ["66", "CC", "15", "78.95", "1700", "180"], ["67", "CC", "15", "80.15", "1700", "180"], ["68", "CC", "15", "81.35", "1700", "180"], ["69", "CC", "15", "82.55", "1700", "180"], ["70", "CC", "15", "83.75", "1700", "180"], ["71", "CC", "15", "84.95", "1700", "180"], ["72", "CC", "15", "86.15", "1700", "180"], ["73", "CC", "15", "87.35", "1700", "180"], ["74", "CC", "15", "88.55", "1700", "180"], ["75", "CC", "15", "89.75", "1700", "180"], ["76", "CC", "15", "90.95", "1700", "180"], ["77", "CC", "15", "92.15", "1700", "180"], ["78", "CC", "15", "93.35", "1700", "180"], ["79", "CC", "15", "94.55", "1700", "180"], ["80", "CC", "15", "95.75", "1700", "180"], ["81", "CC", "15", "96.95", "1700", "180"], ["82", "CC", "15", "98.15", "1700", "180"], ["83", "CC", "15", "99.35", "1700", "180"], ["84", "CC", "15", "100.55", "1700", "180"], [" ", " ", " ", " ", " ", " "]] ("已删除元素的数组子集"), "字符串"=w1136, "输出簇 2"=w1120) -> (reference out=w1139:refnum<vi>)  [unwired: 13 in, 1 out]
                    n862 = Insert Into Array(array=w1119, new element=w1139) -> (w1118:refnum<vi>[])  [unwired: 1 in]
                    n863 = property on="数组 7" class="Arr (严格)"("Value"=w1118) -> ()  [unwired: 2 in, 2 out]
                  }
                }
              }
            }
          }
          frame "耐久性曲线" {
            n864 = case shown="真" w1144 {
              tunnel: w1143 -> [w1145 w1151]
              frame False {
                n865 = case shown="\"开始测量\", 默认" w1145 {
                  frame "开始测量", Default {
                    n866 = flat-sequence {
                      frame #0 {
                        n867 = property on="数组 4" class="Arr (严格)"() -> ("Value"=w1146:refnum<vi>[])  [unwired: 2 in, 2 out]
                        n868 = for {
                          tunnel: w1146 -> [w1149] mode=indexing
                          n869 = invoke class="VI" method="Abort VI"(reference=w1149) -> (reference out=w1148:refnum<vi>)  [unwired: 2 in, 2 out]
                          n870 = invoke class="VI" method="FP.Close"(reference=w1148) -> (reference out=w1147:refnum<vi>)  [unwired: 2 in, 2 out]
                          n871 = Close Reference(reference=w1147) -> ()  [unwired: 1 in, 1 out]
                        }
                      }
                      frame #1 {
                        n872 = property on="数组 4" class="Arr (严格)"("Value"=refnum<vi>[] [] ("数组 9")) -> ()  [unwired: 2 in, 2 out]
                      }
                    }
                  }
                  frame "开始测量 2" {
                  }
                  frame "开始测量 3" {
                  }
                  frame "开始测量 4" {
                  }
                }
              }
              frame True {
                n873 = case shown="\"开始测量\", 默认" w1151 {
                  frame "开始测量", Default {
                    w1161 = "USB0::0x2EC7::0x3000::803489033757710017::INSTR"  # 用户名
                    n874 = property on="施加电流(A):" class="DigNum (严格)"() -> ("Value"=w1164:dbl)  [unwired: 2 in, 2 out]
                    n875 = property on="测试时长(H):" class="DigNum (严格)"() -> ("Value"=w1163:dbl)  [unwired: 2 in, 2 out]
                    n876 = control-ref of="电压1"() -> (w1154:refnum<vi>)
                    n877 = control-ref of="电流1"() -> (w1153:refnum<vi>)
                    n878 = Bundle By Name(cluster=cluster{"电压1":refnum<vi>, "电流1":refnum<vi>} {"电压1"=refnum, "电流1"=refnum}, "电压1"=w1154, "电流1"=w1153) -> (w1152:cluster{"电压1":refnum<vi>, "电流1":refnum<vi>})
                    n879 = Open VI Reference(type specifier VI Refnum (for type only)=refnum<vi> refnum ("类型说明符VI引用句柄（仅用于类型）"), vi path=path "C:/Users/526computer/Desktop/2022 - 副本/pem/电源函数/耐久性测试输出调用01.vi" ("VI路径"), options=128 ("选项")) -> (vi reference=w1165:refnum<vi>)  [unwired: 3 in, 1 out]
                    n880 = call-by-ref "开始异步调用"(reference=w1165, "电流"=w1164, "时长"=w1163, "字符串"=w1161, "输出簇"=w1152) -> (reference out=w1162:refnum<vi>)  [unwired: 13 in, 1 out]
                    n881 = property on="数组 4" class="Arr (严格)"() -> ("Value"=w1156:refnum<vi>[])  [unwired: 2 in, 2 out]
                    n882 = Insert Into Array(array=w1156, new element=w1162) -> (w1157:refnum<vi>[])  [unwired: 1 in]
                    n883 = property on="数组 4" class="Arr (严格)"("Value"=w1157) -> ()  [unwired: 2 in, 2 out]
                  }
                  frame "开始测量 2" {
                  }
                  frame "开始测量 3" {
                  }
                  frame "开始测量 4" {
                  }
                }
              }
            }
          }
          frame "线性扫描" {
          }
        }
      }
      event "测试项目": Value Change {
        n884 = event-data() -> ("NewVal"=w1166:enum32{"EIS", "极化曲线", "耐久性曲线", "线性扫描"})  [unwired: 1 in, 5 out]
        n885 = case shown="\"EIS\", 默认" w1166 {
          frame "EIS", Default {
            n886 = flat-sequence {
              frame #0 {
                n887 = property on="测试项目 2" class="TabCtl (严格)"("Value"=enum32{"极化曲线", "耐久性测试", "EIS"}."EIS" ("测试项目 2")) -> ()  [unwired: 2 in, 2 out]
              }
              frame #1 {
                w1168 = T2."Disabled and Grayed Out" ("禁用")
                n888 = property on="连接" class="Bool (严格)"("DisabledEnum"=w1168) -> ()  [unwired: 2 in, 2 out]
                n889 = property on="保存所有" class="Bool (严格)"("DisabledEnum"=w1168) -> ()  [unwired: 2 in, 2 out]
                n890 = property on="配置" class="Bool (严格)"("DisabledEnum"=w1168) -> ()  [unwired: 2 in, 2 out]
                n891 = property on="分析" class="Bool (严格)"("DisabledEnum"=w1168) -> ()  [unwired: 2 in, 2 out]
                n892 = property on="3" class="Bool (严格)"("DisabledEnum"=w1168) -> ()  [unwired: 2 in, 2 out]
                n893 = property on="4" class="Bool (严格)"("DisabledEnum"=w1168) -> ()  [unwired: 2 in, 2 out]
                n894 = property on="2" class="Bool (严格)"("DisabledEnum"=w1168) -> ()  [unwired: 2 in, 2 out]
                n895 = property on="通道选择" class="RadioBtnsControl (严格)"("DisabledEnum"=w1168) -> ()  [unwired: 2 in, 2 out]
              }
            }
          }
          frame "极化曲线" {
            n896 = flat-sequence {
              frame #0 {
                n897 = property on="测试项目 2" class="TabCtl (严格)"("Value"=enum32{"极化曲线", "耐久性测试"}."极化曲线" ("测试项目 2")) -> ()  [unwired: 2 in, 2 out]
              }
              frame #1 {
                w1170 = T2."Enabled" ("禁用")
                n898 = property on="连接" class="Bool (严格)"("DisabledEnum"=w1170) -> ()  [unwired: 2 in, 2 out]
                n899 = property on="保存所有" class="Bool (严格)"("DisabledEnum"=w1170) -> ()  [unwired: 2 in, 2 out]
                n900 = property on="配置" class="Bool (严格)"("DisabledEnum"=w1170) -> ()  [unwired: 2 in, 2 out]
                n901 = property on="分析" class="Bool (严格)"("DisabledEnum"=w1170) -> ()  [unwired: 2 in, 2 out]
                n902 = property on="3" class="Bool (严格)"("DisabledEnum"=w1170) -> ()  [unwired: 2 in, 2 out]
                n903 = property on="4" class="Bool (严格)"("DisabledEnum"=w1170) -> ()  [unwired: 2 in, 2 out]
                n904 = property on="2" class="Bool (严格)"("DisabledEnum"=w1170) -> ()  [unwired: 2 in, 2 out]
                n905 = property on="通道选择" class="RadioBtnsControl (严格)"("DisabledEnum"=w1170) -> ()  [unwired: 2 in, 2 out]
              }
            }
          }
          frame "耐久性曲线" {
            n906 = flat-sequence {
              frame #0 {
                n907 = property on="测试项目 2" class="TabCtl (严格)"("Value"=enum32{"极化曲线", "耐久性测试"}."耐久性测试" ("测试项目 2")) -> ()  [unwired: 2 in, 2 out]
              }
              frame #1 {
                w1172 = T2."Enabled" ("禁用")
                n908 = property on="连接" class="Bool (严格)"("DisabledEnum"=w1172) -> ()  [unwired: 2 in, 2 out]
                n909 = property on="保存所有" class="Bool (严格)"("DisabledEnum"=w1172) -> ()  [unwired: 2 in, 2 out]
                n910 = property on="配置" class="Bool (严格)"("DisabledEnum"=w1172) -> ()  [unwired: 2 in, 2 out]
                n911 = property on="分析" class="Bool (严格)"("DisabledEnum"=w1172) -> ()  [unwired: 2 in, 2 out]
                n912 = property on="3" class="Bool (严格)"("DisabledEnum"=w1172) -> ()  [unwired: 2 in, 2 out]
                n913 = property on="4" class="Bool (严格)"("DisabledEnum"=w1172) -> ()  [unwired: 2 in, 2 out]
                n914 = property on="2" class="Bool (严格)"("DisabledEnum"=w1172) -> ()  [unwired: 2 in, 2 out]
                n915 = property on="通道选择" class="RadioBtnsControl (严格)"("DisabledEnum"=w1172) -> ()  [unwired: 2 in, 2 out]
              }
            }
          }
        }
      }
      event "重排所有视图": Value Change {
        n916 = event-data() -> ()  [unwired: 1 in, 6 out]
        n917 = stacked-sequence {
          frame #0 {
            n918 = for {
              tunnel: "数组 3" -> [w1177] mode=indexing
              n919 = property class="VI"(reference=w1177) -> (reference out=w1174:refnum<vi>, "Front Panel.Title"=w1178:string)  [unwired: 1 in, 1 out]
              n920 = Wait (ms)(milliseconds to wait=u32 100 ("等待时间（毫秒）")) -> ()  [unwired: 1 out]
              n921 = flat-sequence {
                tunnel: w1178 -> [w1181]
                tunnel: [w1181] -> w1175
                tunnel: w1174 -> [w1180]
                tunnel: w1175 -> [w1190]
                frame #0 {
                  n922 = property class="VI"(reference=w1180, "FP.State"=T15."Standard" ("前面板窗口:状态")) -> ()  [unwired: 1 in, 2 out]
                }
                frame #1 {
                  n923 = case shown="\"工步列表\"" w1190 {
                    tunnel: ["" ("winname") "极化曲线" ("winname") "温度" ("winname") "压力" ("winname") "列表" ("winname") "工步列表" ("winname")] -> w1188
                    tunnel: [_ 729 1310 728 126 126] -> w1186
                    tunnel: [_ 192 568 568 192 568] -> w1182
                    tunnel: [_ 1163 583 582 604 604] -> w1183
                    tunnel: [_ 376 364 364 376 365] -> w1184
                    frame "假", Default {
                    }
                    frame "极化曲线" {
                    }
                    frame "温度" {
                    }
                    frame "压力" {
                    }
                    frame "列表" {
                    }
                    frame "工步列表" {
                      # "left:126,top:568,right:729,bottom:933"
                    }
                  }
                  n924 = dll-call lib="C:/Users/526computer/Desktop/LABVIEW.dll" fn="findlabview"("lpcallsname"=0, "winname"=w1188, "layer"=-1, "x"=w1186, "y"=w1182, "cx"=w1183, "cy"=w1184, "flag"=4) -> ()  [unwired: 12 in, 2 out]
                }
                frame #2 {
                }
              }
            }
          }
          frame #1 {
            n925 = property on="重排所有视图" class="Bool (严格)"("Value"=TRUE ("重排所有视图")) -> ()  [unwired: 2 in, 2 out]
          }
        }
      }
      event Panel Close? {
        n926 = event-data() -> ()  [unwired: 1 in, 4 out]
        n927 = flat-sequence {
          tunnel: [w1232] -> w1219
          tunnel: w1219 -> [w1234]
          tunnel: [w1234] -> w1218
          tunnel: w1218 -> [w1236]
          frame #0 {
            n928 = property on="数组 4" class="Arr (严格)"() -> ("Value"=w1223:refnum<vi>[])  [unwired: 2 in, 2 out]
            n929 = property on="数组 7" class="Arr (严格)"() -> ("Value"=w1220:refnum<vi>[])  [unwired: 2 in, 2 out]
            n930 = property on="数组 6" class="Arr (严格)"() -> ("Value"=w1221:refnum<vi>[])  [unwired: 2 in, 2 out]
            n931 = property on="数组 5" class="Arr (严格)"() -> ("Value"=w1222:refnum<vi>[])  [unwired: 2 in, 2 out]
            n932 = for {
              tunnel: w1223 -> [w1231] mode=indexing
              n933 = invoke class="VI" method="Abort VI"(reference=w1231) -> (reference out=w1230:refnum<vi>)  [unwired: 2 in, 2 out]
              n934 = invoke class="VI" method="FP.Close"(reference=w1230) -> ()  [unwired: 2 in, 3 out]
            }
            n935 = for {
              tunnel: w1222 -> [w1229] mode=indexing
              n936 = invoke class="VI" method="Abort VI"(reference=w1229) -> (reference out=w1228:refnum<vi>)  [unwired: 2 in, 2 out]
              n937 = invoke class="VI" method="FP.Close"(reference=w1228) -> ()  [unwired: 2 in, 3 out]
            }
            n938 = for {
              tunnel: w1220 -> [w1225] mode=indexing
              n939 = invoke class="VI" method="Abort VI"(reference=w1225) -> (reference out=w1224:refnum<vi>)  [unwired: 2 in, 2 out]
              n940 = invoke class="VI" method="FP.Close"(reference=w1224) -> ()  [unwired: 2 in, 3 out]
            }
            n941 = for {
              tunnel: w1221 -> [w1227] mode=indexing
              n942 = invoke class="VI" method="Abort VI"(reference=w1227) -> (reference out=w1226:refnum<vi>)  [unwired: 2 in, 2 out]
              n943 = invoke class="VI" method="FP.Close"(reference=w1226) -> ()  [unwired: 2 in, 3 out]
            }
          }
          frame #1 {
            n944 = property on="数组 3" class="Arr (严格)"() -> ("Value"=w1232:refnum<vi>[])  [unwired: 2 in, 2 out]
            n945 = for {
              tunnel: w1232 -> [w1233] mode=indexing
              n946 = invoke class="VI" method="Abort VI"(reference=w1233) -> ()  [unwired: 2 in, 3 out]
            }
          }
          frame #2 {
            n947 = for {
              tunnel: w1234 -> [w1235] mode=indexing
              n948 = invoke class="VI" method="FP.Close"(reference=w1235) -> ()  [unwired: 2 in, 3 out]
            }
          }
          frame #3 {
            n949 = for {
              tunnel: w1236 -> [w1237] mode=indexing
              n950 = Close Reference(reference=w1237) -> ()  [unwired: 1 in, 1 out]
            }
          }
          frame #4 {
            n951 = Stop(stop? (T)=TRUE ("停止？(T)")) -> ()
          }
        }
        n952 = event-data() -> ()  [unwired: 2 in, 1 out]
      }
      event "通道选择 2": Value Change {
        n953 = event-data() -> ("NewVal"=w1239:enum32{"未选择", "A1", "A2", "A3", "A4"})  [unwired: 1 in, 5 out]
        n954 = case shown="\"A1\", 默认" w1239 {
          frame "A1", Default {
            n955 = property on="开始测量 4" class="Bool (严格)"("Visible"=FALSE ("可见")) -> ()  [unwired: 2 in, 2 out]
            n956 = property on="开始测量 3" class="Bool (严格)"("Visible"=FALSE ("可见")) -> ()  [unwired: 2 in, 2 out]
            n957 = property on="开始测量" class="Bool (严格)"("Visible"=TRUE ("可见")) -> ()  [unwired: 2 in, 2 out]
            n958 = property on="开始测量 2" class="Bool (严格)"("Visible"=FALSE ("可见")) -> ()  [unwired: 2 in, 2 out]
          }
          frame "A2" {
            n959 = property on="开始测量 4" class="Bool (严格)"("Visible"=FALSE ("可见")) -> ()  [unwired: 2 in, 2 out]
            n960 = property on="开始测量 3" class="Bool (严格)"("Visible"=FALSE ("可见")) -> ()  [unwired: 2 in, 2 out]
            n961 = property on="开始测量" class="Bool (严格)"("Visible"=FALSE ("可见")) -> ()  [unwired: 2 in, 2 out]
            n962 = property on="开始测量 2" class="Bool (严格)"("Visible"=TRUE ("可见")) -> ()  [unwired: 2 in, 2 out]
          }
          frame "A3" {
            n963 = property on="开始测量 4" class="Bool (严格)"("Visible"=FALSE ("可见")) -> ()  [unwired: 2 in, 2 out]
            n964 = property on="开始测量 3" class="Bool (严格)"("Visible"=TRUE ("可见")) -> ()  [unwired: 2 in, 2 out]
            n965 = property on="开始测量" class="Bool (严格)"("Visible"=FALSE ("可见")) -> ()  [unwired: 2 in, 2 out]
            n966 = property on="开始测量 2" class="Bool (严格)"("Visible"=FALSE ("可见")) -> ()  [unwired: 2 in, 2 out]
          }
          frame "A4" {
            n967 = property on="开始测量 4" class="Bool (严格)"("Visible"=TRUE ("可见")) -> ()  [unwired: 2 in, 2 out]
            n968 = property on="开始测量 3" class="Bool (严格)"("Visible"=FALSE ("可见")) -> ()  [unwired: 2 in, 2 out]
            n969 = property on="开始测量" class="Bool (严格)"("Visible"=FALSE ("可见")) -> ()  [unwired: 2 in, 2 out]
            n970 = property on="开始测量 2" class="Bool (严格)"("Visible"=FALSE ("可见")) -> ()  [unwired: 2 in, 2 out]
          }
        }
      }
      event "历史曲线": Value Change {
        n971 = event-data() -> ()  [unwired: 1 in, 6 out]
        n972 = Current VI's Path() -> (path=w1263:path)
        n973 = Strip Path(path=w1263) -> (stripped path=w1264:path)  [unwired: 1 out]
        n974 = Build Path(base path=w1264, name or relative path=path "TEMPDATA" ("名称或相对路径")) -> (appended path=w1265:path)
        n975 = call "文件对话框4"("start path"=w1265) -> ("selected path"=w1261:path, "error out"=w1257:errorcluster)  [unwired: 11 in, 2 out]
        n976 = Build Path(base path=w1261, name or relative path=path "索引.txt" ("名称或相对路径")) -> (appended path=w1259:path)
        n977 = Open/Create/Replace File(file path (use dialog)=w1259, error in=w1257, operation (0:open)=T16."open" ("操作(0:open)")) -> (refnum out=w1267:refnum<file>, error out=w1266:errorcluster)  [unwired: 3 in, 1 out]
        n978 = Unbundle(w1266) -> ("status"=w1256:bool)  [unwired: 2 out]
        n979 = case shown="假" w1256 {
          tunnel: w1267 -> [w1269 _]
          tunnel: w1266 -> [w1268 _]
          frame False {
            n980 = disable-structure shown="禁用" {
              disable-tunnel: w1269 -> [w1271 _]
              disable-tunnel: w1268 -> [w1270 _]
              frame Disabled {
                n981 = flat-sequence {
                  tunnel: w1270 -> [w1277]
                  tunnel: w1271 -> [w1278]
                  tunnel: [w1278] -> w1275
                  tunnel: [w1277] -> w1274
                  tunnel: [w1281] -> w1273
                  tunnel: [w1280] -> w1272
                  tunnel: w1275 -> [w1290]
                  tunnel: w1274 -> [w1289]
                  tunnel: w1273 -> [w1312]
                  tunnel: w1272 -> [w1313]
                  frame #0 {
                    w1276 = cluster{dbl[], dbl[]} {[], []} ("XY图 2")
                  }
                  frame #1 {
                    n982 = while {
                      tunnel: w1290 -> [w1304]
                      tunnel: w1289 -> [w1303]
                      tunnel: [w1296] -> w1279 mode=indexing
                      tunnel: [w1295] -> w1285
                      stop <- w1293 stop-if-true
                      n983 = Read from Text File(file (use dialog)=w1304, count=1 ("计数"), error in=w1303) -> (refnum out=w1295:refnum<file>, text=w1300:string[], error out=w1301:errorcluster)  [unwired: 1 in, 1 out]
                      n984 = Unbundle(w1301) -> ("status"=w1294:bool)  [unwired: 2 out]
                      n985 = Index Array(array=w1300, index=0 ("索引")) -> (element=w1297:string)
                      n986 = Not Equal?(x=w1297, y="") -> (x != y?=w1292:bool)
                      n987 = case shown="假" w1292 {
                        tunnel: w1297 -> [_ w1308]
                        tunnel: [0 w1306] -> w1296
                        frame False {
                        }
                        frame True {
                          n988 = Scan From String(format string="%d" ("格式字符串"), input string=w1308) -> (output 1=w1306:i32)  [unwired: 3 in, 3 out]
                        }
                      }
                      n989 = Not(x=w1292) -> (.not. x?=w1291:bool)
                      n990 = Or(x=w1291, y=w1294) -> (x .or. y?=w1293:bool)
                    }
                    n991 = Array Size(array=w1279) -> (size(s)=w1288:i32)
                    n992 = Close File(refnum=w1285) -> (path=w1284:path)  [unwired: 1 in, 1 out]
                    n993 = Decrement(x=w1288) -> (x-1=w1286:i32)
                    n994 = Strip Path(path=w1284) -> (stripped path=w1283:path)  [unwired: 1 out]
                    n995 = Build Path(base path=w1283, name or relative path=path "数据.txt" ("名称或相对路径")) -> (appended path=w1281:path)
                    n996 = Delete From Array(array=w1279, length=1 ("长度"), index=w1286) -> (array with subset deleted=w1280:i32[])  [unwired: 1 out]
                  }
                  frame #2 {
                    n997 = Open/Create/Replace File(file path (use dialog)=w1312, operation (0:open)=T16."open" ("操作(0:open)")) -> (refnum out=w1315:refnum<file>, error out=w1316:errorcluster)  [unwired: 4 in, 1 out]
                    n998 = for {
                      tunnel: w1315 -> [w1333]
                      tunnel: w1316 -> [w1332]
                      tunnel: [w1327] -> _
                      tunnel: [w1326] -> _
                      tunnel: [w1321] -> w1311 mode=indexing
                      tunnel: [w1320] -> w1310 mode=indexing
                      tunnel: w1313 -> [w1319] mode=indexing
                      n999 = Decrement(x=w1319) -> (x-1=w1325:i32)
                      n1000 = Read from Text File(file (use dialog)=w1333, count=w1319, error in=w1332) -> (refnum out=w1331:refnum<file>, text=w1318:string[], error out=w1330:errorcluster)  [unwired: 1 in, 1 out]
                      n1001 = Index Array(array=w1318, index=w1325) -> (element=w1317:string)
                      n1002 = Set File Position(offset (in bytes) (0)=i64 0 ("偏移量（字节）（0）"), refnum=w1331, from (0:start)=enum16{"start", "end", "current"}."start" ("自（0:起始）"), error in=w1330) -> (refnum out=w1327:refnum<file>, error out=w1326:errorcluster)
                      n1003 = Search/Split String(string=w1317, search string/char (-)="电流" ("搜索字符串/字符(-)")) -> (match + rest of string=w1323:string)  [unwired: 1 in, 2 out]
                      n1004 = Scan From String(format string="电流：%f 电压：%f" ("格式字符串"), input string=w1323) -> (output 1=w1321:dbl, output 2=w1320:dbl)  [unwired: 4 in, 3 out]
                    }
                    n1005 = Bundle(w1311, w1310) -> (w1309:cluster{dbl[], dbl[]})  [unwired: 1 in]
                  }
                  frame #3 {
                  }
                }
              }
              frame Enabled {
              }
            }
          }
          frame True {
          }
        }
      }
      event "保存当前设置", "打开历史设置", "撤销当前设置": Value Change {
        n1006 = event-data() -> ("CtlRef"=w1335:refnum<vi>)  [unwired: 1 in, 3 out]
        n1007 = property class="Bool"(reference=w1335) -> ("BoolText.Text"=w1334:string)  [unwired: 1 in, 2 out]
        n1008 = property on="队列输出 2" class="TypRef (严格)" props=["Value"]() -> ()  [unwired: 2 in, 3 out]
        n1009 = case shown="\"保存设置\"" w1334 {
          frame "假", Default {
          }
          frame "保存设置" {
            n1010 = case shown="\"ALL\"" "通道选择" {
              selector: "通道选择" -> [_ w1390]
              frame "ALL" {
                n1011 = flat-sequence {
                  tunnel: [w1344] -> w1342
                  tunnel: [w1343] -> w1341
                  tunnel: w1342 -> [w1358]
                  tunnel: w1341 -> [w1357]
                  tunnel: [w1356] -> w1340
                  tunnel: [w1355] -> w1338
                  tunnel: w1340 -> [w1380]
                  tunnel: [w1375] -> w1339
                  tunnel: w1338 -> [w1379]
                  tunnel: [w1374] -> w1337
                  tunnel: w1339 -> [w1382]
                  tunnel: w1337 -> [w1381]
                  frame #0 {
                    n1012 = Current VI's Path() -> (path=w1354:path)
                    n1013 = String To Path(string="设置文件") -> (path=w1351:path)
                    n1014 = Strip Path(path=w1354) -> (stripped path=w1352:path)  [unwired: 1 out]
                    n1015 = Build Path(base path=w1352, name or relative path=w1351) -> (appended path=w1350:path)
                    n1016 = call "文件对话框"("start path"=w1350, "default name"="配置文件", "pattern (all files)"="*.ini", "pattern label"="类型文件") -> ("selected path"=w1346:path)  [unwired: 8 in, 3 out]
                    n1017 = call <vilib>:"Open Config Data.vi"("create file if necessary (T)"=TRUE, "configuration file path"=w1346) -> ("error out"=w1343:errorcluster, "refnum"=w1344:T17)  [unwired: 7 in, 1 out]
                  }
                  frame #1 {
                    n1018 = for {
                      tunnel: string[] ["A1", "A2", "A3", "A4"] -> [w1363] mode=indexing
                      tunnel: w1358 -> [w1362]
                      tunnel: w1357 -> [_]
                      tunnel: [w1361] -> w1356
                      tunnel: [w1360] -> w1355
                      i -> [w1364]
                      n1019 = property on="树形控件 2" class="Tree (严格)"() -> ("All Tags"=w1365:string[])  [unwired: 2 in, 2 out]
                      n1020 = for {
                        tunnel: w1365 -> [w1369] mode=indexing
                        tunnel: w1364 -> [w1372]
                        tunnel: w1363 -> [w1371]
                        tunnel: w1362 -> [w1370]
                        tunnel: [w1367] -> w1361
                        tunnel: [w1366] -> w1360
                        n1021 = Increment(x=w1372) -> (x+1=w1373:i32)
                        n1022 = property on="树形控件 2" class="Tree (严格)"("Active Item Tag"=w1369, "ActiveColNum"=w1373) -> ("Cell String"=w1368:string)  [unwired: 2 in, 2 out]
                        n1023 = call-poly <vilib>:"Write Key.vi"("section"=w1371, "value"=w1368, "key"=w1369, "refnum"=w1370) -> ("error out"=w1366:errorcluster, "refnum out"=w1367:T17)  [unwired: 5 in, 1 out]
                      }
                    }
                  }
                  frame #2 {
                    n1024 = call-poly <vilib>:"Write Key.vi"("section"="通道数量", "error in (no error)"=w1379, "value"="4", "key"="数量", "refnum"=w1380) -> ("error out"=w1374:errorcluster, "refnum out"=w1375:T17)  [unwired: 4 in, 1 out]
                  }
                  frame #3 {
                    n1025 = call <vilib>:"Close Config Data.vi"("error in (no error)"=w1381, "refnum"=w1382) -> ()  [unwired: 8 in, 2 out]
                  }
                }
              }
              frame "A1", Default {
                n1026 = Current VI's Path() -> (path=w1404:path)
                n1027 = String To Path(string="设置文件") -> (path=w1402:path)
                n1028 = Strip Path(path=w1404) -> (stripped path=w1403:path)  [unwired: 1 out]
                n1029 = Build Path(base path=w1403, name or relative path=w1402) -> (appended path=w1401:path)
                n1030 = call "文件对话框2"("start path"=w1401, "default name"="配置文件", "pattern (all files)"="*.ini", "pattern label"="类型文件") -> ("selected path"=w1400:path)  [unwired: 8 in, 3 out]
                n1031 = property on="树形控件 2" class="Tree (严格)"() -> ("All Tags"=w1391:string[])  [unwired: 2 in, 2 out]
                n1032 = call <vilib>:"Open Config Data.vi"("create file if necessary (T)"=TRUE, "configuration file path"=w1400) -> ("error out"=w1393:errorcluster, "refnum"=w1394:T17)  [unwired: 7 in, 1 out]
                n1033 = for {
                  tunnel: w1394 -> [w1412]
                  tunnel: w1393 -> [w1411]
                  tunnel: "通道配置" -> [w1410]
                  tunnel: w1391 -> [w1408] mode=indexing
                  tunnel: w1390 -> [w1409]
                  tunnel: [w1406] -> w1386
                  tunnel: [w1405] -> w1385
                  n1034 = property on="树形控件 2" class="Tree (严格)"("Active Item Tag"=w1408, "ActiveColNum"=w1409) -> ("Cell String"=w1407:string)  [unwired: 2 in, 2 out]
                  n1035 = call-poly <vilib>:"Write Key.vi"("section"=w1410, "error in (no error)"=w1411, "value"=w1407, "key"=w1408, "refnum"=w1412) -> ("error out"=w1405:errorcluster, "refnum out"=w1406:T17)  [unwired: 4 in, 1 out]
                }
                n1036 = call-poly <vilib>:"Write Key.vi"("section"="通道数量", "error in (no error)"=w1385, "value"="1", "key"="数量", "refnum"=w1386) -> ("error out"=w1383:errorcluster, "refnum out"=w1384:T17)  [unwired: 4 in, 1 out]
                n1037 = call <vilib>:"Close Config Data.vi"("error in (no error)"=w1383, "refnum"=w1384) -> ()  [unwired: 8 in, 2 out]
              }
            }
          }
          frame "打开设置" {
            n1038 = property on="通道选择" class="RadioBtnsControl (严格)"() -> ("Value"=w1419:enum32{"ALL", "A1", "A2", "A3", "A4"})  [unwired: 2 in, 2 out]
            n1039 = Current VI's Path() -> (path=w1433:path)
            n1040 = String To Path(string="设置文件") -> (path=w1431:path)
            n1041 = Strip Path(path=w1433) -> (stripped path=w1432:path)  [unwired: 1 out]
            n1042 = case shown="\"ALL\"" w1419 {
              tunnel: ["4" "1"] -> w1417
              frame "ALL" {
              }
              frame "A1", Default {
              }
            }
            n1043 = Build Path(base path=w1432, name or relative path=w1431) -> (appended path=w1430:path)
            n1044 = call "文件对话框5"("start path"=w1430, "default name"="配置文件", "pattern (all files)"="*.ini", "pattern label"="类型文件") -> ("selected path"=w1429:path, "error out"=w1413:errorcluster)  [unwired: 8 in, 2 out]
            n1045 = call <vilib>:"Open Config Data.vi"("create file if necessary (T)"=FALSE, "configuration file path"=w1429) -> ("error out"=w1422:errorcluster, "refnum"=w1423:T17)  [unwired: 7 in, 1 out]
            n1046 = call <vilib>:"Clear Errors.vi"("error in (no error)"=w1413) -> ()  [unwired: 5 in, 2 out]
            n1047 = call-poly <vilib>:"Read Key.vi"("section"="通道数量", "error in (no error)"=w1422, "key"="数量", "refnum"=w1423) -> ("error out"=w1414:errorcluster, "value"=w1418:string, "refnum out"=w1415:T17)  [unwired: 4 in, 1 out]
            n1048 = Equal?(x=w1418, y=w1417) -> (x = y?=w1416:bool)
            n1049 = case shown="真" w1416 {
              tunnel: w1415 -> [_ w1439]
              tunnel: w1414 -> [_ w1436]
              frame False {
                n1050 = One Button Dialog(message="配置文件通道数与通道选项不相等" ("消息"), button name ("OK")="确定" ("按钮名称（“确定”）")) -> ()  [unwired: 1 out]
              }
              frame True {
                n1051 = flat-sequence {
                  tunnel: w1439 -> [w1442]
                  tunnel: [w1442] -> w1438
                  tunnel: [w1440] -> w1437
                  tunnel: w1438 -> [w1446]
                  tunnel: w1437 -> [w1447]
                  tunnel: w1436 -> [w1445]
                  frame #0 {
                    n1052 = property on="通道选择" class="RadioBtnsControl (严格)"() -> ("Value"=w1441:enum32{"ALL", "A1", "A2", "A3", "A4"})  [unwired: 2 in, 2 out]
                    n1053 = case shown="\"A1\", 默认" w1441 {
                      tunnel: ["ALL" "通道配置"] -> w1440
                      frame "ALL" {
                      }
                      frame "A1", Default {
                      }
                    }
                  }
                  frame #1 {
                    n1054 = flat-sequence {
                      tunnel: w1447 -> [w1452]
                      tunnel: w1446 -> [w1451]
                      tunnel: w1445 -> [w1450]
                      frame #0 {
                        n1055 = case shown="\"ALL\"" w1452 {
                          selector: w1452 -> [_ w1474]
                          tunnel: w1451 -> [w1455 w1476]
                          tunnel: [w1454 w1473] -> w1449
                          tunnel: [w1453 w1472] -> w1448
                          tunnel: w1450 -> [_ w1471]
                          frame "ALL" {
                            n1056 = for {
                              tunnel: string[] ["A1", "A2", "A3", "A4"] -> [w1460] mode=indexing
                              tunnel: w1455 -> [w1461]
                              tunnel: [w1458] -> w1454
                              tunnel: [w1457] -> w1453
                              i -> [w1459]
                              n1057 = property on="树形控件 2" class="Tree (严格)"() -> ("All Tags"=w1462:string[])  [unwired: 2 in, 2 out]
                              n1058 = for {
                                tunnel: w1462 -> [w1468] mode=indexing
                                tunnel: w1461 -> [w1470]
                                tunnel: w1460 -> [w1469]
                                tunnel: w1459 -> [w1466]
                                tunnel: [w1464] -> w1458
                                tunnel: [w1463] -> w1457
                                n1059 = call-poly <vilib>:"Read Key.vi"("section"=w1469, "key"=w1468, "refnum"=w1470) -> ("error out"=w1463:errorcluster, "value"=w1465:string, "refnum out"=w1464:T17)  [unwired: 5 in, 1 out]
                                n1060 = Increment(x=w1466) -> (x+1=w1467:i32)
                                n1061 = property on="树形控件 2" class="Tree (严格)"("Active Item Tag"=w1468, "ActiveColNum"=w1467, "Cell String"=w1465) -> ()  [unwired: 2 in, 2 out]
                              }
                            }
                          }
                          frame "A1", Default {
                            n1062 = property on="树形控件 2" class="Tree (严格)"() -> ("All Tags"=w1475:string[])  [unwired: 2 in, 2 out]
                            n1063 = for {
                              tunnel: w1476 -> [w1484]
                              tunnel: w1475 -> [w1482] mode=indexing
                              tunnel: w1474 -> [w1483]
                              tunnel: [w1479] -> w1473
                              tunnel: [w1478] -> w1472
                              tunnel: w1471 -> [w1477]
                              n1064 = call-poly <vilib>:"Read Key.vi"("section"=w1483, "error in (no error)"=w1477, "key"=w1482, "refnum"=w1484) -> ("error out"=w1478:errorcluster, "value"=w1480:string, "refnum out"=w1479:T17)  [unwired: 4 in, 1 out]
                              n1065 = property on="通道选择" class="RadioBtnsControl (严格)"() -> ("Value"=w1481:enum32{"ALL", "A1", "A2", "A3", "A4"})  [unwired: 2 in, 2 out]
                              n1066 = property on="树形控件 2" class="Tree (严格)"("Active Item Tag"=w1482, "ActiveColNum"=w1481, "Cell String"=w1480) -> ()  [unwired: 2 in, 2 out]
                            }
                          }
                        }
                        n1067 = call <vilib>:"Close Config Data.vi"("error in (no error)"=w1448, "refnum"=w1449) -> ()  [unwired: 8 in, 2 out]
                      }
                      frame #1 {
                        n1068 = property on="通道选择" class="RadioBtnsControl (严格)"() -> ("Value"=w1485:enum32{"ALL", "A1", "A2", "A3", "A4"})  [unwired: 2 in, 2 out]
                        n1069 = stacked-sequence {
                          seq-local: [w1487 _ _] -> [_ _ _]
                          tunnel: w1485 -> [w1487 _ _]
                          frame #0 {
                            n1070 = property on="树形控件 2" class="Tree (严格)" props=["Active Item Tag", "ActiveColNum", "Cell String"]("Active Item Tag"="循环水温度" ("活动项:标识符"), "ActiveColNum"=w1487) -> ()  [unwired: 2 in, 3 out]
                          }
                          frame #1 {
                          }
                          frame #2 {
                          }
                        }
                      }
                    }
                  }
                }
              }
            }
          }
        }
      }
      event "保存": Value Change {
        n1071 = event-data() -> ()  [unwired: 1 in, 6 out]
        n1072 = property on="通道选择" class="RadioBtnsControl (严格)"() -> ("Value"=w1490:enum32{"ALL", "A1", "A2", "A3", "A4"})  [unwired: 2 in, 2 out]
        n1073 = disable-structure shown="禁用" {
          frame Disabled {
            n1074 = property on="树形控件 2" class="Tree (严格)" props=["Active Item Tag", "ActiveColNum", "Cell String"]() -> ()  [unwired: 4 in, 3 out]
          }
          frame Enabled {
          }
        }
        n1075 = case shown="\"A1\", 默认" w1490 {
          frame "ALL" {
          }
          frame "A1", Default {
            # "<=10℃"
            n1076 = property on="水质换水" class="DigNum (严格)"() -> ("Value"=w1549:dbl)  [unwired: 2 in, 2 out]
            n1077 = property on="氢气出口背压设定：" class="DigNum (严格)"() -> ("Value"=w1553:dbl)  [unwired: 2 in, 2 out]
            n1078 = property on="氢气出口最大压力：" class="DigNum (严格)"() -> ("Value"=w1519:dbl)  [unwired: 2 in, 2 out]
            n1079 = property on="冷却水最高温度：" class="DigNum (严格)"() -> ("Value"=w1499:dbl)  [unwired: 2 in, 2 out]
            n1080 = property on="电解槽最高温度：" class="DigNum (严格)"() -> ("Value"=w1531:dbl)  [unwired: 2 in, 2 out]
            n1081 = property on="水箱补水液位：" class="DigNum (严格)"() -> ("Value"=w1544:dbl)  [unwired: 2 in, 2 out]
            n1082 = property on="气液分离液位：" class="DigNum (严格)"() -> ("Value"=w1538:dbl)  [unwired: 2 in, 2 out]
            n1083 = property on="氢气最大露点：" class="DigNum (严格)"() -> ("Value"=w1534:dbl)  [unwired: 2 in, 2 out]
            n1084 = property on="电解槽最大电压" class="DigNum (严格)"() -> ("Value"=w1527:dbl)  [unwired: 2 in, 2 out]
            n1085 = property on="循环水最差水质" class="DigNum (严格)"() -> ("Value"=w1514:dbl)  [unwired: 2 in, 2 out]
            n1086 = property on="水箱最低液位" class="DigNum (严格)"() -> ("Value"=w1524:dbl)  [unwired: 2 in, 2 out]
            n1087 = Format Into String(format string="%.2f" ("格式字符串"), w1549) -> (resulting string=w1547:string)  [unwired: 2 in, 1 out]
            n1088 = Format Into String(format string="%d" ("格式字符串"), w1544) -> (resulting string=w1543:string)  [unwired: 2 in, 1 out]
            n1089 = Format Into String(format string="%d" ("格式字符串"), w1531) -> (resulting string=w1530:string)  [unwired: 2 in, 1 out]
            n1090 = Format Into String(format string="%d" ("格式字符串"), w1499) -> (resulting string=w1498:string)  [unwired: 2 in, 1 out]
            n1091 = Format Into String(format string="%d" ("格式字符串"), w1524) -> (resulting string=w1523:string)  [unwired: 2 in, 1 out]
            n1092 = Format Into String(format string="%.2f" ("格式字符串"), w1553) -> (resulting string=w1552:string)  [unwired: 2 in, 1 out]
            n1093 = Format Into String(format string="%.2f" ("格式字符串"), w1538) -> (resulting string=w1540:string)  [unwired: 2 in, 1 out]
            n1094 = Format Into String(format string="%.1f" ("格式字符串"), w1534) -> (resulting string=w1536:string)  [unwired: 2 in, 1 out]
            n1095 = Format Into String(format string="%.2f" ("格式字符串"), w1527) -> (resulting string=w1526:string)  [unwired: 2 in, 1 out]
            n1096 = Format Into String(format string="%.2f" ("格式字符串"), w1519) -> (resulting string=w1521:string)  [unwired: 2 in, 1 out]
            n1097 = Format Into String(format string="%.2f" ("格式字符串"), w1514) -> (resulting string=w1516:string)  [unwired: 2 in, 1 out]
            n1098 = Concatenate Strings(w1526, "V" ("字符串")) -> (w1507:string)
            n1099 = Concatenate Strings(w1530, "℃" ("字符串")) -> (w1508:string)
            n1100 = Concatenate Strings(w1498, "℃" ("字符串")) -> (w1496:string)
            n1101 = Concatenate Strings("<=" ("字符串"), w1547, "MΩ.cm" ("字符串")) -> (w1512:string)
            n1102 = Concatenate Strings(w1543, "cm" ("字符串")) -> (w1511:string)
            n1103 = Concatenate Strings(w1540, "cm" ("字符串")) -> (w1510:string)
            n1104 = Concatenate Strings("<=" ("字符串"), w1536, "℃" ("字符串")) -> (w1509:string)
            n1105 = Concatenate Strings(w1523, "cm" ("字符串")) -> (w1506:string)
            n1106 = Concatenate Strings(w1552, "MPa" ("字符串")) -> (w1513:string)
            n1107 = Concatenate Strings(w1521, "MPa" ("字符串")) -> (w1505:string)
            n1108 = Concatenate Strings(w1516, "MΩ.cm" ("字符串")) -> (w1504:string)
            n1109 = Build Array(w1513, w1512, w1511, w1510, w1509, w1508, w1507, w1496, w1506, w1505, w1504) -> (w1503:string[])
            n1110 = case shown="\"200ml/min\", 默认" "流量" {
              tunnel: ["200ml/min" "600l/min" "800l/min" "1000l/min" "1200l/min" "1400l/min" "1600l/min" "400ml/min"] -> w1556
              frame "200ml/min", Default {
              }
              frame "600ml/min" {
              }
              frame "800ml/min" {
              }
              frame "1000ml/min" {
              }
              frame "1200ml/min" {
              }
              frame "1400ml/min" {
              }
              frame "1600ml/min" {
              }
              frame "400lml/min" {
              }
            }
            n1111 = case shown="\"二线\"" "单选按钮 2" {
              tunnel: ["四线制" "二线制"] -> w1555
              frame "四线", Default {
              }
              frame "二线" {
              }
            }
            n1112 = Divide(x="温度25", y=10) -> (x/y=w1493:dbl)
            n1113 = Format Into String(format string="%d" ("格式字符串"), w1493) -> (resulting string=w1557:string)  [unwired: 2 in, 1 out]
            n1114 = property on="数据" class="Str"() -> ("Value"=w1491:string)  [unwired: 2 in, 2 out]
            n1115 = Build Array (concatenate)(w1557, w1491, w1556, w1491, w1555, w1503) -> (w1501:string[])
            n1116 = for {
              tunnel: string[] ["循环水温度", "温度控制串口", "循环水流速", "流速控制串口", "采样方式", "氢气出口背压设定", "水质换水", "水箱补水液位", "气液分离器排水液位", "氢气最大露点", "电解槽最高温度", "电解槽最大电压", "冷却水最高温度", "水箱最低液位", "氢气出口最大压力", "循环水最差水质"] -> [w1563] mode=indexing
              tunnel: w1501 -> [w1561] mode=indexing
              n1117 = property on="通道选择" class="RadioBtnsControl (严格)"() -> ("Value"=w1562:enum32{"ALL", "A1", "A2", "A3", "A4"})  [unwired: 2 in, 2 out]
              n1118 = property on="树形控件 2" class="Tree (严格)"("Active Item Tag"=w1563, "ActiveColNum"=w1562, "Cell String"=w1561) -> ()  [unwired: 2 in, 2 out]
            }
          }
        }
      }
      event "温度25": Value Change {
        n1119 = event-data() -> ("NewVal"=w1575:u16)  [unwired: 1 in, 5 out]
        n1120 = Quotient & Remainder(x=w1575, y=u16 100) -> (x-y*floor(x/y)=w1578:u16)  [unwired: 1 out]
        n1121 = Equal?(x=w1578, y=u16 0) -> (x = y?=w1576:bool)
        n1122 = case shown="假" w1576 {
          tunnel: w1575 -> [w1584 w1638]
          tunnel: w1574 -> [w1582 w1631]
          frame True {
            n1123 = flat-sequence {
              tunnel: w1582 -> [w1594]
              tunnel: [w1594] -> w1580
              tunnel: [w1595] -> w1581
              tunnel: w1580 -> [w1595]
              tunnel: [w1599] -> w1592
              tunnel: [w1598] -> w1591
              tunnel: w1581 -> [w1597]
              tunnel: w1592 -> [w1607]
              tunnel: w1591 -> [w1606]
              tunnel: [w1603] -> w1590
              tunnel: [w1602] -> w1589
              tunnel: w1590 -> [w1613]
              tunnel: w1589 -> [w1612]
              tunnel: [w1610] -> w1588
              tunnel: [w1609] -> w1587
              tunnel: w1584 -> [w1608]
              tunnel: [w1608] -> w1583
              tunnel: w1588 -> [w1623]
              tunnel: w1587 -> [w1621]
              tunnel: [w1616] -> w1586
              tunnel: [w1615] -> w1585
              tunnel: w1583 -> [w1614]
              tunnel: w1586 -> [w1625]
              tunnel: w1585 -> [w1624]
              frame #0 {
                n1124 = property on="字符串" class="Str"("Value"="0" ("字符串")) -> ()  [unwired: 2 in, 2 out]
              }
              frame #1 {
                n1125 = Wait (ms)(milliseconds to wait=u32 800 ("等待时间（毫秒）")) -> ()  [unwired: 1 out]
              }
              frame #2 {
                n1126 = call-dynamic "Write Single Holding Register.vi"("holding register value"=u16 2, "address"=u16 271, "Modbus master in"=w1597) -> ("error out"=w1598:errorcluster, "Modbus master out"=w1599:refnum<class "Modbus Master.lvclass">)  [unwired: 7 in]
              }
              frame #3 {
                n1127 = call-dynamic "Write Single Holding Register.vi"("error in (no error)"=w1606, "holding register value"=u16 9999, "address"=u16 20484, "Modbus master in"=w1607) -> ("error out"=w1602:errorcluster, "Modbus master out"=w1603:refnum<class "Modbus Master.lvclass">)  [unwired: 6 in]
              }
              frame #4 {
                n1128 = call-dynamic "Write Single Holding Register.vi"("error in (no error)"=w1612, "holding register value"=w1608, "address"=u16 20485, "Modbus master in"=w1613) -> ("error out"=w1609:errorcluster, "Modbus master out"=w1610:refnum<class "Modbus Master.lvclass">)  [unwired: 6 in]
              }
              frame #5 {
                n1129 = call-dynamic "Write Single Holding Register.vi"("error in (no error)"=w1621, "holding register value"=u16 0, "address"=u16 20488, "Modbus master in"=w1623) -> ("error out"=w1620:errorcluster, "Modbus master out"=w1622:refnum<class "Modbus Master.lvclass">)  [unwired: 6 in]
                n1130 = call-dynamic "Write Single Holding Register.vi"("error in (no error)"=w1620, "holding register value"=w1614, "address"=u16 20489, "Modbus master in"=w1622) -> ("error out"=w1615:errorcluster, "Modbus master out"=w1616:refnum<class "Modbus Master.lvclass">)  [unwired: 6 in]
              }
              frame #6 {
                n1131 = call-dynamic "Write Single Holding Register.vi"("error in (no error)"=w1624, "holding register value"=u16 0, "address"=u16 271, "Modbus master in"=w1625) -> ()  [unwired: 6 in, 2 out]
              }
              frame #7 {
                n1132 = property on="字符串" class="Str"("Value"="2" ("字符串")) -> ()  [unwired: 2 in, 2 out]
              }
              frame #8 {
                n1133 = Wait (ms)(milliseconds to wait=u32 800 ("等待时间（毫秒）")) -> ()  [unwired: 1 out]
              }
            }
          }
          frame False {
            n1134 = flat-sequence {
              tunnel: w1638 -> [w1649]
              tunnel: [w1649] -> w1637
              tunnel: [w1648] -> w1632
              tunnel: w1631 -> [w1648]
              tunnel: w1637 -> [w1651]
              tunnel: [w1651] -> w1635
              tunnel: w1632 -> [w1650]
              tunnel: [w1650] -> w1630
              tunnel: [w1656] -> w1646
              tunnel: [w1655] -> w1645
              tunnel: [w1654] -> w1636
              tunnel: w1635 -> [w1654]
              tunnel: w1630 -> [w1653]
              tunnel: w1646 -> [w1665]
              tunnel: w1645 -> [w1664]
              tunnel: [w1661] -> w1644
              tunnel: [w1660] -> w1643
              tunnel: w1636 -> [w1659]
              tunnel: [w1659] -> w1634
              tunnel: w1644 -> [w1671]
              tunnel: w1643 -> [w1670]
              tunnel: [w1668] -> w1642
              tunnel: [w1667] -> w1641
              tunnel: w1634 -> [w1666]
              tunnel: [w1666] -> w1633
              tunnel: w1642 -> [w1681]
              tunnel: w1641 -> [w1679]
              tunnel: [w1674] -> w1640
              tunnel: [w1673] -> w1639
              tunnel: w1633 -> [w1672]
              tunnel: w1640 -> [w1683]
              tunnel: w1639 -> [w1682]
              frame #0 {
                n1135 = property on="字符串" class="Str"("Value"="0" ("字符串")) -> ()  [unwired: 2 in, 2 out]
              }
              frame #1 {
                n1136 = Wait (ms)(milliseconds to wait=u32 800 ("等待时间（毫秒）")) -> ()  [unwired: 1 out]
              }
              frame #2 {
                n1137 = call-dynamic "Write Single Holding Register.vi"("holding register value"=u16 2, "address"=u16 271, "Modbus master in"=w1653) -> ("error out"=w1655:errorcluster, "Modbus master out"=w1656:refnum<class "Modbus Master.lvclass">)  [unwired: 7 in]
              }
              frame #3 {
                n1138 = call-dynamic "Write Single Holding Register.vi"("error in (no error)"=w1664, "holding register value"=u16 9999, "address"=u16 20484, "Modbus master in"=w1665) -> ("error out"=w1660:errorcluster, "Modbus master out"=w1661:refnum<class "Modbus Master.lvclass">)  [unwired: 6 in]
              }
              frame #4 {
                n1139 = call-dynamic "Write Single Holding Register.vi"("error in (no error)"=w1670, "holding register value"=w1666, "address"=u16 20485, "Modbus master in"=w1671) -> ("error out"=w1667:errorcluster, "Modbus master out"=w1668:refnum<class "Modbus Master.lvclass">)  [unwired: 6 in]
              }
              frame #5 {
                n1140 = call-dynamic "Write Single Holding Register.vi"("error in (no error)"=w1679, "holding register value"=u16 0, "address"=u16 20488, "Modbus master in"=w1681) -> ("error out"=w1678:errorcluster, "Modbus master out"=w1680:refnum<class "Modbus Master.lvclass">)  [unwired: 6 in]
                n1141 = call-dynamic "Write Single Holding Register.vi"("error in (no error)"=w1678, "holding register value"=w1672, "address"=u16 20489, "Modbus master in"=w1680) -> ("error out"=w1673:errorcluster, "Modbus master out"=w1674:refnum<class "Modbus Master.lvclass">)  [unwired: 6 in]
              }
              frame #6 {
                n1142 = call-dynamic "Write Single Holding Register.vi"("error in (no error)"=w1682, "holding register value"=u16 0, "address"=u16 271, "Modbus master in"=w1683) -> ()  [unwired: 6 in, 2 out]
              }
              frame #7 {
                n1143 = property on="字符串" class="Str"("Value"="1" ("字符串")) -> ()  [unwired: 2 in, 2 out]
              }
              frame #8 {
                n1144 = Wait (ms)(milliseconds to wait=u32 800 ("等待时间（毫秒）")) -> ()  [unwired: 1 out]
              }
            }
          }
        }
        n1145 = property on="温度25" class="Ring (严格)" props=["Value"]() -> ()  [unwired: 2 in, 3 out]
      }
      event "添加工步", "保存工步": Value Change {
        n1146 = event-data() -> ("CtlRef"=w1689:refnum<vi>)  [unwired: 1 in, 5 out]
        n1147 = property class="Bool"(reference=w1689) -> ("BoolText.Text"=w1688:string)  [unwired: 1 in, 2 out]
        n1148 = case shown="\"添加工步\"" w1688 {
          frame "假", Default {
          }
          frame "显示工步曲线" {
            n1149 = flat-sequence {
              frame #0 {
                (unwired) dbl[] []
              }
              frame #1 {
              }
              frame #2 {
                n1150 = property on="数组" class="Arr (严格)"() -> ("Value"=w1695:string[][])  [unwired: 2 in, 2 out]
                n1151 = Index Array(array=w1695, index (col)=3 ("禁用的索引 (列)")) -> (element=w1692:string[])  [unwired: 1 in]
                n1152 = Index Array(array=w1695, index (col)=5 ("禁用的索引 (列)")) -> (element=w1691:string[])  [unwired: 1 in]
                n1153 = Search 1D Array(1D array=w1692, element=" " ("元素")) -> (index of element=w1693:i32)  [unwired: 1 in]
                n1154 = for {
                  N: w1693 -> [_]
                  tunnel: w1692 -> [w1710] mode=indexing
                  tunnel: w1691 -> [w1707] mode=indexing
                  shift-right: [w1699] -> _
                  shift-left: dbl[] [] -> [w1700]
                  n1155 = Scan From String(format string="%.2f" ("格式字符串"), input string=w1710) -> (output 1=w1703:dbl)  [unwired: 3 in, 3 out]
                  n1156 = Scan From String(format string="%.2f" ("格式字符串"), input string=w1707) -> (output 1=w1706:dbl)  [unwired: 3 in, 3 out]
                  n1157 = Divide(x=w1706, y=10.0) -> (x/y=w1704:dbl)
                  n1158 = Round Toward +Infinity(x=w1704) -> (ceil(x): smallest int >= x=w1702:dbl)
                  n1159 = To Long Integer(number=w1702) -> (32bit integer=w1698:i32)
                  n1160 = Initialize Array(w1703, w1698) -> (w1701:dbl[])
                  n1161 = Build Array (concatenate)(w1700, w1701) -> (w1699:dbl[])
                }
              }
            }
          }
          frame "保存工步" {
            n1162 = Current VI's Path() -> (path=w1723:path)
            n1163 = Strip Path(path=w1723) -> (stripped path=w1722:path)  [unwired: 1 out]
            n1164 = String To Path(string="工步") -> (path=w1720:path)
            n1165 = Build Path(base path=w1722, name or relative path=w1720) -> (appended path=w1719:path)
            n1166 = call "文件对话框3"("start path"=w1719, "pattern (all files)"=".xls" ("pattern label"), "pattern label"="工步文件" ("pattern (all files)")) -> ("selected path"=w1718:path)  [unwired: 9 in, 3 out]
            n1167 = call-poly <vilib>:"Write Delimited Spreadsheet.vi"("file path (dialog if empty)"=w1718, "1D data"=string[] ["序号", "电源模式", "电压(V)", "电流(A)", "功率(W)", "运行时间(S)"]) -> ("new file path (Not A Path if cancelled)"=w1716:path, "error out"=w1715:errorcluster)  [unwired: 12 in]
            n1168 = property on="数组" class="Arr (严格)"() -> ("Value"=w1711:string[][])  [unwired: 2 in, 2 out]
            n1169 = call-poly <vilib>:"Write Delimited Spreadsheet.vi"("file path (dialog if empty)"=w1716, "2D data"=w1711, "append to file? (new file:F)"=TRUE, "error in (no error)"=w1715) -> ()  [unwired: 10 in, 2 out]
          }
          frame "添加工步" {
            n1170 = flat-sequence {
              tunnel: [w1737] -> w1727
              tunnel: [w1733] -> w1726
              tunnel: [w1729] -> w1725
              tunnel: [w1728] -> w1724
              tunnel: w1726 -> [w1755]
              tunnel: w1727 -> [w1756]
              tunnel: w1725 -> [w1754]
              tunnel: w1724 -> [w1753]
              frame #0 {
                n1171 = property on="队列输出 2" class="TypRef (严格)" props=["Value"]() -> ()  [unwired: 2 in, 3 out]
                n1172 = case shown="1" u16 1 ("Value") {
                  tunnel: ["ITECH" "TDK"] -> w1738
                  frame 0, Default {
                  }
                  frame 1 {
                  }
                }
                n1173 = property on="通道选择 2" class="RadioBtnsControl (严格)"() -> ("Value"=w1730:enum32{"未选择", "A1", "A2", "A3", "A4"})  [unwired: 2 in, 2 out]
                n1174 = Open VI Reference(type specifier VI Refnum (for type only)=refnum<vi> refnum ("类型说明符VI引用句柄（仅用于类型）"), vi path=path "C:/Users/526computer/Desktop/2022 - 副本/pem/添加工步.vi" ("VI路径"), options=128 ("选项")) -> (vi reference=w1740:refnum<vi>, error out=w1739:errorcluster)  [unwired: 3 in]
                n1175 = case shown="\"A4\"" w1730 {
                  tunnel: [w1744 w1746 w1748 w1750] -> w1729
                  tunnel: [w1743 w1745 w1747 w1749] -> w1728
                  frame "A1", Default {
                    n1176 = control-ref of="数组"() -> (w1744:refnum<vi>)
                    n1177 = property on="数组" class="Arr (严格)"() -> ("Value"=w1743:string[][])  [unwired: 2 in, 2 out]
                  }
                  frame "A2" {
                    n1178 = control-ref of="数组 10"() -> (w1746:refnum<vi>)
                    n1179 = property on="数组 10" class="Arr (严格)"() -> ("Value"=w1745:string[][])  [unwired: 2 in, 2 out]
                  }
                  frame "A3" {
                    n1180 = control-ref of="数组 11"() -> (w1748:refnum<vi>)
                    n1181 = property on="数组 11" class="Arr (严格)"() -> ("Value"=w1747:string[][])  [unwired: 2 in, 2 out]
                  }
                  frame "A4" {
                    n1182 = control-ref of="数组 12"() -> (w1750:refnum<vi>)
                    n1183 = property on="数组 12" class="Arr (严格)"() -> ("Value"=w1749:string[][])  [unwired: 2 in, 2 out]
                  }
                }
                n1184 = call-by-ref "?"(reference=w1740, error in=w1739, "字符串"=w1738, "Arr引用句柄"=w1729) -> (reference out=w1735:refnum<vi>, error out=w1737:errorcluster, "布尔"=w1733:bool)  [unwired: 9 in]
                n1185 = property on="数组 2" class="Arr (严格)"() -> ("Value"=w1736:refnum<vi>[])  [unwired: 2 in, 2 out]
                n1186 = Insert Into Array(array=w1736, new element=w1735) -> (w1734:refnum<vi>[])  [unwired: 1 in]
                n1187 = property on="数组 2" class="Arr (严格)"("Value"=w1734) -> ()  [unwired: 2 in, 2 out]
              }
              frame #1 {
                n1188 = case shown="真" w1755 {
                  tunnel: w1756 -> [_ w1760]
                  tunnel: w1754 -> [_ w1758]
                  tunnel: w1753 -> [_ w1757]
                  frame False {
                  }
                  frame True {
                    n1189 = flat-sequence {
                      tunnel: w1760 -> [w1766]
                      tunnel: [w1765] -> w1759
                      tunnel: w1758 -> [w1764]
                      tunnel: w1759 -> [w1772]
                      tunnel: [w1780] -> w1763
                      tunnel: [w1777] -> w1762
                      tunnel: [w1782] -> w1761
                      tunnel: w1757 -> [w1777]
                      tunnel: w1763 -> [w1795]
                      tunnel: w1762 -> [w1796]
                      tunnel: w1761 -> [w1797]
                      frame #0 {
                        n1190 = property class="Arr (严格)"(reference=w1764, error in=w1766) -> (error out=w1770:errorcluster, "Value"=w1768:string[][])  [unwired: 1 out]
                        n1191 = Insert Into Array(array=w1768, new element=string[] [" ", " ", " ", " ", " ", " "] ("new element/subarray")) -> (w1769:string[][])  [unwired: 2 in]
                        n1192 = property class="Arr (严格)"(reference=w1764, error in=w1770, "Value"=w1769) -> (error out=w1765:errorcluster)  [unwired: 1 out]
                      }
                      frame #1 {
                        (unwired) TRUE ("删除子项？")
                        (unwired) "A1" ("标识符")
                        n1193 = Unbundle(w1772) -> ("status"=w1776:bool, "code"=w1775:i32)  [unwired: 1 out]
                        n1194 = property on="队列输出 2" class="TypRef (严格)"() -> ("Value"=w1774:refnum<queue>)  [unwired: 2 in, 2 out]
                        n1195 = Bundle("status"=w1776, "code"=w1775, "添加工步") -> (w1771:cluster{"status":bool, "code":i32, string})  [unwired: 1 in]
                        n1196 = Enqueue Element(queue=w1774, element=w1771) -> ()  [unwired: 2 in, 3 out]
                        n1197 = call <vilib>:"Clear Errors.vi"() -> ()  [unwired: 6 in, 2 out]
                      }
                      frame #2 {
                        n1198 = Index Array(array=w1777, index (col)=1 ("索引 (行)")) -> (element=w1789:string[])  [unwired: 1 in]
                        n1199 = Index Array(array=w1777, index (row)=0 ("索引 (行)")) -> (element=w1785:string[])  [unwired: 1 in]
                        n1200 = Index Array(array=w1777, index (row)=0 ("索引 (行)")) -> (element=w1790:string[])  [unwired: 1 in]
                        n1201 = Search 1D Array(1D array=w1789, element=" ") -> (index of element=w1780:i32)  [unwired: 1 in]
                        n1202 = Index Array(array=w1790, index=4 ("索引")) -> (element=w1791:string)
                        n1203 = case shown="\"400\"" w1791 {
                          tunnel: ["ITECH" "ITECH"] -> w1782
                          frame "1700", Default {
                          }
                          frame "400" {
                          }
                        }
                        n1204 = Equal?(x=w1780, y=-1) -> (x = y?=w1778:bool)
                        n1205 = Build Array (concatenate)(w1782, w1785, "未运行") -> (w1783:string[])
                        n1206 = case shown="真" w1778 {
                          tunnel: w1783 -> [_ _]
                          frame False {
                            (unwired) 0 ("新项缩进")
                            (unwired) "A1" ("左单元格字符串")
                          }
                          frame True {
                          }
                        }
                      }
                      frame #3 {
                        n1207 = for {
                          N: w1795 -> [_]
                          tunnel: w1797 -> [w1799]
                          tunnel: w1796 -> [w1800]
                          tunnel: [w1801] -> _ mode=indexing
                          i -> [w1809]
                          n1208 = Index Array(array=w1800, index (row)=w1809) -> (element=w1798:string[])  [unwired: 1 in]
                          n1209 = Build Array (concatenate)(w1799, w1798, "未运行") -> (w1806:string[])
                          n1210 = Bundle("A1", w1806, "", 1, FALSE, 6) -> (w1801:T18)  [unwired: 1 in]
                        }
                      }
                    }
                  }
                }
              }
            }
          }
        }
      }
    }
  }
  "字符串 3" <- "测量" ("字符串 3")
  "用户：" <- "张三" ("用户：")
  "登录时间：" <- "2022-7-28:10:52:12" ("测试时间：")
  "报警信息" <- "水箱缺水" ("报警信息")
  "电流范围" <- "100A" ("电流范围")
  "电压范围" <- "10V" ("电压范围")
  "测试类型 2" <- "阶梯扫描" ("测试类型 2")
  "通讯方式" <- "LAN" ("通讯方式")
  "当前温度" <- "50" ("当前温度")
  "电源模式" <- "CC" ("电源模式")
